vi "ControlProgram6.6_10_updateFFB_3_savefittingoutput_v2.vi"() -> ()   [LabVIEW 2016]
uses:
  <vilib>/Utility/miscctls.llb/LVPoint32TypeDef.ctl
  <vilib>/Platform/TimedLoop/XDataNode/timing_clust.ctl
  <vilib>/Platform/TimedLoop/XDataNode/nitl_modes.ctl
  <vilib>/Platform/TimedLoop/XDataNode/wakeup.ctl
  <vilib>/Instr/_visa.llb/Select Event Type.ctl
  <vilib>/vision/Avi1.llb/AviRefnum.ctl
  <vilib>/Utility/error.llb/DialogType.ctl
  <vilib>/DAQmx/write.llb/DAQmx Write (Analog 1D DBL NChan 1Samp).vi
  <vilib>/DAQmx/read.llb/DAQmx Read (Analog 2D DBL NChan NSamp).vi
  <vilib>/Analysis/baseanly.llb/Mean (DBL).vi
  <vilib>/DAQmx/write.llb/DAQmx Write (Digital Bool 1Line 1Point).vi
  <vilib>/DAQmx/create/channels.llb/DAQmx Create Channel (DO-Digital Output).vi
  <vilib>/DAQmx/create/channels.llb/DAQmx Create Channel (AI-Voltage-Basic).vi
  <vilib>/DAQmx/create/channels.llb/DAQmx Create Channel (AO-Voltage-Basic).vi
  <vilib>/DAQmx/configure/timing.llb/DAQmx Timing (Sample Clock).vi
  <vilib>/DAQmx/miscellaneous.llb/DAQmx Fill In Error Info.vi
  <vilib>/Instr/_visa.llb/VISA Configure Serial Port (Instr).vi
  Arnulf--joystick/git(most_up_to_date)/Logitech-joystick/Old Trap/FAST_Global_var.vi
  <vilib>/Utility/inputDevices.llb/mouseAcquire.vi
  <vilib>/Utility/inputDevices.llb/closeMouse.vi
  <vilib>/platform/TimedLoop/XDataNode/XDataNode.xnode
  <vilib>/Platform/TimedLoop/XDataNode/XDNodeRunTimeDep.lvlib
  <resource>/objmgr/daqmx.rc
  <vilib>/Analysis/NI_AALBase.lvlib
panel:
  out "offset ffb param":T1
  in  "Save file index":i32
  out "Saving Move":bool
  out "Move time":string
  out "Primary Video Display":T2(plugin-control)
  out "Flush Sample Start Time":u32=2111292881
  out "Sample flush time (s)":dbl=48.0
  in  "Inject Sample":bool
  out "Cal values":T3={"AX alpha"=612.9626061060078, "BX alpha"=549.6584469744151, "AX kappa"=0.3485731373010688, "BX kappa"=0.3853424216291352, "AX offset"=-0.03900484438240665, "BX offset"=-0.11295550662085417, "AY alpha"=582.7562541114835, "BY alpha"=571.1587543790358, "AY kappa"=0.37498408087930674, "BY kappa"=0.36252029651198364, "AY offset"=-0.21125584642206058, "BY offset"=-0.12469077200400738}
  in  "Inject Pump 1":bool
  in  "Inject Pump 2":bool
  in  "Tab Control 2":T4(tab)
  in  "Force FB script":bool
  in  "Got ADig bead":bool
  in  "Move Cap. 2 (ADig Top)":bool
  in  "Dump beads":bool
  in  "Got DNA bead":bool
  in  "Flow on\ncap 2?":bool=TRUE
  in  "Flow on\ncap 1?":bool=TRUE
  in  "Flow on\ndump?":bool=TRUE
  in  "Raster set":i32=1
  in  "Fish After TA?":bool=TRUE
  in  "Delta after tether":dbl=1700.0
  in  "TA Cancel Save?":bool=TRUE
  in  "Min fish\ndelta (nm)":dbl=1425.0 min=0.0 max=5000.0 step=50.0
  in  "Max fish\ndelta (nm)":dbl=1900.0 min=0.0 max=5000.0 step=25.0
  in  "Fish Speed (ms)":i32=5000
  in  "Wait (ms)":i32=1500
  in  "# attempts":dbl=10.0
  in  "Cutoff force (pN)":dbl=4.5
  in  "Raster after\n tether?":bool=TRUE
  out "Tether":bool
  out "Attempt #":i32
  in  "Flow on\nwhile fish?":bool=TRUE
  in  "Flow on\nafter raster?":bool=TRUE
  in  "Offset raster set":i32
  in  "Offset @ Delta (nm)":dbl=1700.0
  in  "Cal @ Delta (nm)":dbl=2500.0
  in  "Cal stage position":i32=3
  out "Cal Final Sampling Rate":dbl=125000.0
  in  "Cal Averaging":i32=1
  in  "Wait before dip (s)":dbl=3.0
  in  "Start dipping after?":bool
  in  "Start trap delta (nm)":dbl=1700.0
  in  "Repeat Dip":bool
  out "Dip #":i32
  in  "Dip attempts":dbl=3.0
  in  "Cancel Rep\n Dip":bool
  out "Return elasped time":i32
  in  "Return duration":dbl=15.0
  in  "Cancel dwell":bool=TRUE
  in  "Pause dwell":bool
  in  "Start/Return position":dbl=3.0
  in  "Dip duration":dbl=15.0
  in  "Dip position":dbl=4.0
  in  "Dip":bool
  out "Dip elasped time":i32
  in  "Stop":bool=TRUE
  in  "?":T5(tab)
  out "FAST X-Y":bool
  out "FAST Z":bool
  in  "Cal time (s)":dbl=5.0
  in  "Save N sets":bool
  in  "N sets":i32=200
  out "Cal sets to save":i32=500
  in  "Reset data stream":bool
  out "Buffer Overflow":bool
  out "Stage moving":bool
  in  "Comment":string
  in  "Raster scan":bool
  out "Saving":bool
  in  "Save cal":bool
  in  "Save Data":bool
  in  "Stop saving":bool
  out "Calibrating":bool
  out "Progress":dbl(slide) scale=0.0..100.0
  in  "Read Cal":bool
  in  "Fish":bool
  in  "Averaging Number":i32=1250
  out "Final Sampling Rate":dbl=100.0
  in  "Trap position (V)":cluster{"X":dbl, "Y":dbl}={"X"=3.9042624789680316, "Y"=0.2}
  in  "Trap delta (nm)":dbl=2500.0 min=0.0 max=5000.0 step=50.0
  in  "Fixed X":dbl=1.1
  in  "Fixed Y":dbl=0.15
  in  "Shutter 1 (B)":bool
  in  "Shutter 2 (A)":bool
  in  "Pulling direction":bool
  out "Raster scanning...":bool
  out "Current file name":path=path "D:/data/160111/160111_006.dat"
  in  "AX alpha":dbl=612.9626061060078 format="%#_3p"
  in  "BX alpha":dbl=549.6584469744151 format="%#_3g"
  in  "AX kappa":dbl=0.3485731373010688 format="%#_3g"
  in  "BX kappa":dbl=0.3853424216291352 format="%#_3g"
  in  "AX offset":dbl=-0.03900484438240665 format="%#_3g"
  in  "BX offset":dbl=-0.11295550662085417 format="%#_3g"
  in  "AY alpha":dbl=582.7562541114835 format="%#_3g"
  in  "BY alpha":dbl=571.1587543790358 format="%#_3g"
  in  "AY kappa":dbl=0.37498408087930674 format="%#_3g"
  in  "BY kappa":dbl=0.36252029651198364 format="%#_3g"
  in  "AY offset":dbl=-0.21125584642206058 format="%#_3g"
  in  "BY offset":dbl=-0.12469077200400738 format="%#_3g"
  out "Buffer status":u8(slide) scale=0.0..100.0
  in  "Target":bool
  in  "Default data save Avg Num":i32=1250
  in  "dump spot 2":string="Dump beads spot"
  in  "Move to Position 6":bool
  in  "Set Position 6":bool
  in  "Set Current\nPos to (0,0,0)":bool
  in  "dump spot":string="Dump beads spot"
  in  "up flow spot":string="Upper flow spot"
  in  "low flow spot":string="Lower flow spot"
  in  "up cap":string="Upper capillary (ADig beads)"
  in  "bottom cap":string="Lower capillary (DNA beads)"
  in  "Move to Position 5":bool
  in  "Set Position 5":bool
  in  "Saved stage positions":dbl[][](array[numeric])=[[1.0, 0.0, 0.0, 0.0], [2.0, -0.13716, -3.21132, 0.01436], [3.0, 0.45, -0.73974, 0.005], [4.0, 0.45, -2.1978, 0.005], [5.0, 0.45, -2.63158, -0.02256]]
  in  "Set Position 2":bool
  in  "Move to Position 2":bool
  in  "Set Position 1":bool
  in  "Move to Position 1":bool
  in  "Set Position 4":bool
  in  "Move to Position 4":bool
  in  "Set Position 3":bool
  in  "Move to Position 3":bool
  out "Stage error":errorcluster
  in  "Clear Volume":bool
  out "Sample Flush Meter":u8(slide) scale=0.0..100.0
  out "Flushing Sample":bool
  in  "Flush Sample":bool
  in  "Normal \nRate (ul/hr)  3":dbl=100.0
  in  "Normal \nVolume (ul) 3":dbl=250.0
  in  "Normal \nVolume (ul) 2":dbl
  in  "Normal \nRate (ul/hr)":dbl
  in  "Normal \nVolume (ul)":dbl
  in  "Flush\nRate (ul/min)":dbl
  in  "Flush\nVolume (ul)":dbl
  in  "Flush \nRate (ul/min)  2":dbl
  in  "Flush Pump 2":bool
  in  "Flush\nVolume (ul)  2":dbl
  in  "Flush Pump 1":bool
  in  "Normal \nRate (ul/hr)  2":dbl
  in  "Write Wait":i32=1000
  in  "Flush \nRate (ul/min)  3":dbl=100.0
  in  "Flush\nVolume (ul)  3":dbl=80.0
  out "error out":errorcluster
  in  "Use Mouse to Move Trap?":bool
  in  "Pause Mouse/Mirror Connection":bool
  out "Reference Voltage":cluster{dbl, dbl}={0.0, -0.0}
  out "Saved voltage":cluster{dbl, dbl}={5.766666666666665, 1.45}
  out "Real Coordinates":cluster{"Horizontal":i32, "Vertical":i32}={"Horizontal"=897, "Vertical"=-1271}
  out "CoordinatesMousePressed":T6
  in  "reset offset ffb param":bool
  in  "Read \nOffset FFB param":bool
  in  "Force Feedback 2":bool
  in  "Offset 2":cluster{"Off Y":dbl, "Off X":dbl}={"Off Y"=1.5, "Off X"=0.17}
  in  "Setpoint voltage 2":cluster{"SP Y":dbl, "SP X":dbl}={"SP Y"=0.6, "SP X"=0.0}
  out "Sum error":dbl(knob) scale=-0.2..0.2
  out "Trap sep":waveform(dbl)[](graph)=[{"t0"=timestamp(4.489999999999949 s since 1904-01-01), "dt"=0.002, "Y"=[-1157.7639781743756, -1157.678951177374, -1157.7582331070425, -1157.7490409992681, -1157.8995617642552], "attributes"=variant("NI_ChannelName"=variant(string "T2 X"))}, {"t0"=timestamp(4.489999999999949 s since 1904-01-01), "dt"=0.002, "Y"=[-909.0775466981794, -909.1316439023619, -909.1322956759037, -909.1570630705896, -909.1264297140281], "attributes"=variant("NI_ChannelName"=variant(string "T2 Y"))}]
  in  "Set reading to\nsetpoint 1":bool
  in  "Offset Y (nm)":dbl format="%0.2f"
  in  "Offset X (nm)":dbl format="%0.2f"
  in  "Remove offsets":bool
  in  "Force Feedback 1":bool
  out "Feedback Output \nVoltage 2":cluster{dbl, dbl} {"?" format="%#_4g"; "?" format="%#_4g"}
  in  "Offset 1":cluster{"Off Y":dbl, "Off X":dbl}={"Off Y"=1.5, "Off X"=0.17}
  in  "Setpoint voltage 1":cluster{"SP Y":dbl, "SP X":dbl}={"SP Y"=0.6, "SP X"=0.0}
  in  "Feedback const":T7={"Ki_B_Y"=0.5, "Ki_B_X"=0.0, "Kp Y"=1.0, "Kp X"=0.0}
  out "Mean Trap Pos X 2 (nm)":dbl=-1157.769953044463 format="%0.2f"
  out "Mean Trp Pos Y 2 (nm)":dbl=-909.1249958122125 format="%0.2f"
  out "T2 X RMS (A)":dbl=0.7168002469275427 format="%0.2f"
  out "T2 Y RMS (A)":dbl=0.25997187037503383 format="%0.2f"
  in  "Set reading to\nsetpoint 2":bool
  out "offset fit ffb output":cluster{dbl, dbl} {"?" format="%#_4g"; "?" format="%#_4g"}
  in  "Scan range (nm)":dbl=425.0
  in  "Scan speed (nm/s)":dbl=100.0 min=0.0 max=100.0
  in  "Step size (nm)":dbl=1.0
  in  "Save scans":bool=TRUE
  in  "# scans":i32=1
  in  "Load param":bool
  in  "Scan Parameters":T8(array[cluster])
  in  "Trap delta\nafter (nm)":dbl=1550.0
  in  "Stop raster":bool
  out "Scan range (V)":dbl=0.47672462142456534
  out "Scan steps (mirror)":u64=425
  out "Scan increment (V)":dbl=0.0011217049915872126
  out "Time per step (ms)":dbl=10.0
  out "Total raster time (s)":dbl=8.5
  out "N sets to be saved":dbl=850.0
  out "moveX":string
  out "moveY":string
  in  "Grid Movable Trap":bool
  in  "take fixed bead\n Images":bool
  in  "Zoom Factor":sgl=7.0
  in  "Center Point":cluster{"X":i32, "Y":i32}={"X"=335, "Y"=271}
  in  "Intensity Upper":dbl=88.0
  in  "Intensity Lower":dbl=66.0
  out "Window Size":cluster{"Height":i32, "Width":i32}
  in  "Image Index":dbl=1.0 min=1.0
  in  "Save Image":bool
  in  "Averaging":bool
  in  "Reset Averaging":bool
  in  "Save Video":bool
  in  "New Video File":bool
  in  "Video Index":dbl=1.0 min=1.0 step=1.0
  in  "Video Capture Rate (Hz)":dbl=30.0
  in  "Initial Window Size":cluster{"Width":i32, "Height":i32}={"Width"=884, "Height"=619}
  in  "Initial Window Position":cluster{"X Position":i32, "Y Position":i32}={"X Position"=796, "Y Position"=4}
  out "Window Position":cluster{"X Position":i32, "Y Position":i32}={"X Position"=40, "Y Position"=40}
  out "Path Out":path
  in  "Target coordinates":cluster{"X1":dbl, "Y1":dbl, "X2":dbl, "Y2":dbl}={"X1"=328.0, "Y1"=274.0, "X2"=368.0, "Y2"=314.0}
  out "image8bitArray":u8[][](array[numeric])
  out "GreyscaleArray":u32[](array[numeric])
  in  "take background images":bool
  in  "# Samples/channel (in)":i32=40000 format="%.2f"
  out "Buffer size\n(Samples/channel)":u32=511
  out "DAQ rate\n(Samples/s)":dbl=125000.0 format="%#_6p"
  out "# Samples/channel":i32=1250
  out "# Samples/channel/s":dbl=100.0
  out "AvailSampPerChan":u32=9
  out "Data update period (s/set)":dbl=0.01 format="%#_6p"
  out "AvailSampPerChan 2":u32=110
  in  "PC samp per channel":i32=1000
  in  "Sampling Rate":dbl=125000.0 format="%0.0p"
  in  "DAQ Rate2":dbl=1000000.0 format="%#_6p"
  out "Data period (s)":dbl=8e-06 format="%#_6p"
  in  "Save user params":bool
  in  "User":string(combo)
  in  "Load user params":bool
  in  "Tether break\nforce (pN)":dbl=1.0
  in  "Path":path=path "E:/Data"
  out "Mirror task":refnum<k21>
  in  "Conv X (nm/V)":dbl=891.5
  in  "Conv Y (nm/V)":dbl=505.7
  in  "Min value Y":dbl format="%.1g"
  in  "Max value Y":dbl=10.0 format="%.1f"
  in  "Min value X":dbl format="%0.1f"
  in  "Max value X":dbl=10.0 format="%.1f"
  in  "HWP1":string="Half waveplate 1: differential trap power"
  in  "HWP0":string="Half waveplate 0: total trap power"
  in  "Move 1":bool
  in  "\"Degrees\" 1":dbl
  in  "Move 0":bool
  in  "\"Degrees\" 0":dbl
  in  "Y command":enum16{"Fish", "Dump", "Got ADig", "Got DNA"}(ring)
  in  "B command":enum16{"Got DNA", "Got ADig", "Dump", "Fish"}(ring)
  in  "A command":enum16{"Got ADig", "Dump", "Fish", "Got DNA"}(ring)
  in  "X command":enum16{"Dump", "Fish", "Got ADig", "Got DNA"}(ring)
  out "Logitech":bool
  out "START":bool
  out "BACK":bool
  out "Right stick button":bool
  out "Left Y":i8(slide) scale=-128.0..127.0
  out "Left X":i8(slide) scale=-128.0..127.0
  out "Right Y":i8(slide) scale=-128.0..127.0
  out "Right X":i8(slide) scale=-128.0..127.0
  out "X":bool
  out "Y":bool
  out "A":bool
  out "B":bool
  out "RB":bool
  out "LB":bool
  out "R":bool
  out "L":bool
  out "D":bool
  out "U":bool
  out "Left stick button":bool
  out "FAST Z":bool
  out "FAST X-Y":bool
  in  "XY Speed Definitions":T9={"Slow X velocity input"="0.05", "Slow Y velocity input"="0.05", "Fast1 X velocity input"="0.1", "Fast1 Y velocity input"="0.1", "Fast2 X velocity input"="0.2", "Fast2 Y velocity input"="0.2"}
  in  "Z Speed Definitions":cluster{"Slow Z":string, "Fast Z":string}={"Slow Z"="0.025", "Fast Z"="0.05"}
  in  "Z Wait time":string="120"
  in  "X-Y Wait time":string="125"
  in  "USB port":refnum<visa-resource-name>="USB0::0x046D::0xC21D::CC66247B::RAW"
  out "Deflection":T6
  in  "Sampling Rate":dbl=125000.0 format="%0.2f"
  in  "Averaging Number":i32=12500
  in  "DAQ Rate":dbl=1000000.0
  out "Final Sampling Rate":dbl
  in  "Tab Control":T10(tab)
  in  "Downsamp\nfact":dbl=250.0
  out "Bead sep":waveform(dbl)[](graph)=[{"t0"=timestamp(4.489999999999949 s since 1904-01-01), "dt"=0.002, "Y"=[8093.963535945606, 8103.1617772716045, 8385.72390184118, 8245.733099167523, 8154.925676756515], "attributes"=variant("NI_ChannelName"=variant(string "T2"))}, {"t0"=timestamp(4.489999999999949 s since 1904-01-01), "dt"=0.002, "Y"=[1717.924930434114, 1628.723007842151, 1787.6888378897193, 1598.475730715916, 1776.2517588078954], "attributes"=variant("NI_ChannelName"=variant(string "T1"))}]
  out "Force (pN)":waveform(dbl)[](graph)=[{"t0"=timestamp(4.489999999999949 s since 1904-01-01), "dt"=0.002, "Y"=[2821.5994183803123, 2824.8226375853515, 2923.3663028678166, 2874.5254578927593, 2842.869034836209], "attributes"=variant("NI_ChannelName"=variant(string "T2"))}, {"t0"=timestamp(4.489999999999949 s since 1904-01-01), "dt"=0.002, "Y"=[623.5850847499229, 591.0680427774053, 648.761979867749, 579.944408346982, 644.7436619059413], "attributes"=variant("NI_ChannelName"=variant(string "T1"))}]
  out "Mean force (pN)":dbl=1737.5286029210451 format="%0.2f"
  out "Force noise (pN)":dbl=26.83032703631318 format="%0.2f"
  out "Mean Bead Sep\n(nm)":dbl=4949.257225667222 format="%0.2f"
  out "Bead Sep Noise\n(A)":dbl=757.8078481959694 format="%0.2f"
  out "PSD 2":cluster{dbl[], dbl[]}(graph)
  out "PSD 1":cluster{dbl[], dbl[]}(graph)
  out "PSD 1 Sum":dbl(slide) scale=0.0..10.0
  out "PSD 2 Sum":dbl(slide) scale=0.0..10.0
  in  "Start":bool
  out "All signals 2":waveform(dbl)[](graph)=[{"t0"=timestamp(4.489999999999949 s since 1904-01-01), "dt"=0.002, "Y"=[0.0010396217068286443, 0.0010666908927528754, 0.001103298744846499, 0.0010651440823993424, 0.0010656596859401936], "attributes"=variant("NI_ChannelName"=variant(string "A y"))}, {"t0"=timestamp(4.489999999999949 s since 1904-01-01), "dt"=0.002, "Y"=[0.02000680227246931, 0.020097032918054827, 0.02003412926844257, 0.020136734401221615, 0.020087494249822452], "attributes"=variant("NI_ChannelName"=variant(string "A x"))}, {"t0"=timestamp(4.489999999999949 s since 1904-01-01), "dt"=0.002, "Y"=[-0.0014958587831537804, -0.0015046240440107857, -0.0014930229638311983, -0.001533240041751485, -0.0015262793936602433], "attributes"=variant("NI_ChannelName"=variant(string "B y"))}, {"t0"=timestamp(4.489999999999949 s since 1904-01-01), "dt"=0.002, "Y"=[0.0002901198559372817, 0.0002731049385577592, 0.00026511308349727467, 0.0002517073909711183, 0.0002916666665966012], "attributes"=variant("NI_ChannelName"=variant(string "B x"))}, {"t0"=timestamp(4.489999999999949 s since 1904-01-01), "dt"=0.002, "Y"=[-0.001511556786147372, -0.0015167122027053212, -0.0014612914746018214, -0.0014935128282145193, -0.0015064013696263116], "attributes"=variant("NI_ChannelName"=variant(string "A sum"))}, {"t0"=timestamp(4.489999999999949 s since 1904-01-01), "dt"=0.002, "Y"=[-0.0005242945138364382, -0.0005565158674093218, -0.000501095139248956, -0.0005771375336978897, -0.0005165613890095197], "attributes"=variant("NI_ChannelName"=variant(string "B sum"))}, {"t0"=timestamp(4.489999999999949 s since 1904-01-01), "dt"=0.002, "Y"=[0.0013303666019343777, 0.0014257418088905328, 0.0013368108726387405, 0.0013471217058124534, 0.0011782818123890176], "attributes"=variant("NI_ChannelName"=variant(string "Trap x"))}, {"t0"=timestamp(4.489999999999949 s since 1904-01-01), "dt"=0.002, "Y"=[0.0023382505474007294, 0.002231275652833831, 0.002229986798687363, 0.0021810103409340116, 0.002241586486003531], "attributes"=variant("NI_ChannelName"=variant(string "Trap y"))}]
  out "All signals":waveform(dbl)[](graph)=[{"t0"=timestamp(4.489999999999949 s since 1904-01-01), "dt"=0.002, "Y"=[0.0010396217068286443, 0.0010666908927528754, 0.001103298744846499, 0.0010651440823993424, 0.0010656596859401936], "attributes"=variant("NI_ChannelName"=variant(string "A y"))}, {"t0"=timestamp(4.489999999999949 s since 1904-01-01), "dt"=0.002, "Y"=[0.02000680227246931, 0.020097032918054827, 0.02003412926844257, 0.020136734401221615, 0.020087494249822452], "attributes"=variant("NI_ChannelName"=variant(string "A x"))}, {"t0"=timestamp(4.489999999999949 s since 1904-01-01), "dt"=0.002, "Y"=[-0.0014958587831537804, -0.0015046240440107857, -0.0014930229638311983, -0.001533240041751485, -0.0015262793936602433], "attributes"=variant("NI_ChannelName"=variant(string "B y"))}, {"t0"=timestamp(4.489999999999949 s since 1904-01-01), "dt"=0.002, "Y"=[0.0002901198559372817, 0.0002731049385577592, 0.00026511308349727467, 0.0002517073909711183, 0.0002916666665966012], "attributes"=variant("NI_ChannelName"=variant(string "B x"))}, {"t0"=timestamp(4.489999999999949 s since 1904-01-01), "dt"=0.002, "Y"=[-0.001511556786147372, -0.0015167122027053212, -0.0014612914746018214, -0.0014935128282145193, -0.0015064013696263116], "attributes"=variant("NI_ChannelName"=variant(string "A sum"))}, {"t0"=timestamp(4.489999999999949 s since 1904-01-01), "dt"=0.002, "Y"=[-0.0005242945138364382, -0.0005565158674093218, -0.000501095139248956, -0.0005771375336978897, -0.0005165613890095197], "attributes"=variant("NI_ChannelName"=variant(string "B sum"))}, {"t0"=timestamp(4.489999999999949 s since 1904-01-01), "dt"=0.002, "Y"=[0.0013303666019343777, 0.0014257418088905328, 0.0013368108726387405, 0.0013471217058124534, 0.0011782818123890176], "attributes"=variant("NI_ChannelName"=variant(string "Trap x"))}, {"t0"=timestamp(4.489999999999949 s since 1904-01-01), "dt"=0.002, "Y"=[0.0023382505474007294, 0.002231275652833831, 0.002229986798687363, 0.0021810103409340116, 0.002241586486003531], "attributes"=variant("NI_ChannelName"=variant(string "Trap y"))}]
  out "Chart Freq (Hz)":dbl=500.0
  # "Bead Calibration"
  # "Y"
  # "X"
  # "Pump #1 Controls"
  # "Pump #2 Controls"
  # "Sample Pump Controls"
  # "Retract the pumps manually. Change it back to INFUSE when you're done. Suck it up, don't whine."
  # "Shutter 1 (B)"
  # "Move to Lower Cap"
  # "Inject Sample"
  # "Move to Upper Cap"
  # "Shutter 2 (A)"
  # "Select the Joystick input:"
  # "Overflow happens when >40 commands\nsent in 5 seconds. Then 4 consecutive beeps."
  # "Try increasing wait time to reduce 'following error threshold exceeded' occurances."
  # "Left stick controls Z axis.\nRight on stick: neg Z-dir\nUp on stick: neg Z-dir"
  # "Toggles FAST Z"
  # "Toggles FAST X-Y"
  # "The default Newport max velocity is 0.4"
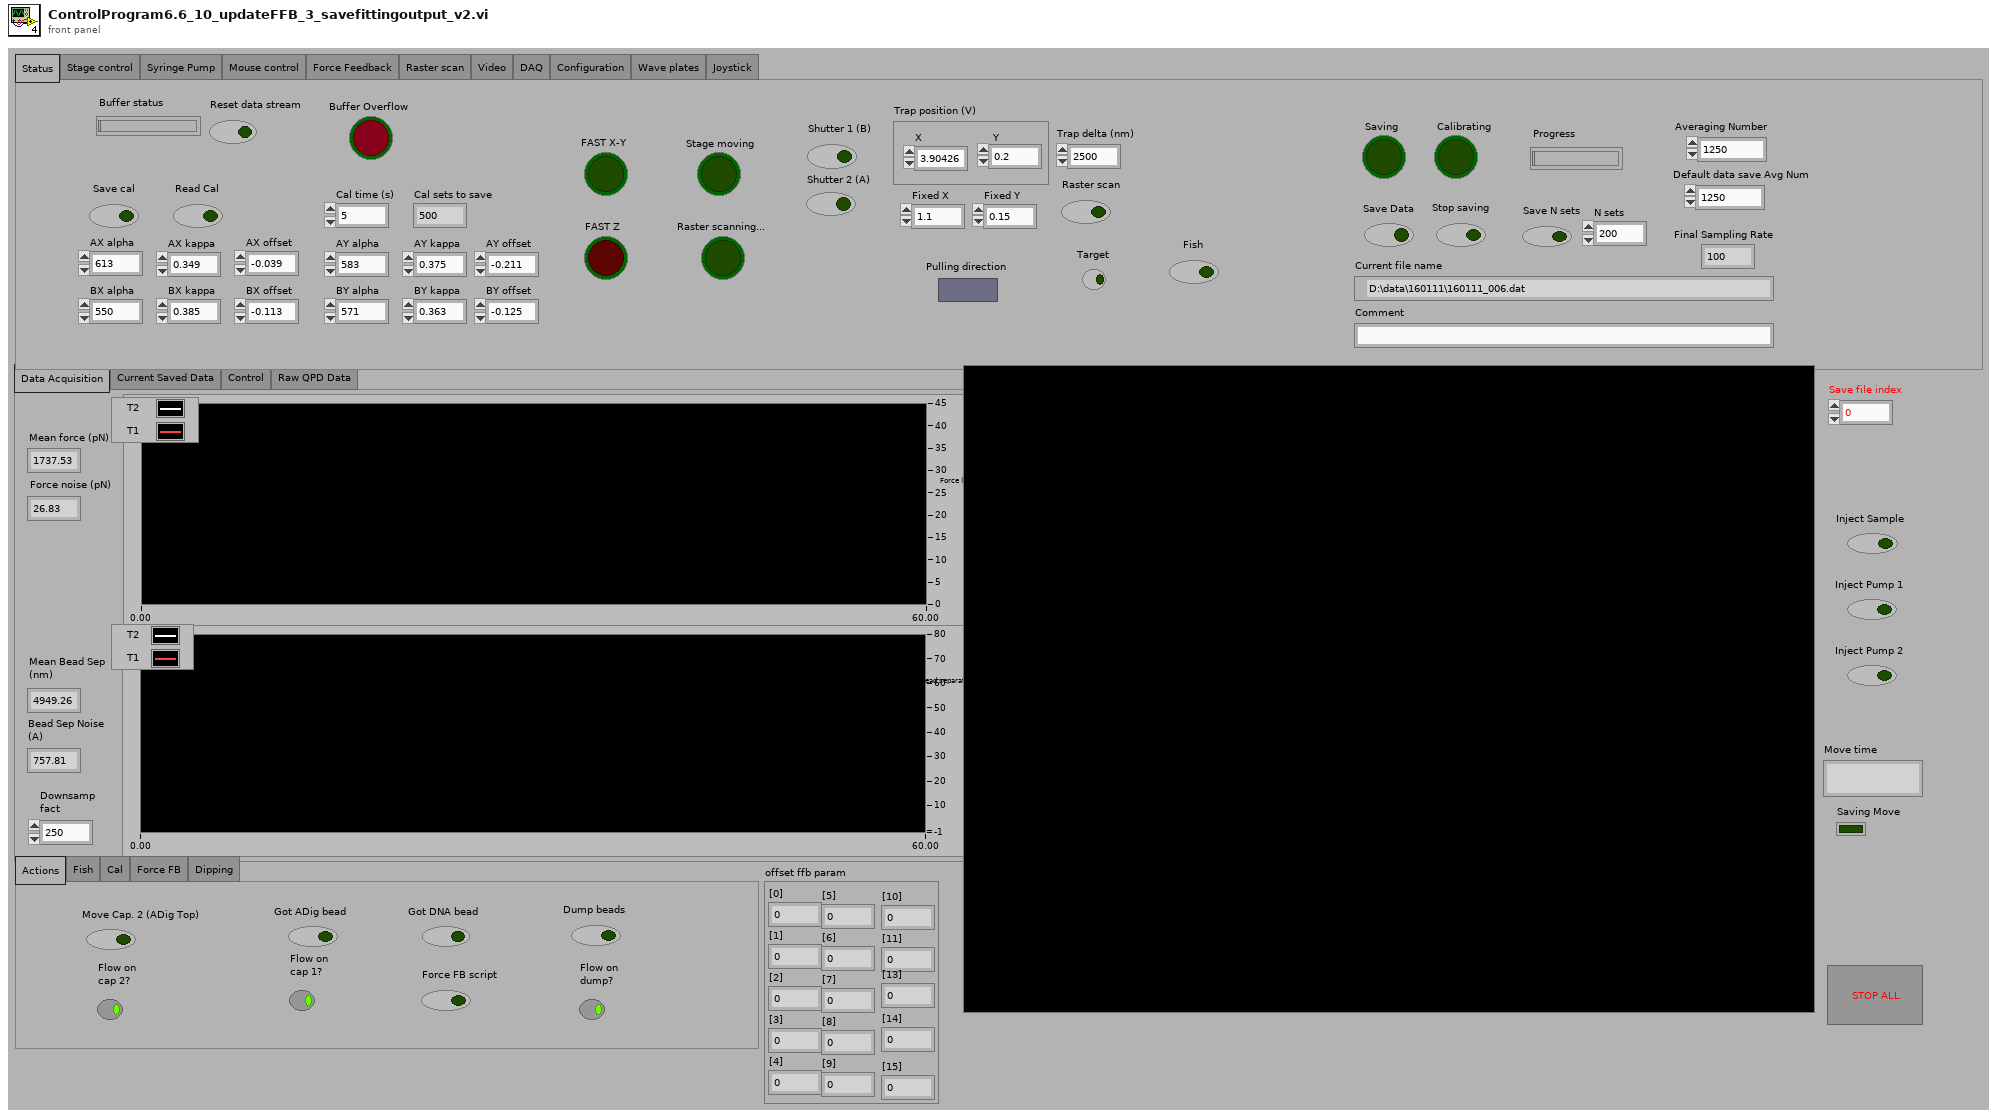
[diagram p1: front panel]
types:
  T1 = cluster{"[0]":dbl, "[1]":dbl, "[2]":dbl, "[3]":dbl, "[4]":dbl, "[5]":dbl, "[6]":dbl, "[7]":dbl, "[8]":dbl, "[9]":dbl, "[10]":dbl, "[11]":dbl, "[13]":dbl, "[14]":dbl, "[15]":dbl}
  T2 = typedef "IMAQ Image.ctl" = refnum<image>
  T3 = cluster{"AX alpha":dbl, "BX alpha":dbl, "AX kappa":dbl, "BX kappa":dbl, "AX offset":dbl, "BX offset":dbl, "AY alpha":dbl, "BY alpha":dbl, "AY kappa":dbl, "BY kappa":dbl, "AY offset":dbl, "BY offset":dbl}
  T4 = enum32{"Actions", "Fish", "Cal", "Force FB", "Dipping"}
  T5 = enum32{"Status", "Stage control", "Syringe Pump", "Mouse control", "Force Feedback", "Raster scan", "Video", "DAQ", "Configuration", "Wave plates", "Joystick"}
  T6 = typedef "LVPoint32TypeDef.ctl" = cluster{"Horizontal":i32, "Vertical":i32}
  T7 = cluster{"Ki_B_Y":dbl, "Ki_B_X":dbl, "Kp Y":dbl, "Kp X":dbl}
  T8 = cluster{"Label":string, "Scan range 1":dbl, "Step size 1":dbl, "Scan speed 1":i32, "# scans 2":i32}[]
  T9 = cluster{"Slow X velocity input":string, "Slow Y velocity input":string, "Fast1 X velocity input":string, "Fast1 Y velocity input":string, "Fast2 X velocity input":string, "Fast2 Y velocity input":string}
  T10 = enum32{"Data Acquisition", "Current Saved Data", "Control", "Raw QPD Data"}
  T11 = typedef "Select Event Type.ctl" = u32
  T12 = enum32{"setting", "request", "request control", "info", "statistics", "system settings", "I/O sub system", "HRT control", "camera descriptions", "device specific data", "event sub system settings", "event sub system results", "image memory manager"}
  T13 = typedef "AviRefnum.ctl" = refnum<k1>
  T14 = typedef "XDNodeRunTimeDep.lvlib/timing_clust.ctl" = cluster{"Expected End [f-1]":u64, "Actual End [f-1]":u64, "Finished Late? [f-1]":bool, "Expected End [i-1]":u64, "Actual End [i-1]":u64, "Finished Late? [i-1]":bool, "Expected Start [i]":u64, "Actual Start [i]":u64, "Expected Start [f]":u64, "Actual Start [f]":u64, "Source Name":string, "Structure Name":string, "Period":i64, "Deadline":i64, "Offset":i64, "Start":i64, "Priority":i32, "Timeout":i32, "Mode":T15, "Wakeup Reason":T16, "Error":errorcluster, "Source Type":string, "Secondary Source Type":string, "Global End Time":u64, "Global Start Time":u64, "Frame Duration":u64, "Iteration Duration":u64, "Assigned CPU":i32, "I/O Scan Engine Mode":u32}
  T15 = typedef "XDNodeRunTimeDep.lvlib/nitl_modes.ctl" = enum32{"No Change", "Process missed periods, maintain original phase", "Discard missed periods, maintain original phase", "Process missed periods, ignore original phase", "Discard missed periods, ignore original phase"}
  T16 = typedef "XDNodeRunTimeDep.lvlib/wakeup.ctl" = enum32{"Normal", "Aborted", "Asynchronous wakeup", "Timing source error", "Timed loop error", "Timeout"}
  T17 = typedef "Image Type" = u32
  T18 = typedef "imagedata.ctl" = cluster{"image type":i32, "image depth":i32, "image":u8[], "mask":u8[], "colors":u32[], "Rectangle":cluster{"left":i16, "top":i16, "right":i16, "bottom":i16}}
  T19 = enum16{"open", "replace", "create", "open or create", "replace or create", "replace or create with confirmation"}
  T20 = enum16{"big-endian, network order", "native, host order", "little-endian"}
  T21 = cluster{string, string, string, string, string, string, string, string}
  T22 = cluster{"LB":bool, "RB":bool, "BACK":bool, "Logitech":bool, "START":bool}
  T23 = cluster{"Right X":i8, "Right Y":i8, "Left X":i8, "Left Y":i8}
  T24 = enum32{"Status", "Stage control", "Syringe Pump", "Mouse control", "Force Feedback", "Raster scan", "Video", "DAQ", "Configuration", "Wave plates"}
  T25 = typedef "DialogType.ctl" = u16
  T26 = cluster{"button 1":bool, "button 2":bool, "button 3":bool, "button 4":bool}
  T27 = cluster{"[0]":dbl, "[1]":dbl, "[2]":dbl, "[3]":dbl, "[4]":dbl, "[5]":dbl, "[6]":dbl, "[7]":dbl, "[8]":dbl, "[9]":dbl, "[10]":dbl, "[11]":dbl}
  T28 = cluster{"[0]":dbl, "[1]":dbl, "[2]":dbl, "[3]":dbl, "[4]":dbl, "[5]":dbl, "[6]":dbl, "[7]":dbl, "[8]":dbl, "[9]":dbl, "[10]":dbl, "[11]":dbl, "[12]":dbl, "[13]":dbl, "[14]":dbl}
  T29 = cluster{"array[0]":dbl, "array[1]":dbl, "array[2]":dbl, "array[3]":dbl, "array[4]":dbl, "array[5]":dbl, "array[6]":dbl, "array[7]":dbl, "array[8]":dbl, "array[9]":dbl, "array[10]":dbl, "array[11]":dbl, "array[12]":dbl, "array[13]":dbl, "array[14]":dbl}
  T30 = cluster{"Label":string, "Scan range 1":dbl, "Step size 1":dbl, "Scan speed 1":i32, "# scans 2":i32}
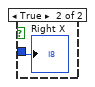
[diagram p5: hidden frame]
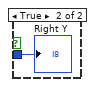
[diagram p6: hidden frame]
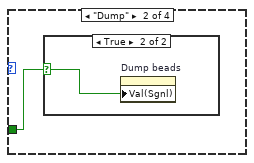
[diagram p10: hidden frame]
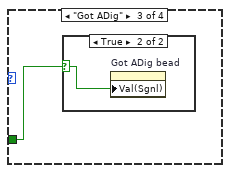
[diagram p12: hidden frame]
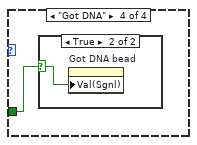
[diagram p14: hidden frame]
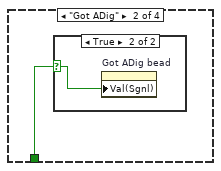
[diagram p17: hidden frame]
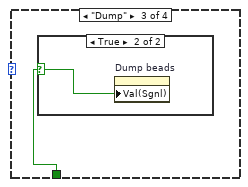
[diagram p19: hidden frame]
diagram:
  w10 = T11 1073684535 items=["Service Request"=1073684491, "Trigger"=3221168138, "Clear"=1073684493, "VXI Signal"=1073684512, "VXI/VME Interrupt"=3221168161, "VXI/VME Sysfail"=1073684509, "VXI/VME Sysreset"=1073684510, "GPIB CIC"=1073684498, "GPIB Talk"=1073684499, "GPIB Listen"=1073684500, "PXI Interrupt"=1073684514, "Serial Break"=1073684515, "Serial TermChar"=1073684516, "Serial CTS"=1073684521, "Serial DSR"=1073684522, "Serial DCD"=1073684524, "Serial RI"=1073684526, "Serial Character"=1073684533, "USB Interrupt"=1073684535, "All Enabled"=1073709055] ("Event Type")
  w49 = 10.0 ("Minimum Value")
  w50 = -10.0 ("Minimum Value")
  w52 = -2.0 ("Minimum Value")
  w53 = 2.0 ("Maximum Value")
  w78 = 10123 items=["Finite Samples"=10178, "Continuous Samples"=10123] ("sample mode")
  w98 = tag "Dev1/port2/line1"  # Shutter 2
  w101 = tag "Dev1/port1/line4"  # Shutter 1
  # "Open the RAW resource"
  # "Enable USB Interrupt Event"
  # "Create channels for movable mirror"
  # "Create channels for detectors"
  n1 = call-poly <vilib>:"DAQmx Create Virtual Channel.vi"("maximum value"=w53, "minimum value"=w52, "physical channels"=tag "Dev1/ai0" ("Physical Channel")) -> ("task out"=w54:refnum<k21>, "error out"=w77:errorcluster)  [unwired: 11 in]
  n2 = call-poly <vilib>:"DAQmx Create Virtual Channel.vi"("task in"=w54, "maximum value"=w53, "minimum value"=w52, "physical channels"=tag "Dev1/ai1", "error in"=w77) -> ("task out"=w75:refnum<k21>, "error out"=w74:errorcluster)  [unwired: 9 in]
  n3 = call-poly <vilib>:"DAQmx Create Virtual Channel.vi"("task in"=w75, "maximum value"=w53, "minimum value"=w52, "physical channels"=tag "Dev1/ai2", "error in"=w74) -> ("task out"=w66:refnum<k21>, "error out"=w65:errorcluster)  [unwired: 9 in]
  n4 = call-poly <vilib>:"DAQmx Create Virtual Channel.vi"("task in"=w66, "maximum value"=w53, "minimum value"=w52, "physical channels"=tag "Dev1/ai3" ("Physical Channel"), "error in"=w65) -> ("task out"=w51:refnum<k21>, "error out"=w71:errorcluster)  [unwired: 9 in]
  n5 = call-poly <vilib>:"DAQmx Create Virtual Channel.vi"("task in"=w51, "maximum value"=w49, "minimum value"=w50, "physical channels"=tag "Dev1/ai4", "error in"=w71) -> ("task out"=w69:refnum<k21>, "error out"=w68:errorcluster)  [unwired: 9 in]
  n6 = call-poly <vilib>:"DAQmx Create Virtual Channel.vi"("task in"=w69, "maximum value"=w49, "minimum value"=w50, "physical channels"=tag "Dev1/ai5", "error in"=w68) -> ("task out"=w64:refnum<k21>, "error out"=w63:errorcluster)  [unwired: 9 in]
  n7 = call-poly <vilib>:"DAQmx Create Virtual Channel.vi"("task in"=w64, "maximum value"=w49, "minimum value"=w50, "physical channels"=tag "Dev1/ai6", "error in"=w63) -> ("task out"=w58:refnum<k21>, "error out"=w56:errorcluster)  [unwired: 9 in]
  n8 = call-poly <vilib>:"DAQmx Create Virtual Channel.vi"("task in"=w58, "maximum value"=w49, "minimum value"=w50, "physical channels"=tag "Dev1/ai7", "error in"=w56) -> ("task out"=w57:refnum<k21>, "error out"=w55:errorcluster)  [unwired: 9 in]
  n9 = call-poly <vilib>:"DAQmx Timing.vi"("task/channels in"=w57, "sample mode"=w78, "samples per channel"="PC samp per channel", "rate"="Sampling Rate", "error in"=w55) -> ("task out"=w61:refnum<k21>, "error out"=w60:errorcluster)  [unwired: 9 in]
  n10 = call-poly <vilib>:"DAQmx Create Virtual Channel.vi"("maximum value"="Max value Y", "minimum value"="Min value Y", "physical channels"=tag "Dev1/ao1" ("Trap X Axis")) -> ("task out"=w46:refnum<k21>, "error out"=w48:errorcluster)  [unwired: 11 in]
  n11 = property class="DAQmx Timing"(reference=w61, error in=w60, "More:AI Convert:Rate"="DAQ Rate2") -> (reference out=w19:refnum<k21>, error out=w18:errorcluster, "SampClk.Rate"=→"DAQ rate\n(Samples/s)":dbl)
  n12 = call-poly <vilib>:"DAQmx Create Virtual Channel.vi"("task in"=w46, "maximum value"="Max value X", "minimum value"="Min value X", "physical channels"=tag "Dev1/ao0" ("Trap Y Axis"), "error in"=w48) -> ("task out"=w37:refnum<k21>, "error out"=w36:errorcluster)  [unwired: 9 in]
  "Mirror task" <- w37
  n13 = property class="DAQmx Buffer"(reference=w19, error in=w18) -> (reference out=w16:refnum<k21>, error out=w15:errorcluster, "Input.OnbrdBufSize"=→"Buffer size\n(Samples/channel)":u32)
  n14 = call <vilib>:"DAQmx Start Task.vi"("task/channels in"=w16, "error in"=w15) -> ("task out"=w38:refnum<k21>)  [unwired: 12 in, 1 out]
  n15 = flat-sequence "Video" {
    tunnel: [w114] -> w13
    tunnel: w13 -> [w155]
    frame #0 {
      n16 = while {
        stop <- w107 continue-if-true
        n17 = call "Close Video Capture.vi"() -> ("error code OUT"=w109:i32)
        n18 = Equal?(x=w109, y=0) -> (x = y?=w107:bool)
      }
      n19 = local write "Stop"(FALSE ("Stop All")) -> ()
    }
    frame #1 {
      n20 = call "DMR_Init.vi"() -> ()  [unwired: 3 out]
    }
    frame #2 {
      # "Setting the destination format to Mono8 makes sure that the image can be displayed in the intensity plot."
      n21 = call "DMR_GetDevice.vi"("search string IN"="DE514724602") -> ("device handle OUT"=w132:i32)  [unwired: 4 in, 2 out]
      n22 = call "DMR_OpenDevice.vi"("device handle IN"=w132) -> ("driver handle OUT"=w115:i32)  [unwired: 4 out]
      n23 = call "DMR_FindList.vi"("flags IN"=u32 0 ("flags"), "list name IN"="" ("String"), "list type IN"=T12."camera descriptions", "driver handle IN"=w115) -> ("list handle OUT"=w118:i32)  [unwired: 2 out]
      n24 = call "DMR_FindList.vi"("flags IN"=u32 0 ("flags"), "list name IN"="Base", "list type IN"=T12."setting", "driver handle IN"=w115) -> ("list handle OUT"=w116:i32)  [unwired: 2 out]
      n25 = call "OBJ_GetHandle.vi"("object name IN"="VideoStandard", "list handle IN"=w118) -> ("object handle OUT"=w112:i32)  [unwired: 3 out]
      n26 = call "OBJ_GetHandle.vi"("object name IN"="PixelFormat", "list handle IN"=w116) -> ("object handle OUT"=w126:i32)  [unwired: 3 out]
      n27 = call "OBJ_SetS.vi"("value index IN"=0, "value IN"="NTSC M", "object handle IN"=w112) -> ()  [unwired: 2 out]
      n28 = call "OBJ_SetS.vi"("value index IN"=0, "value IN"="Mono8" ("value"), "object handle IN"=w126) -> ()  [unwired: 2 out]
      n29 = call "OBJ_GetHandle.vi"("object name IN"="VideoChannel", "list handle IN"=w116) -> ("object handle OUT"=w122:i32)  [unwired: 3 out]
      n30 = while {
        tunnel: [w137] -> w114
        tunnel: w115 -> [w134]
        stop <- w135 continue-if-true
        n31 = call "DMR_ImageRequestSingle.vi"("request control IN"=0, "driver handle IN"=w134) -> ("error code OUT"=w136:i32, "driver handle OUT"=w137:i32)  [unwired: 2 out]
        n32 = Equal To 0?(x=w136) -> (x = 0?=w135:bool)
      }
      n33 = call "OBJ_SetI.vi"("value index IN"=0, "value IN"=0 ("Video channel"), "object handle IN"=w122) -> ()  [unwired: 2 out]
    }
    frame #3 {
      w143 = T17 0 items=["Grayscale (U8)", "Grayscale (I16)", "Grayscale (SGL)", "Complex (CSG)", "RGB (U32)", "HSL (U32)", "RGB (U64)"] ("Image Type")
      w151 = T17 0 items=["Grayscale (U8)", "Grayscale (I16)", "Grayscale (SGL)", "Complex (CSG)", "RGB (U32)", "HSL (U32)", "RGB (U64)"] ("Image Type")
      n34 = for "Create Greyscale map" {
        N: 256 -> [_]
        tunnel: [w157] -> w140 mode=indexing
        workers-P: _ -> [_]
        i -> [w160]
        n35 = To Unsigned Byte Integer(number=w160) -> (unsigned 8bit integer=w156:u8)
        n36 = Join Numbers(hi=w156, lo=w156) -> ((hi.lo)=w159:u16)
        n37 = Join Numbers(hi=w156, lo=w156) -> ((hi.lo)=w158:u16)
        n38 = Join Numbers(hi=w159, lo=w158) -> ((hi.lo)=w157:u32)
      }
      n39 = call "IMAQ Create"("Image Name"="Scaled video", "Image Type"=w143) -> ("New Image"=w142:T2)  [unwired: 2 in, 2 out]
      n40 = call "IMAQ Create"("Image Name"="Main video", "Image Type"=w151) -> ("New Image"=w152:T2)  [unwired: 2 in, 2 out]
      n41 = node-c288(0 ("Processor")) -> (w150:T14)  [unwired: 3 out]
      n42 = Initialize Array(u32 0 ("Window Number (0...15)"), 480 ("dimension size"), 640 ("dimension size")) -> (w145:u32[][])
      n43 = timed-loop {
        tunnel: w155 -> [w177]
        tunnel: [w176] -> w154
        tunnel: w152 -> [w175]
        timing: w150 -> [_]
        timing-out: [_] -> w149
        tunnel: w145 -> [w164]
        tunnel: w142 -> [w162]
        tunnel: w140 -> [w161]
        stop <- w163 stop-if-true
        # "This block performs the \nactual image capture."
        n44 = node-c288() -> ()  [unwired: 2 out]
        n45 = local read "Stop"() -> (w163:bool)
        n46 = Reciprocal(x="Video Capture Rate (Hz)") -> (1/x=w167:dbl)
        n47 = Multiply(x=w167, y=1000.0) -> (x*y=w165:dbl)
        n48 = call "DMR_ImageRequestWaitFor.vi"("queue number IN"=0, "timeout(ms) IN"=500, "driver handle IN"=w177) -> ("error code OUT"=w181:i32, "request number OUT"=w178:i32, "driver handle OUT"=w179:i32)
        n49 = feedback #1(T13 refnum ("Avi Refnum")) -> (w169:T13)
        n50 = case shown="True" "New Video File" {
          tunnel: [T13 refnum ("Avi Refnum") w198] -> w171
          tunnel: [FALSE TRUE] -> w172
          tunnel: w169 -> [_ w194]
          frame False {
          }
          frame True {
            n51 = call "Create new save file.vi"("Ext"=".avi" ("string"), "Index In"="Video Index") -> ("Path Out"=w190:path, "Index Out"=w191:dbl)  [unwired: 1 in]
            "Path Out" <- w190
            n52 = Not Equal?(x=w194, y=T13 refnum ("Avi Refnum")) -> (x != y?=w195:bool)
            n53 = Increment(x=w191) -> (x+1=w200:dbl)
            n54 = case shown="True" w195 {
              tunnel: w194 -> [_ w201]
              frame False {
              }
              frame True {
                n55 = call "IMAQ AVI Close"("Avi Refnum"=w201) -> ()  [unwired: 1 in, 10 out]
              }
            }
            n56 = local write "Video Index"(w200) -> ()
            n57 = call "IMAQ AVI Create"("Frames Per Second"=u32 30, "AVI Path"=w190) -> ("Avi Refnum"=w198:T13)  [unwired: 5 in, 4 out]
          }
        }
        n58 = Equal To 0?(x=w181) -> (x = 0?=w180:bool)
        n59 = Select(t=w171, s=w172, f=w169) -> (s? t:f=w170:T13)
        n60 = feedback-in #1(w170) -> ()
        n61 = case shown="True" w180 {
          tunnel: w179 -> [w202 w231]
          tunnel: w178 -> [_ w230]
          tunnel: [w202 w227] -> w176
          tunnel: w175 -> [_ w210]
          tunnel: w164 -> [_ w215]
          tunnel: w170 -> [_ w213]
          tunnel: w162 -> [_ w211]
          tunnel: w161 -> [_ w204]
          frame False {
          }
          frame True {
            w221 = u32 0 ("X-offset IN")
            n62 = call "DMR_GetImageRequestBufferData.vi"("driver handle IN"=w231, "request number IN"=w230) -> ("width OUT"=w220:i32, "height OUT"=w219:i32, "driver handle OUT"=w226:i32, "request number OUT"=w225:i32, "bytes per pixel OUT"=w222:i32)  [unwired: 13 out]
            n63 = call "DMR_GetImageRequestBufferImageData.vi"("driver handle IN"=w226, "request number IN"=w225, "bytes per pixel IN"=w222, "X-offset IN"=w221, "Y-offset IN"=w221, "height IN"=w219, "width IN"=w220) -> ("driver handle OUT"=w224:u32, "request number OUT"=w223:u32, "image OUT"=w216:u32[][])  [unwired: 10 out]
            n64 = call "DMR_ImageRequestUnlock.vi"("request number IN"=w223, "driver handle IN"=w224) -> ("driver handle OUT"=w229:i32)  [unwired: 1 in, 2 out]
            n65 = case shown="False" "Averaging" {
              tunnel: w216 -> [w307 w312]
              tunnel: [w307 w311] -> w212
              tunnel: w215 -> [_ w309]
              frame False {
              }
              frame True {
                (unwired) 1
                w317 = 1
                n66 = feedback #2(w309) -> (w308:u32[][])
                n67 = Add(x=w312, y=w308) -> (x+y=w313:u32[][])
                n68 = Select(t=w309, s="Reset Averaging", f=w313) -> (s? t:f=w315:u32[][])
                n69 = feedback-in #2(w315) -> ()
                n70 = feedback #3(w317) -> (w310:i32)
                n71 = Divide(x=w313, y=w310) -> (x/y=w314:dbl[][])
                n72 = Increment(x=w310) -> (x+1=w318:i32)
                n73 = To Unsigned Long Integer(number=w314) -> (unsigned 32bit integer=w311:u32[][])
                n74 = Select(t=w317, s="Reset Averaging", f=w318) -> (s? t:f=w316:i32)
                n75 = feedback-in #3(w316) -> ()
              }
            }
            n76 = call "DMR_ImageRequestSingle.vi"("request control IN"=0, "driver handle IN"=w229) -> ("driver handle OUT"=w227:i32)  [unwired: 3 out]
            n77 = disable-structure shown="Disabled" {
              disable-tunnel: w212 -> [w284 _]
              disable-tunnel: w211 -> [w283 _]
              frame Disabled {
                n78 = To Double Precision Float(number=w284) -> (double precision float=w282:dbl[][])
                n79 = In Range and Coerce(upper limit="Intensity Upper", x=w282, lower limit="Intensity Lower") -> (coerced(x)=w281:dbl[][])  [unwired: 1 out]
                n80 = Subtract(x="Intensity Upper", y="Intensity Lower") -> (x-y=w278:dbl)
                n81 = Subtract(x=w281, y="Intensity Lower") -> (x-y=w279:dbl[][])
                n82 = Divide(x=w279, y=w278) -> (x/y=w280:dbl[][])
                n83 = Multiply(x=255.0, y=w280) -> (x*y=w276:dbl[][])
                n84 = To Unsigned Byte Integer(number=w276) -> (unsigned 8bit integer=w285:u8[][])
                n85 = call "IMAQ ArrayToImage"("Image Pixels (U8)"=w285, "Image"=w283) -> ("Image Out"=w272:T2)  [unwired: 4 in, 5 out]
                n86 = First Call?() -> (First Call?: T/F=w273:bool)
                n87 = case shown="True" w273 {
                  tunnel: w272 -> [w286 w297]
                  frame False {
                    n88 = flat-sequence {
                      tunnel: w286 -> [w292]
                      frame #0 {
                        w289 = FALSE ("Get/Set Status? (Set)")
                        w288 = 0 ("Window Number (0...15)")
                        n89 = call "IMAQ WindSize"("Get/Set Status? (Set)"=w289, "Window Number"=w288) -> ("Width & Height out"=→"Window Size":cluster{"Width":i32, "Height":i32})  [unwired: 4 in, 2 out]
                        n90 = call "IMAQ WindMove"("Window Number (0...15)"=w288, "Get/Set Status? (Set)"=w289) -> ("Coordinates (screen)"=→"Window Position":cluster{"X Position":i32, "Y Position":i32})  [unwired: 3 in, 1 out]
                        n91 = call "IMAQ WindDraw"("Resize to Image Size? (Y)"=FALSE, "Window Number (0...15)"=w288, "Image"=w292) -> ()  [unwired: 7 in, 2 out]
                      }
                      frame #1 {
                        n92 = call "IMAQ WindZoom 2"("Center Point"="Center Point", "Zoom to Fit? (False)"=FALSE, "Zoom Factor"="Zoom Factor") -> ()  [unwired: 5 in, 4 out]
                      }
                    }
                  }
                  frame True {
                    n93 = flat-sequence {
                      tunnel: w297 -> [w300]
                      tunnel: [w298] -> w296
                      tunnel: w296 -> [w302]
                      frame #0 {
                        w299 = TRUE ("Resize to Image Size? (Y)")
                        w298 = 0 ("Window Number (0...15)")
                        n94 = call "IMAQ WindNonTearing"("Window Number"=w298, "NonTearing? (True)"=w299) -> ()  [unwired: 8 in, 2 out]
                        n95 = call "IMAQ WindDraw"("Resize to Image Size? (Y)"=w299, "Window Number (0...15)"=w298, "Image"=w300) -> ()  [unwired: 7 in, 2 out]
                      }
                      frame #1 {
                        n96 = call "IMAQ WindSize"("Scrollbars? (N)"=FALSE, "Width & Height"="Initial Window Size", "Window Number"=w302) -> ()  [unwired: 3 in, 3 out]
                        n97 = call "IMAQ WindMove"("Window Number (0...15)"=w302, "Coordinates (screen)"="Initial Window Position") -> ()  [unwired: 3 in, 2 out]
                      }
                    }
                  }
                }
              }
              frame Enabled {
              }
            }
            n98 = To Unsigned Byte Integer(number=w212) -> (unsigned 8bit integer=w203:u8[][])
            "image8bitArray" <- w203
            n99 = call "IMAQ ArrayToImage"("Image Pixels (U8)"=w203, "Image"=w210) -> ("Image Out"=w208:T2)  [unwired: 4 in, 5 out]
            n100 = case shown="True" "take fixed bead\n Images" {
              tunnel: w203 -> [_ w251]
              tunnel: w204 -> [_ w250]
              frame False {
              }
              frame True {
                n101 = local write "take fixed bead\n Images"(FALSE ("Save 10 Images")) -> ()
                n102 = while {
                  tunnel: w251 -> [w253]
                  tunnel: w250 -> [w252]
                  i -> [w255]
                  stop <- w254 stop-if-true
                  n103 = flat-sequence {
                    tunnel: w253 -> [w265]
                    tunnel: w252 -> [w264]
                    frame #0 {
                      n104 = local read "Image Index"() -> (w261:dbl)
                      n105 = call "Create new save file.vi"("Insert"="fixed_" ("string"), "Ext"=".bmp" ("string"), "Index In"=w261) -> ("Path Out"=w262:path, "Index Out"=w258:dbl)
                      n106 = call <vilib>:"Flatten Pixmap.vi"("colors"=w264, "8-bit pixmap"=w265) -> ("image data"=w263:T18)  [unwired: 4 in, 5 out]
                      n107 = Increment(x=w258) -> (x+1=w257:dbl)
                      n108 = call <vilib>:"Write BMP File.vi"("image data"=w263, "path to BMP file"=w262) -> ()  [unwired: 1 in, 9 out]
                      n109 = local write "Image Index"(w257) -> ()
                    }
                    frame #1 {
                      n110 = Wait (ms)(milliseconds to wait=u32 50) -> ()  [unwired: 1 out]
                    }
                  }
                  n111 = Equal?(x=w255, y=2) -> (x = y?=w254:bool)
                }
              }
            }
            n112 = case shown="True" "Save Video" {
              tunnel: w213 -> [_ w306]
              tunnel: w208 -> [_ w305]
              frame False {
              }
              frame True {
                n113 = call "IMAQ AVI Write Frame"("Image"=w305, "Avi Refnum"=w306) -> ()  [unwired: 2 in, 8 out]
              }
            }
            n114 = case shown="True" "take background images" {
              tunnel: w204 -> [_ w233]
              tunnel: w203 -> [_ w232]
              frame False {
              }
              frame True {
                n115 = while {
                  tunnel: w233 -> [w235]
                  tunnel: w232 -> [w234]
                  i -> [w238]
                  stop <- w236 stop-if-true
                  n116 = flat-sequence {
                    tunnel: w235 -> [w240]
                    tunnel: w234 -> [w239]
                    frame #0 {
                      n117 = local read "Image Index"() -> (w246:dbl)
                      n118 = call "Create new save file.vi"("Insert"="background_" ("string"), "Ext"=".bmp" ("string"), "Index In"=w246) -> ("Path Out"=w242:path, "Index Out"=w243:dbl)
                      n119 = call <vilib>:"Flatten Pixmap.vi"("colors"=w240, "8-bit pixmap"=w239) -> ("image data"=w241:T18)  [unwired: 4 in, 5 out]
                      n120 = Increment(x=w243) -> (x+1=w247:dbl)
                      n121 = local write "Image Index"(w247) -> ()
                      n122 = call <vilib>:"Write BMP File.vi"("image data"=w241, "path to BMP file"=w242) -> ()  [unwired: 1 in, 9 out]
                    }
                    frame #1 {
                      n123 = Wait (ms)(milliseconds to wait=u32 50) -> ()  [unwired: 1 out]
                    }
                  }
                  n124 = Equal?(x=w238, y=9) -> (x = y?=w236:bool)
                }
              }
            }
            n125 = case shown="False" "Target" {
              tunnel: w208 -> [w267 w271]
              tunnel: [w267 w269] -> w207
              frame False {
              }
              frame True {
                n126 = local read "Target coordinates"() -> (w268:cluster{"X1":dbl, "Y1":dbl, "X2":dbl, "Y2":dbl})
                n127 = call "IMAQ Overlay Oval"("Color"=u32 16711680, "Bounding Rectangle"=w268, "Image"=w271) -> ("Image Out"=w269:T2)  [unwired: 7 in, 1 out]
              }
            }
            "Primary Video Display" <- w207
            n128 = case shown="True" "Save Image" {
              tunnel: w203 -> [_ w321]
              tunnel: w204 -> [_ w320]
              frame False {
              }
              frame True {
                n129 = call <vilib>:"Flatten Pixmap.vi"("colors"=w320, "8-bit pixmap"=w321) -> ("image data"=w327:T18)  [unwired: 4 in, 5 out]
                n130 = call "Create new save file.vi"("Insert"="video_frame_" ("string"), "Ext"=".bmp" ("string"), "Index In"="Image Index") -> ("Path Out"=w323:path, "Index Out"=w328:dbl)
                n131 = Increment(x=w328) -> (x+1=w322:dbl)
                n132 = local write "Image Index"(w322) -> ()
                n133 = call <vilib>:"Write BMP File.vi"("image data"=w327, "path to BMP file"=w323) -> ()  [unwired: 1 in, 9 out]
              }
            }
            "GreyscaleArray" <- w204
          }
        }
        n134 = node-c288(w165) -> ()  [unwired: 1 out]
      }
      n135 = node-c288(w149) -> ()  [unwired: 1 out]
      n136 = call "DMR_CloseDevice2.vi"("driver handle IN"=w154) -> ()  [unwired: 3 in, 2 out]
    }
    frame #4 {
      n137 = call "DMR_Close.vi"() -> ()  [unwired: 1 out]
    }
  }
  n138 = while {
    tunnel: [w412] -> w84
    tunnel: [w583] -> w85
    tunnel: [w410] -> w83
    tunnel: [w691] -> w80
    tunnel: w38 -> [w397]
    tunnel: w37 -> [w687]
    tunnel: w36 -> [w692]
    stop <- w691 stop-if-true
    w448 = "NI_ChannelName" ("name")
    w354 = "NI_ChannelName" ("name")
    w511 = -1
    # "Negate these value to make Force feedback work in X. 6-14-18 A.T."
    # "BX - AX"
    # "BY - AY"
    # "Scan # counter"
    # "DAQ loop iteration\ncounter (for timing)"
    # "Step counter"
    # "Force feedback"
    # "Raster scan"
    # "Rewire everything"
    # "Invert these because changed\nfrom PSD to QPD"
    # "Trap Y"
    # "Trap X"
    # "Convert to\npN"
    # "Convert to\nnm"
    # "Subtract\noffset"
    # "Normalize by\nsum"
    # "B sum"
    # "BX"
    # "BY"
    # "AX"
    # "AY"
    # "A sum"
    # "Close files when done saving"
    n139 = disable-structure shown="Disabled" {
      frame Disabled {
        n140 = property class="DAQmx Read"() -> ("AvailSampPerChan"=→"AvailSampPerChan 2":u32)  [unwired: 2 in, 2 out]
      }
      frame Enabled {
      }
    }
    n141 = local read "Averaging Number"() -> (w420:i32)
    n142 = local read "Averaging Number"() -> (w422:i32)
    "# Samples/channel" <- w422
    n143 = local read "Sampling Rate"() -> (w690:dbl)
    n144 = call-poly <vilib>:"DAQmx Read.vi"("task/channels in"=w397, "number of samples per channel"=w420, "timeout"=10.0) -> ("task out"=w396:refnum<k21>, "data"=w421:dbl[][], "error out"=w512:errorcluster)  [unwired: 10 in]
    n145 = Unbundle By Name(w512) -> ("status"=w631:bool)
    n146 = Divide(x=w690, y="Cal Averaging") -> (x/y=→"Cal Final Sampling Rate":dbl)
    n147 = Divide(x=w690, y=w422) -> (x/y=→"Final Sampling Rate" →"# Samples/channel/s":dbl)
    n148 = Index Array(array=w421, index (row)=4) -> (element=w341:dbl[])  [unwired: 1 in]
    n149 = disable-structure shown="Disabled" {
      frame Disabled {
        n150 = local read "Buffer size\n(Samples/channel)"() -> (w709:u32)
        n151 = property class="DAQmx Read"() -> ("AvailSampPerChan"=w710:u32)  [unwired: 2 in, 2 out]
        "AvailSampPerChan" <- w710
        n152 = Divide(x=w710, y=w709) -> (x/y=→"Buffer status":dbl)
      }
      frame Enabled {
      }
    }
    n153 = Index Array(array=w421, index (row)=5) -> (element=w343:dbl[])  [unwired: 1 in]
    n154 = Index Array(array=w421, index (row)=0) -> (element=w373:dbl[])  [unwired: 1 in]
    n155 = Index Array(array=w421, index (row)=3) -> (element=w372:dbl[])  [unwired: 1 in]
    n156 = Index Array(array=w421, index (row)=1) -> (element=w371:dbl[])  [unwired: 1 in]
    n157 = Index Array(array=w421, index (row)=7) -> (element=w369:dbl[])  [unwired: 1 in]
    n158 = Index Array(array=w421, index (row)=2) -> (element=w374:dbl[])  [unwired: 1 in]
    n159 = Index Array(array=w421, index (row)=6) -> (element=w370:dbl[])  [unwired: 1 in]
    n160 = case shown="True" w631 {
      frame False {
      }
      frame True {
        n161 = call <vilib>:"Beep.vi"() -> ()  [unwired: 12 in]
        "Buffer Overflow" <- TRUE
      }
    }
    n162 = Divide(x=w374, y=w370) -> (x/y=w368:dbl[])
    n163 = Divide(x=w373, y=w370) -> (x/y=w367:dbl[])
    n164 = Divide(x=w372, y=w369) -> (x/y=w366:dbl[])
    n165 = Divide(x=w371, y=w369) -> (x/y=w365:dbl[])
    n166 = local read "Cal values"() -> (w623:T3)
    n167 = call-poly <vilib>:"Mean.vi"("X"=w343) -> ("mean"=w342:dbl)  [unwired: 1 out]
    n168 = Build Array(w368, w367, w366, w365) -> (w364:dbl[][])
    n169 = call-poly <vilib>:"Mean.vi"("X"=w341) -> ("mean"=w340:dbl)  [unwired: 1 out]
    n170 = Bundle("mean"=w342, "mean"=w340) -> (w339:cluster{"mean":dbl, "mean":dbl})  [unwired: 1 in]
    n171 = Unbundle(w623) -> ("AX alpha"=w611:dbl, "BX alpha"=w607:dbl, "AX kappa"=w603:dbl, "BX kappa"=w599:dbl, "AX offset"=w617:dbl, "BX offset"=w615:dbl, "AY alpha"=w614:dbl, "BY alpha"=w609:dbl, "AY kappa"=w605:dbl, "BY kappa"=w601:dbl, "AY offset"=w621:dbl, "BY offset"=w619:dbl)
    n172 = Multiply(x=w371, y=w511) -> (x*y=w509:dbl[])
    n173 = Multiply(x=w373, y=w511) -> (x*y=w510:dbl[])
    n174 = local write "AX alpha"(w611) -> ()
    n175 = local write "BY offset"(w619) -> ()
    n176 = Build Array(w510, w374, w509, w372, w370, w369, w341, w343) -> (w333:dbl[][])
    n177 = local write "BX alpha"(w607) -> ()
    n178 = case shown="True" "Reset data stream" {
      selector: "Reset data stream" -> [_ w858]
      tunnel: w396 -> [w850 w856]
      tunnel: [w850 w854] -> w583
      tunnel: w512 -> [w849 w853]
      tunnel: [w849 w851] -> _
      frame False {
      }
      frame True {
        n179 = Not(x=w858) -> (.not. x?=w857:bool)
        n180 = call <vilib>:"DAQmx Stop Task.vi"("task/channels in"=w856, "error in"=w853) -> ("task out"=w855:refnum<k21>, "error out"=w852:errorcluster)  [unwired: 12 in]
        n181 = local write "Reset data stream"(w857) -> ()
        n182 = local write "Buffer Overflow"(w857) -> ()
        n183 = call <vilib>:"DAQmx Start Task.vi"("task/channels in"=w855, "error in"=w852) -> ("task out"=w854:refnum<k21>, "error out"=w851:errorcluster)  [unwired: 12 in]
      }
    }
    n184 = call-poly <vilib>:"Mean.vi"("X"=w343) -> ("mean"=w637:dbl)  [unwired: 1 out]
    n185 = local write "AY offset"(w621) -> ()
    n186 = call-poly <vilib>:"Mean.vi"("X"=w341) -> ("mean"=w638:dbl)  [unwired: 1 out]
    n187 = call-poly <vilib>:"Mean.vi"("X"=w374) -> ("mean"=w644:dbl)  [unwired: 1 out]
    n188 = call-poly <vilib>:"Mean.vi"("X"=w372) -> ("mean"=w642:dbl)  [unwired: 1 out]
    n189 = call-poly <vilib>:"Mean.vi"("X"=w370) -> ("mean"=w641:dbl)  [unwired: 1 out]
    n190 = call-poly <vilib>:"Mean.vi"("X"=w369) -> ("mean"=w640:dbl)  [unwired: 1 out]
    n191 = local read "Averaging Number"() -> (w419:i32)
    n192 = local write "BY kappa"(w601) -> ()
    n193 = local write "AX kappa"(w603) -> ()
    n194 = call-poly <vilib>:"Mean.vi"("X"=w509) -> ("mean"=w643:dbl)  [unwired: 1 out]
    n195 = local write "AY kappa"(w605) -> ()
    n196 = call-poly <vilib>:"Mean.vi"("X"=w510) -> ("mean"=w645:dbl)  [unwired: 1 out]
    n197 = local read "DAQ rate\n(Samples/s)"() -> (w425:dbl)
    n198 = Build Array(w638, w637) -> (w636:dbl[])
    n199 = local write "BX kappa"(w599) -> ()
    n200 = local write "BY alpha"(w609) -> ()
    n201 = local write "AX offset"(w617) -> ()
    n202 = local write "BX offset"(w615) -> ()
    n203 = local write "AY alpha"(w614) -> ()
    n204 = Build Array(w645, w644, w643, w642, w641, w640) -> (w634:dbl[])
    n205 = local read "Total raster time (s)"() -> (w393:dbl)
    n206 = local read "offset ffb param"() -> (w344:T1)
    n207 = Divide(x=w419, y=w425) -> (x/y=w389:dbl)
    "Data update period (s/set)" <- w389
    n208 = Reciprocal(x=w425) -> (1/x=w426:dbl)
    "Data period (s)" <- w426
    n209 = Divide(x=w393, y=w389) -> (x/y=w392:dbl)
    n210 = Divide(x="Cal time (s)", y=w389) -> (x/y=w388:dbl)
    n211 = Divide(x=w645, y=w641) -> (x/y=w675:dbl)
    n212 = Divide(x=w644, y=w641) -> (x/y=w334:dbl)
    n213 = Round Toward -Infinity(1:w392) -> (0:w391:dbl)
    n214 = Divide(x=w643, y=w640) -> (x/y=w682:dbl)
    n215 = Divide(x=w642, y=w640) -> (x/y=w386:dbl)
    n216 = Round Toward -Infinity(1:w388) -> (0:→"Cal sets to save":dbl)
    n217 = local write "N sets to be saved"(w391) -> ()
    n218 = Build Array("Force Feedback 1", "Force Feedback 2") -> (w350:bool[])
    n219 = Boolean Array To Number(Boolean array=w350) -> (number=w349:u32)
    n220 = Negate(x=w334) -> (-x=w384:dbl)
    n221 = Negate(x=w386) -> (-x=w385:dbl)
    n222 = Subtract(x=w675, y="AY offset") -> (x-y=w657:dbl)
    n223 = Subtract(x=w334, y="AX offset") -> (x-y=w658:dbl)
    n224 = Subtract(x=w682, y="BY offset") -> (x-y=w656:dbl)
    n225 = Subtract(x=w386, y="BX offset") -> (x-y=w659:dbl)
    n226 = Subtract(x=w682, y=w675) -> (x-y=w673:dbl)
    n227 = Subtract(x=w385, y=w384) -> (x-y=w674:dbl)
    n228 = feedback #4(0.0) -> (w582:dbl)
    n229 = Multiply(x="Downsamp\nfact", y=w426) -> (x*y=w362:dbl)
    n230 = Multiply(x=w657, y="AY alpha") -> (x*y=w591:dbl)
    n231 = Multiply(x=w658, y="AX alpha") -> (x*y=w589:dbl)
    n232 = Multiply(x=w659, y="BX alpha") -> (x*y=w590:dbl)
    n233 = Multiply(x=w656, y="BY alpha") -> (x*y=w592:dbl)
    n234 = Add(x=w389, y=w582) -> (x+y=w580:dbl)
    n235 = feedback-in #4(w580) -> ()
    n236 = Square(x=w591) -> (x^2=w667:dbl)
    n237 = Square(x=w589) -> (x^2=w668:dbl)
    n238 = Square(x=w592) -> (x^2=w669:dbl)
    n239 = Square(x=w590) -> (x^2=w670:dbl)
    n240 = Bundle(w673, w674) -> (w381:cluster{dbl, dbl})  [unwired: 1 in]
    n241 = case shown="True" "Set reading to\nsetpoint 1" {
      tunnel: w381 -> [_ w847]
      frame False {
      }
      frame True {
        n242 = property on="Setpoint voltage 1" class="Clust (strict)"("Val(Sgnl)"=w847) -> ()  [unwired: 2 in, 2 out]
        n243 = local read "Trap position (V)"() -> (w846:cluster{"X":dbl, "Y":dbl})
        n244 = local write "Set reading to\nsetpoint 1"(FALSE ("Set reading to\nsetpoint")) -> ()
        n245 = Unbundle(w846) -> ("X"=w845:dbl, "Y"=w844:dbl)
        n246 = Bundle("Y"=w844, "X"=w845) -> (w843:cluster{"Y":dbl, "X":dbl})  [unwired: 1 in]
        n247 = property on="Offset 1" class="Clust (strict)"("Val(Sgnl)"=w843) -> ()  [unwired: 2 in, 2 out]
      }
    }
    n248 = Reciprocal(x=w362) -> (1/x=→"Chart Freq (Hz)":dbl)
    n249 = To Time Stamp(1:w580) -> (0:w361:timestamp)
    n250 = Add(x=w667, y=w668) -> (x+y=w671:dbl)
    n251 = Add(x=w669, y=w670) -> (x+y=w681:dbl)
    n252 = Multiply(x=w589, y="AX kappa") -> (x*y=w585:dbl)
    n253 = Bundle("A y", "A x", "B y", "B x", "A sum", "B sum", "Trap x", "Trap y") -> (w571:T21)  [unwired: 1 in]
    n254 = Multiply(x=w590, y="BX kappa") -> (x*y=w586:dbl)
    n255 = Square Root(x=w671) -> (sqrt(x)=w685:dbl)
    n256 = Square Root(x=w681) -> (sqrt(x)=w684:dbl)
    n257 = Multiply(x=w591, y="AY kappa") -> (x*y=w587:dbl)
    n258 = Multiply(x=w592, y="BY kappa") -> (x*y=w588:dbl)
    n259 = Subtract(x=w637, y="Fixed Y") -> (x-y=w672:dbl)
    n260 = Subtract(x=w638, y="Fixed X") -> (x-y=w676:dbl)
    n261 = Cluster To Array(cluster=w571) -> (array=w570:string[])
    n262 = for {
      tunnel: w333 -> [w836] mode=indexing
      tunnel: w362 -> [w835]
      tunnel: "Downsamp\nfact" -> [w841]
      tunnel: [w839] -> w380 mode=indexing
      tunnel: w361 -> [w842]
      tunnel: w570 -> [w838] mode=indexing
      tunnel: w354 -> [w837]
      n263 = call "Downsample 1D array.vi"("Ave N"=w841, "Arrray In"=w836) -> ("Array Out"=w834:dbl[])  [unwired: 9 in]
      n264 = Bundle By Name("Y"=w834, "dt"=w835, "t0"=w842) -> (w840:waveform(dbl))  [unwired: 1 in]
      n265 = Set Waveform Attribute(5:w838, 6:w837, 7:w840) -> (3:w839:waveform(dbl))  [unwired: 1 in, 2 out]
    }
    "All signals" <- w380
    n266 = Square(x=w587) -> (x^2=w660:dbl)
    n267 = Square(x=w585) -> (x^2=w661:dbl)
    n268 = Square(x=w588) -> (x^2=w662:dbl)
    n269 = Square(x=w586) -> (x^2=w663:dbl)
    n270 = Add(x=w660, y=w661) -> (x+y=w664:dbl)
    n271 = Add(x=w662, y=w663) -> (x+y=w665:dbl)
    n272 = Multiply(x=w672, y="Conv Y (nm/V)") -> (x*y=w594:dbl)
    n273 = Multiply(x=w676, y="Conv X (nm/V)") -> (x*y=w595:dbl)
    n274 = feedback #5() -> (w632:cluster{"B_Y":dbl, "B_X":dbl})  [unwired: 1 in]
    n275 = case shown="1" w349 {
      tunnel: [w1207 w1226 w1239] -> w413
      tunnel: [w1206 w1225 w1240] -> w411
      tunnel: w381 -> [_ w1224 w1242]
      tunnel: [cluster{"B_Y":dbl, "B_X":dbl} {"B_Y"=0.0, "B_X"=0.0} ("Sum error past") w1218 w1237] -> w633
      tunnel: w632 -> [_ w1223 w1238]
      tunnel: w687 -> [w1207 w1221 w1233]
      tunnel: w692 -> [w1206 w1220 w1241]
      tunnel: [0.0 ("B_X") w1213 w1231] -> w347
      tunnel: [cluster{"B_Y":dbl, "B_X":dbl} {"B_Y"=0.0, "B_X"=0.0} ("Sum error past") w1212 w1230] -> w346
      tunnel: "Feedback const" -> [_ w1211 w1232]
      tunnel: w344 -> [_ w1210 w1229]
      tunnel: w339 -> [_ w1209 w1228]
      tunnel: [cluster{dbl, dbl} {0.0, 0.0} ("output cluster") w1208 w1227] -> w338
      frame 0, Default {
        # "Force feedback"
      }
      frame 1 {
        n276 = local write "Force Feedback 2"(FALSE) -> ()
        n277 = call "ForceFeedback4_offsetoutput.vi"("Current Voltage(B-A)"=w1224, "Current Mirror Voltage"=w1209, "offset ffb param"=w1210, "Sum error"=w1223, "task/channels in"=w1221, "error in"=w1220, "Setpoint/Desired Voltage"="Setpoint voltage 1", "Feedback const"=w1211, "offset voltage"="Offset 1") -> ("task out"=w1226:refnum<k21>, "output cluster"=w1208:cluster{dbl, dbl}, "Sum error past"=w1218:cluster{"B_Y":dbl, "B_X":dbl}, "Output Voltage"=w1212:cluster{dbl, dbl}, "error out"=w1225:errorcluster)  [unwired: 4 in, 2 out]
        n278 = local read "Pulling direction"() -> (w1217:bool)
        n279 = Unbundle(w1218) -> ("B_Y"=w1216:dbl, "B_X"=w1215:dbl)
        n280 = Select(t=w1216, s=w1217, f=w1215) -> (s? t:f=w1213:dbl)
      }
      frame 2 {
        n281 = local write "Force Feedback 1"(FALSE) -> ()
        n282 = call "ForceFeedback4_offsetoutput.vi"("Current Voltage(B-A)"=w1242, "Current Mirror Voltage"=w1228, "offset ffb param"=w1229, "Sum error"=w1238, "task/channels in"=w1233, "error in"=w1241, "Setpoint/Desired Voltage"="Setpoint voltage 2", "Feedback const"=w1232, "offset voltage"="Offset 2") -> ("task out"=w1239:refnum<k21>, "output cluster"=w1227:cluster{dbl, dbl}, "Sum error past"=w1237:cluster{"B_Y":dbl, "B_X":dbl}, "Output Voltage"=w1230:cluster{dbl, dbl}, "error out"=w1240:errorcluster)  [unwired: 4 in, 2 out]
        n283 = local read "Pulling direction"() -> (w1234:bool)
        n284 = Unbundle(w1237) -> ("B_Y"=w1236:dbl, "B_X"=w1235:dbl)
        n285 = Select(t=w1236, s=w1234, f=w1235) -> (s? t:f=w1231:dbl)
      }
    }
    "Sum error" <- w347
    "Feedback Output \nVoltage 2" <- w346
    "offset fit ffb output" <- w338
    n286 = feedback-in #5(w633) -> ()
    n287 = Square Root(x=w664) -> (sqrt(x)=w593:dbl)
    n288 = Square Root(x=w665) -> (sqrt(x)=w686:dbl)
    n289 = Add(x=w593, y=w686) -> (x+y=w666:dbl)
    n290 = case shown="True" "Set reading to\nsetpoint 2" {
      tunnel: w381 -> [_ w704]
      frame False {
      }
      frame True {
        n291 = local read "Trap position (V)"() -> (w707:cluster{"X":dbl, "Y":dbl})
        n292 = property on="Setpoint voltage 2" class="Clust (strict)"("Val(Sgnl)"=w704) -> ()  [unwired: 2 in, 2 out]
        n293 = local write "Set reading to\nsetpoint 2"(FALSE) -> ()
        n294 = Unbundle(w707) -> ("X"=w706:dbl, "Y"=w705:dbl)
        n295 = Bundle("Y"=w705, "X"=w706) -> (w703:cluster{"Y":dbl, "X":dbl})  [unwired: 1 in]
        n296 = property on="Offset 2" class="Clust (strict)"("Val(Sgnl)"=w703) -> ()  [unwired: 2 in, 2 out]
      }
    }
    n297 = Build Array(w675, w334, w682, w386, w641, w640, w593, w686, w685, w684, w595, w594) -> ()  [unwired: 1 out]
    n298 = Divide(x=w666, y=2.0) -> (x/y=w630:dbl)
    n299 = Bundle("AX/Asum", "AY/Asum", "BX/Bsum", "BY/Bsum") -> (w356:cluster{string, string, string, string})  [unwired: 1 in]
    n300 = Index Array(array=w380, index=6) -> (element=w450:waveform(dbl))
    n301 = Index Array(array=w380, index=7) -> (element=w452:waveform(dbl))
    n302 = Cluster To Array(cluster=w356) -> (array=w355:string[])
    n303 = for {
      tunnel: w364 -> [w702] mode=indexing
      tunnel: "Downsamp\nfact" -> [w701]
      tunnel: w362 -> [w700]
      tunnel: w361 -> [w698]
      tunnel: w355 -> [w696] mode=indexing
      tunnel: w354 -> [w695]
      tunnel: [w694] -> w353 mode=indexing
      n304 = call "Downsample 1D array.vi"("Ave N"=w701, "Arrray In"=w702) -> ("Array Out"=w699:dbl[])  [unwired: 9 in]
      n305 = Bundle By Name("Y"=w699, "dt"=w700, "t0"=w698) -> (w697:waveform(dbl))  [unwired: 1 in]
      n306 = Set Waveform Attribute(5:w696, 6:w695, 7:w697) -> (3:w694:waveform(dbl))  [unwired: 1 in, 2 out]
    }
    "All signals 2" <- w353
    n307 = local read "Fixed X"() -> (w499:dbl)
    n308 = local read "Fixed Y"() -> (w501:dbl)
    n309 = Unbundle By Name(w450) -> ("Y"=w503:dbl[])
    n310 = Unbundle By Name(w452) -> ("Y"=w502:dbl[])
    n311 = Index Array(array=w380, index=0) -> (element=w457:waveform(dbl))
    n312 = Index Array(array=w380, index=1) -> (element=w567:waveform(dbl))
    n313 = Index Array(array=w380, index=4) -> (element=w561:waveform(dbl))
    n314 = Subtract(x=w503, y=w499) -> (x-y=w500:dbl[])
    n315 = Subtract(x=w502, y=w501) -> (x-y=w497:dbl[])
    n316 = Unbundle By Name(w457) -> ("Y"=w559:dbl[])
    n317 = Unbundle By Name(w567) -> ("Y"=w558:dbl[])
    n318 = Unbundle By Name(w561) -> ("Y"=w557:dbl[])
    n319 = Index Array(array=w380, index=5) -> (element=w560:waveform(dbl))
    n320 = local read "Conv X (nm/V)"() -> (w498:dbl)
    n321 = Unbundle(w338) -> (w337:dbl, w336:dbl)
    n322 = local read "Conv Y (nm/V)"() -> (w496:dbl)
    n323 = Index Array(array=w380, index=2) -> (element=w375:waveform(dbl))
    n324 = Index Array(array=w380, index=3) -> (element=w564:waveform(dbl))
    n325 = Set Waveform Attribute(5:"T2 X", 6:w448, 7:w450) -> (3:w449:waveform(dbl))  [unwired: 1 in, 2 out]
    n326 = Set Waveform Attribute(5:"T2 Y", 6:w448, 7:w452) -> (3:w451:waveform(dbl))  [unwired: 1 in, 2 out]
    n327 = Unbundle By Name(w560) -> ("Y"=w554:dbl[])
    n328 = Unbundle By Name(w375) -> ("Y"=w556:dbl[])
    n329 = Unbundle By Name(w564) -> ("Y"=w555:dbl[])
    n330 = Divide(x=w559, y=w557) -> (x/y=w379:dbl[])
    n331 = Divide(x=w558, y=w557) -> (x/y=w378:dbl[])
    n332 = local read "AY offset"() -> (w545:dbl)
    n333 = Build Array(w337, w336) -> (w335:dbl[])
    n334 = local read "AX offset"() -> (w543:dbl)
    n335 = Multiply(x=w500, y=w498) -> (x*y=w443:dbl[])
    n336 = Multiply(x=w497, y=w496) -> (x*y=w445:dbl[])
    n337 = Divide(x=w555, y=w554) -> (x/y=w376:dbl[])
    n338 = local read "Raster scanning..."() -> (w395:bool)
    n339 = Subtract(x=w378, y=w543) -> (x-y=w546:dbl[])
    n340 = local read "BX offset"() -> (w553:dbl)
    n341 = local read "Saving"() -> (w596:bool)
    n342 = local read "Tether"() -> (w597:bool)
    n343 = Subtract(x=w379, y=w545) -> (x-y=w547:dbl[])
    n344 = Divide(x=w556, y=w554) -> (x/y=w377:dbl[])
    n345 = local read "AY alpha"() -> (w544:dbl)
    n346 = local read "AX alpha"() -> (w542:dbl)
    n347 = call-poly <vilib>:"Mean.vi"("X"=w445) -> ("mean"=w479:dbl)  [unwired: 1 out]
    "Mean Trp Pos Y 2 (nm)" <- w479
    n348 = Subtract(x=w377, y=w379) -> (x-y=w469:dbl[])
    n349 = Subtract(x=w376, y=w378) -> (x-y=w468:dbl[])
    n350 = local read "BY offset"() -> (w550:dbl)
    n351 = Subtract(x=w443, y="Offset X (nm)") -> (x-y=w442:dbl[])
    n352 = Subtract(x=w445, y="Offset Y (nm)") -> (x-y=w444:dbl[])
    n353 = Subtract(x=w377, y=w550) -> (x-y=w552:dbl[])
    n354 = Subtract(x=w376, y=w553) -> (x-y=w551:dbl[])
    n355 = Less?(x=w630, y="Tether break\nforce (pN)") -> (x < y?=w628:bool)
    n356 = Subtract(x=w479, y=w445) -> (x-y=w478:dbl[])
    n357 = call-poly <vilib>:"Mean.vi"("X"=w443) -> ("mean"=w483:dbl)  [unwired: 1 out]
    "Mean Trap Pos X 2 (nm)" <- w483
    n358 = Build Array(w469, w468) -> (w466:dbl[][])
    n359 = Index Array(array=w466, index (row)=0) -> (element=w464:dbl[])  [unwired: 1 in]
    n360 = Index Array(array=w466, index (row)=1) -> (element=w463:dbl[])  [unwired: 1 in]
    n361 = call-poly <vilib>:"Mean.vi"("X"=w464) -> ("mean"=w462:dbl)  [unwired: 1 out]
    n362 = call-poly <vilib>:"Mean.vi"("X"=w463) -> ("mean"=w461:dbl)  [unwired: 1 out]
    n363 = Bundle("mean"=w462, "mean"=w461) -> ()  [unwired: 1 in, 1 out]
    n364 = local read "BX alpha"() -> (w548:dbl)
    n365 = Multiply(x=w547, y=w544) -> (x*y=w535:dbl[])
    n366 = Multiply(x=w546, y=w542) -> (x*y=w534:dbl[])
    n367 = Square(x=w478) -> (x^2=w477:dbl[])
    n368 = Subtract(x=w483, y=w443) -> (x-y=w482:dbl[])
    n369 = Bundle By Name(cluster=w451, "Y"=w444) -> (w494:waveform(dbl))
    n370 = Bundle By Name(cluster=w449, "Y"=w442) -> (w495:waveform(dbl))
    n371 = Compound Arithmetic op=AND(w596, w597, w628) -> (w627:bool)
    n372 = local read "BY alpha"() -> (w549:dbl)
    n373 = Square(x=w482) -> (x^2=w481:dbl[])
    n374 = case shown="True" w627 {
      selector: w627 -> [_ w864]
      tunnel: w395 -> [w859 w861]
      tunnel: [w859 w861] -> w394
      frame False {
      }
      frame True {
        n375 = stacked-sequence {
          frame #0 {
            n376 = property on="Cancel Rep\n Dip" class="Bool (strict)"("Val(Sgnl)"=TRUE) -> ()  [unwired: 2 in, 2 out]
          }
          frame #1 {
            n377 = local write "Cancel Rep\n Dip"(FALSE ("Cancel Rep\n Dip")) -> ()
          }
          frame #2 {
            n378 = property on="Stop saving" class="Bool (strict)"("Val(Sgnl)"="TA Cancel Save?") -> ()  [unwired: 2 in, 2 out]
          }
        }
        n379 = And(x=w861, y="Fish After TA?") -> (x .and. y?=w863:bool)
        n380 = case shown="True" w863 {
          selector: w863 -> [_ w868]
          frame False {
          }
          frame True {
            n381 = property on="Fish" class="Bool (strict)"("Val(Sgnl)"=w868) -> ()  [unwired: 2 in, 2 out]
          }
        }
        n382 = call <vilib>:"Beep.vi"() -> ()  [unwired: 12 in]
        n383 = Not(x=w864) -> (.not. x?=w860:bool)
        n384 = local write "Force Feedback 1"(w860) -> ()
        n385 = local write "Tether"(w860) -> ()
        n386 = local write "Force Feedback 2"(w860) -> ()
      }
    }
    n387 = call-poly <vilib>:"Mean.vi"("X"=w477) -> ("mean"=w476:dbl)  [unwired: 1 out]
    n388 = Square(x=w535) -> (x^2=w541:dbl[])
    n389 = Multiply(x=w552, y=w549) -> (x*y=w533:dbl[])
    n390 = Square(x=w534) -> (x^2=w540:dbl[])
    n391 = Multiply(x=w551, y=w548) -> (x*y=w532:dbl[])
    n392 = call-poly <vilib>:"Mean.vi"("X"=w481) -> ("mean"=w480:dbl)  [unwired: 1 out]
    n393 = Build Array(w495, w494) -> (w414:waveform(dbl)[])
    "Trap sep" <- w414
    n394 = Square Root(x=w476) -> (sqrt(x)=w475:dbl)
    n395 = Square(x=w533) -> (x^2=w539:dbl[])
    n396 = Square(x=w532) -> (x^2=w538:dbl[])
    n397 = Add(x=w541, y=w540) -> (x+y=w537:dbl[])
    n398 = Square Root(x=w480) -> (sqrt(x)=w473:dbl)
    n399 = Multiply(x=w475, y=10) -> (x*y=→"T2 Y RMS (A)":dbl)
    n400 = Square Root(x=w537) -> (sqrt(x)=w438:dbl[])
    n401 = Add(x=w539, y=w538) -> (x+y=w536:dbl[])
    n402 = Set Waveform Attribute(5:"T2", 6:"NI_ChannelName" ("name"), 7:w457) -> (3:w456:waveform(dbl))  [unwired: 1 in, 2 out]
    n403 = Set Waveform Attribute(5:"T1", 6:"NI_ChannelName" ("name"), 7:w375) -> (3:w454:waveform(dbl))  [unwired: 1 in, 2 out]
    n404 = Square Root(x=w536) -> (sqrt(x)=w437:dbl[])
    n405 = Multiply(x=w473, y=10) -> (x*y=→"T2 X RMS (A)":dbl)
    n406 = Bundle By Name(cluster=w456, "Y"=w438) -> (w460:waveform(dbl))
    n407 = Bundle By Name(cluster=w454, "Y"=w437) -> (w514:waveform(dbl))
    n408 = Add(x=w438, y=w437) -> (x+y=w436:dbl[])
    n409 = case shown="True" "Remove offsets" {
      selector: "Remove offsets" -> [_ w832]
      frame False {
      }
      frame True {
        n410 = local read "Mean Trp Pos Y 2 (nm)"() -> (w830:dbl)
        n411 = Not(x=w832) -> (.not. x?=w833:bool)
        n412 = local read "Mean Trap Pos X 2 (nm)"() -> (w831:dbl)
        n413 = local write "Remove offsets"(w833) -> ()
        n414 = local write "Offset Y (nm)"(w830) -> ()
        n415 = local write "Offset X (nm)"(w831) -> ()
      }
    }
    n416 = Build Array(w460, w514) -> (→"Bead sep":waveform(dbl)[])
    n417 = local read "AY kappa"() -> (w531:dbl)
    n418 = local read "AX kappa"() -> (w530:dbl)
    n419 = Divide(x=w436, y=2) -> (x/y=w434:dbl[])
    n420 = local read "BX kappa"() -> (w528:dbl)
    n421 = local read "BY kappa"() -> (w529:dbl)
    n422 = call-poly <vilib>:"Mean.vi"("X"=w434) -> ("mean"=w433:dbl)  [unwired: 1 out]
    "Mean Bead Sep\n(nm)" <- w433
    n423 = local read "Calibrating"() -> (w348:bool)
    n424 = Multiply(x=w535, y=w531) -> (x*y=w524:dbl[])
    n425 = Multiply(x=w534, y=w530) -> (x*y=w525:dbl[])
    n426 = Square(x=w524) -> (x^2=w523:dbl[])
    n427 = Square(x=w525) -> (x^2=w522:dbl[])
    n428 = Subtract(x=w434, y=w433) -> (x-y=w432:dbl[])
    n429 = Multiply(x=w533, y=w529) -> (x*y=w526:dbl[])
    n430 = Multiply(x=w532, y=w528) -> (x*y=w527:dbl[])
    n431 = Or(x=w394, y="Raster scan") -> (x .or. y?=w409:bool)
    n432 = Add(x=w523, y=w522) -> (x+y=w519:dbl[])
    n433 = Square(x=w432) -> (x^2=w431:dbl[])
    n434 = call-poly <vilib>:"Mean.vi"("X"=w431) -> ("mean"=w430:dbl)  [unwired: 1 out]
    n435 = Square Root(x=w519) -> (sqrt(x)=w493:dbl[])
    n436 = Square(x=w526) -> (x^2=w521:dbl[])
    n437 = Square(x=w527) -> (x^2=w520:dbl[])
    n438 = Add(x=w521, y=w520) -> (x+y=w518:dbl[])
    n439 = Bundle By Name(cluster=w456, "Y"=w493) -> (w517:waveform(dbl))
    n440 = Square Root(x=w518) -> (sqrt(x)=w492:dbl[])
    n441 = local read "Saving"() -> (w626:bool)
    n442 = Or(x=w348, y=w626) -> ()  [unwired: 1 out]
    n443 = Square Root(x=w430) -> (sqrt(x)=w429:dbl)
    n444 = Multiply(x=10, y=w429) -> (x*y=→"Bead Sep Noise\n(A)":dbl)
    n445 = Bundle By Name(cluster=w454, "Y"=w492) -> (w516:waveform(dbl))
    n446 = Add(x=w493, y=w492) -> (x+y=w491:dbl[])
    n447 = Build Array(w517, w516) -> (→"Force (pN)":waveform(dbl)[])
    n448 = Divide(x=w491, y=2) -> (x/y=w488:dbl[])
    n449 = call-poly <vilib>:"Mean.vi"("X"=w488) -> ("mean"=w489:dbl)  [unwired: 1 out]
    "Mean force (pN)" <- w489
    n450 = Subtract(x=w489, y=w488) -> (x-y=w487:dbl[])
    n451 = Square(x=w487) -> (x^2=w486:dbl[])
    n452 = call-poly <vilib>:"Mean.vi"("X"=w486) -> ("mean"=w485:dbl)  [unwired: 1 out]
    n453 = flat-sequence {
      tunnel: w348 -> [w911]
      tunnel: w626 -> [_]
      tunnel: w348 -> [_]
      tunnel: w626 -> [_]
      tunnel: w333 -> [w898]
      tunnel: [w898] -> w647
      tunnel: w512 -> [w897]
      tunnel: [w897] -> w646
      tunnel: w634 -> [w896]
      tunnel: [w896] -> w639
      tunnel: w636 -> [w895]
      tunnel: [w895] -> w635
      tunnel: [w892] -> w625
      tunnel: [w889] -> w624
      tunnel: [w886] -> w508
      tunnel: [w885] -> w507
      tunnel: [w882] -> w506
      tunnel: w416 -> [w879]
      tunnel: ["Save Data"] -> w415
      tunnel: [w872] -> w383
      tunnel: w647 -> [w1082]
      tunnel: w646 -> [w1092]
      tunnel: w639 -> [_]
      tunnel: w635 -> [_]
      tunnel: w625 -> [w1091]
      tunnel: w624 -> [w1090]
      tunnel: w508 -> [w1089]
      tunnel: w507 -> [w1088]
      tunnel: w506 -> [w1087]
      tunnel: w415 -> [w1086]
      tunnel: w414 -> [w1085]
      tunnel: w383 -> [w1083]
      tunnel: w335 -> [w1081]
      frame #0 {
        w878 = 0.0
        # "1: old trap\n0: fleezers"
        # "Create files if saving data"
        n454 = local read "Save N sets"() -> (w881:bool)
        n455 = local read "Fixed X"() -> (w877:dbl)
        n456 = local read "Trap position (V)"() -> (w906:cluster{"X":dbl, "Y":dbl})
        n457 = local read "Fixed Y"() -> (w876:dbl)
        n458 = local read "Sampling Rate"() -> (w909:dbl)
        n459 = Or(x=w881, y="Save Data") -> (x .or. y?=w880:bool)
        n460 = Build Array(w880, "Save cal", w879) -> (w900:bool[])
        n461 = Compound Arithmetic op=OR("Save Data", "Save cal", w879) -> (w902:bool)
        n462 = Boolean Array To Number(Boolean array=w900) -> (number=w899:u32)
        n463 = Unbundle(w906) -> ("X"=w875:dbl, "Y"=w874:dbl)
        n464 = Build Array(w875, w874, w877, w876, w878, w878) -> (w905:dbl[])
        n465 = feedback #6(refnum<k0> refnum) -> (w871:refnum<file>)
        n466 = feedback #7(0) -> (w903:i32)
        n467 = feedback #8(refnum<k0> refnum) -> (w893:refnum<file>)
        n468 = feedback #9() -> (w887:dbl)  [unwired: 1 in]
        n469 = feedback #10(FALSE) -> (w883:bool)
        n470 = feedback #11(refnum<k0> refnum) -> (w890:refnum<file>)
        n471 = case shown="True" w902 {
          tunnel: w911 -> [_ _]
          tunnel: 9 -> [_ w957]
          tunnel: w909 -> [_ w956]
          tunnel: 6 -> [_ w955]
          tunnel: 5 -> [_ w954]
          tunnel: w905 -> [_ w953]
          tunnel: [w917 1] -> w886
          tunnel: w903 -> [w918 _]
          tunnel: w899 -> [_ w929]
          tunnel: [w916 w928] -> w892
          tunnel: w893 -> [w916 _]
          tunnel: [w915 w927] -> w889
          tunnel: w890 -> [w915 _]
          tunnel: 1.0 -> [_ w926]
          tunnel: [w914 w925] -> w885
          tunnel: w887 -> [w914 _]
          tunnel: [w913 w924] -> w882
          tunnel: w883 -> [w913 _]
          tunnel: [w912 w919] -> w872
          tunnel: w871 -> [w912 _]
          frame False {
            n472 = Increment(x=w918) -> (x+1=w917:i32)
          }
          frame True {
            w930 = FALSE ("Save Data")
            w935 = FALSE
            w936 = T20."big-endian, network order" ("byte order (0:big-endian, network order)")
            n473 = local write "Save cal"(w930) -> ()
            n474 = local write "Save Data"(w930) -> ()
            n475 = case shown="1, Default" w929 {
              tunnel: w957 -> [w1031 w1049 w1080]
              tunnel: w956 -> [w1012 w1048 w1058]
              tunnel: w955 -> [w1030 w1046 w1076]
              tunnel: w954 -> [w1029 w1045 w1075]
              tunnel: w953 -> [w1028 w1042 w1072]
              tunnel: [w1027 w1041 w1061] -> w950
              tunnel: [w1010 w1032 w1053] -> w924
              tunnel: ["Default data save Avg Num" 200 w1050] -> _
              tunnel: w926 -> [w1017 w1034 w1059]
              tunnel: [w1013 w1033 w1054] -> w925
              tunnel: [w1010 w1032 w1052] -> w921
              frame 1, Default {
                w1010 = TRUE
                w1018 = 0.0
                # "stage x,yz"
                # "Save N number/length of data. e.g. N =200 \nwill give only 200 long data points"
                # "Time trace"
                n476 = Boolean To (0,1)(Boolean=w1010) -> (0, 1=w1022:i16)
                n477 = Increment(x=w1022) -> (x+1=w1021:i16)
                n478 = Divide(x=w1012, y="Default data save Avg Num") -> (x/y=w1026:dbl)
                n479 = To Double Precision Float(number=w1021) -> (double precision float=w1020:dbl)
                n480 = Reciprocal(x=w1026) -> (1/x=w1025:dbl)
                n481 = Reciprocal(x=w1012) -> (1/x=w1011:dbl)
                n482 = Build Array(w1031, w1011, w1025, w1030, w1029, 0 ("f")) -> (w1024:dbl[])
                n483 = Build Array(w1020, w1017, w1018, w1018, w1018) -> (w1023:dbl[])
                n484 = Build Array (concatenate)(w1024, w1028, w1023) -> (w1027:dbl[])
                n485 = Select(t="N sets", s="Save N sets", f=2147483647) -> (s? t:f=w1013:i32)
              }
              frame 2 {
                w1032 = FALSE
                w1037 = 0.0
                # "Calibration file"
                n486 = Reciprocal(x=w1048) -> (1/x=w1047:dbl)
                n487 = Boolean To (0,1)(Boolean=w1032) -> (0, 1=w1040:i16)
                n488 = To Double Precision Float(number=w1040) -> (double precision float=w1039:dbl)
                n489 = Build Array(w1049, w1047, w1047, w1046, w1045, 1) -> (w1043:dbl[])
                n490 = Build Array(w1039, w1034, w1037, w1037, w1037) -> (w1038:dbl[])
                n491 = Build Array (concatenate)(w1043, w1042, w1038) -> (w1041:dbl[])
                n492 = local read "Cal sets to save"() -> (w1033:i32)
                "Calibrating" <- TRUE ("Calibrating")
              }
              frame 4 {
                w1051 = FALSE ("Raster scan")
                w1068 = 0.0
                w1053 = TRUE
                # "Not using ncycles"
                # "FX curve"
                n493 = Not(x=w1053) -> (.not. x?=w1052:bool)
                n494 = local read "Averaging Number"() -> (w1079:i32)
                n495 = Boolean To (0,1)(Boolean=w1053) -> (0, 1=w1071:i16)
                n496 = local write "Saving Move"(w1051) -> ()
                n497 = Divide(x=w1058, y=w1079) -> (x/y=w1078:dbl)
                n498 = Increment(x=w1071) -> (x+1=w1070:i16)
                n499 = local write "Raster scan"(w1051) -> ()
                n500 = To Double Precision Float(number=w1070) -> (double precision float=w1069:dbl)
                n501 = Reciprocal(x=w1078) -> (1/x=w1077:dbl)
                n502 = Reciprocal(x=w1058) -> (1/x=w1057:dbl)
                n503 = Build Array(w1069, w1059, w1068, w1068, w1068) -> (w1067:dbl[])
                n504 = Build Array(w1080, w1057, w1077, w1076, w1075, 2) -> (w1073:dbl[])
                n505 = local read "Scan range (V)"() -> (w1055:dbl)
                n506 = local read "Pulling direction"() -> (w1065:bool)
                n507 = local read "Scan steps (mirror)"() -> (w1056:u64)
                n508 = local read "# scans"() -> (w1063:i32)
                n509 = local read "N sets to be saved"() -> (w1054:dbl)
                n510 = Not(x=w1065) -> (.not. x?=w1064:bool)
                n511 = local read "Averaging Number"() -> (w1050:i32)
                n512 = Boolean To (0,1)(Boolean=w1064) -> (0, 1=w1066:i16)
                n513 = Build Array(w1066, w1055, w1056, 0, w1063) -> (w1062:dbl[])
                n514 = Build Array (concatenate)(w1073, w1072, w1067, w1062) -> (w1061:dbl[])
              }
            }
            n515 = call "CreateSaveFile.vi"("Index In"="Save file index", "Ext"=".dat", "Insert"="", "Directory"="Path") -> ("Index Out"=w923:i32, "Path Out"=w920:path)  [unwired: 6 in]
            "Current file name" <- w920
            n516 = case shown="True" w921 {
              tunnel: w920 -> [_ w969]
              tunnel: [refnum<k0> refnum w966] -> w919
              frame False {
              }
              frame True {
                # "SY 190201 \nAdding functionality to get time points of start and stop moves. \nWehn timetrace save data starts save time point"
                n517 = Path To String(path=w969) -> (string=w973:string)
                n518 = Get Date/Time In Seconds() -> (seconds since 1Jan1904=w983:timestamp)
                n519 = String Length(string=w973) -> (length=w970:i32)
                n520 = Subtract(x=w970, y=4) -> (x-y=w972:i32)
                n521 = Format Date/Time String(time format string (%c)="%H:%M:%S%3u", seconds (now)=w983, UTC format=TRUE) -> (date/time string=w967:string)
                n522 = call <vilib>:"Space Constant.vi"() -> ("String"=w961:string)
                n523 = String Subset(string=w973, length (rest)=w972) -> (substring=w974:string)  [unwired: 1 in]
                n524 = Concatenate Strings(w974, "_stagetime.txt" ("string")) -> (w976:string)
                n525 = String To Path(string=w976) -> (path=w977:path)
                n526 = Open/Create/Replace File(file path (use dialog)=w977, operation (0:open)=T19."create", access (0:read/write)=enum16{"read/write", "read-only", "write-only"}."write-only") -> (refnum out=w981:refnum<file>, error out=w980:errorcluster)  [unwired: 3 in, 1 out]
                n527 = Deny Access(4:w980, 7:w981) -> (3:w982:refnum<file>)  [unwired: 1 in, 1 out]
                n528 = Concatenate Strings(w967, w961, "start", "\r\n") -> (w968:string)
                n529 = Write to Text File(file (use dialog)=w982, text=w968) -> (refnum out=w966:refnum<file>)  [unwired: 2 in, 2 out]
                n530 = local write "Move time"(w967) -> ()
                n531 = local read "Raster scanning..."() -> (w964:bool)
                n532 = local read "Calibrating"() -> (w965:bool)
                n533 = Or(x=w965, y=w964) -> (x .or. y?=w963:bool)
                n534 = Not(x=w963) -> (.not. x?=w962:bool)
                n535 = local write "Saving Move"(w962) -> ()
              }
            }
            n536 = Open/Create/Replace File(file path (use dialog)=w920, operation (0:open)=T19."create", access (0:read/write)=enum16{"read/write", "read-only", "write-only"}."write-only") -> (refnum out=w943:refnum<file>, error out=w944:errorcluster)  [unwired: 3 in, 1 out]
            n537 = local write "Save file index"(w923) -> ()
            n538 = Array Size(array=w950) -> (size(s)=w952:i32)
            n539 = case shown="True" w924 {
              tunnel: w920 -> [_ w1008]
              tunnel: [refnum<k0> refnum w988] -> w927
              frame False {
              }
              frame True {
                w987 = 0.0
                n540 = Path To String(path=w1008) -> (string=w1004:string)
                n541 = Build Array(w987, w987, w987, w987, w987, w987, w987, w987) -> (w992:dbl[])
                n542 = String Length(string=w1004) -> (length=w1007:i32)
                n543 = Array Size(array=w992) -> (size(s)=w994:i32)
                n544 = Subtract(x=w1007, y=4) -> (x-y=w1005:i32)
                n545 = To Double Precision Float(number=w994) -> (double precision float=w993:dbl)
                n546 = String Subset(string=w1004, length (rest)=w1005) -> (substring=w1003:string)  [unwired: 1 in]
                n547 = Build Array (concatenate)(w993, w992) -> (w991:dbl[])
                n548 = Concatenate Strings(w1003, "_pos.dat" ("string")) -> (w1001:string)
                n549 = String To Path(string=w1001) -> (path=w1000:path)
                n550 = Open/Create/Replace File(file path (use dialog)=w1000, operation (0:open)=T19."create", access (0:read/write)=enum16{"read/write", "read-only", "write-only"}."write-only") -> (refnum out=w996:refnum<file>, error out=w997:errorcluster)  [unwired: 3 in, 1 out]
                n551 = Deny Access(4:w997, 7:w996) -> (3:w995:refnum<file>)  [unwired: 1 in, 1 out]
                n552 = Write to Binary File(file (use dialog)=w995, data=w991, 5:FALSE ("prepend array or string size? (T)"), 9:T20."big-endian, network order" ("byte order (0:big-endian, network order)")) -> (refnum out=w988:refnum<file>)  [unwired: 2 in, 2 out]
              }
            }
            n553 = Deny Access(4:w944, 7:w943) -> (0:w934:errorcluster, 3:w942:refnum<file>)  [unwired: 1 in]
            n554 = String Length(string="Comment") -> (length=w949:i32)
            n555 = To Double Precision Float(number=w952) -> (double precision float=w951:dbl)
            n556 = To Double Precision Float(number=w949) -> (double precision float=w948:dbl)
            n557 = Build Array (concatenate)(w951, w950, w948) -> (w939:dbl[])
            n558 = Write to Binary File(file (use dialog)=w942, data=w939, error in=w934, 5:w935, 9:w936) -> (refnum out=w938:refnum<file>, error out=w933:errorcluster)  [unwired: 1 in, 1 out]
            n559 = Write to Binary File(file (use dialog)=w938, data="Comment", error in=w933, 5:w935, 9:w936) -> (refnum out=w928:refnum<file>)  [unwired: 1 in, 2 out]
            "Saving" <- TRUE
          }
        }
        n560 = feedback-in #6(w872) -> ()
        n561 = feedback-in #7(w886) -> ()
        n562 = feedback-in #8(w892) -> ()
        n563 = feedback-in #9(w885) -> ()
        n564 = feedback-in #10(w882) -> ()
        n565 = feedback-in #11(w889) -> ()
      }
      frame #1 {
        n566 = local read "Saving"() -> (w1084:bool)
        n567 = case shown="True" w1084 {
          tunnel: w1082 -> [_ w1113]
          tunnel: w1092 -> [_ w1112]
          tunnel: w1091 -> [_ w1111]
          tunnel: w1090 -> [_ w1110]
          tunnel: w1089 -> [_ w1101]
          tunnel: w1088 -> [_ w1102]
          tunnel: w1087 -> [_ w1105]
          tunnel: w1086 -> [_ w1097]
          tunnel: w1085 -> [_ w1096]
          tunnel: w1083 -> [_ w1094]
          tunnel: w1081 -> [_ w1093]
          frame False {
            (unwired) FALSE ("Calibrating")
          }
          frame True {
            n568 = local read "Stop"() -> (w1108:bool)
            n569 = Less Or Equal?(x=w1101, y=w1102) -> (x <= y?=w1109:bool)
            n570 = Divide(x=w1101, y=w1102) -> (x/y=w1100:dbl)
            n571 = Or(x=w1108, y="Stop saving") -> (x .or. y?=w1095:bool)
            n572 = Multiply(x=100.0, y=w1100) -> (x*y=w1099:dbl)
            n573 = Not(x=w1095) -> (.not. x?=w1107:bool)
            n574 = And(x=w1109, y=w1107) -> (x .and. y?=w1106:bool)
            n575 = case shown="True" w1106 {
              tunnel: w1111 -> [w1118 w1144]
              tunnel: w1112 -> [_ w1143]
              tunnel: w1113 -> [_ w1142]
              tunnel: w1110 -> [w1117 w1141]
              tunnel: w1105 -> [w1114 _]
              tunnel: [0.0 ("Progress") w1140] -> w1104
              tunnel: w1099 -> [_ w1140]
              tunnel: w1097 -> [_ _]
              tunnel: w1096 -> [_ w1139]
              tunnel: w1094 -> [w1115 w1136]
              tunnel: w1093 -> [_ w1135]
              frame False {
                n576 = flat-sequence {
                  tunnel: w1118 -> [w1123]
                  tunnel: w1117 -> [w1122]
                  tunnel: w1115 -> [w1121]
                  tunnel: w1114 -> [w1120]
                  frame #0 {
                    n577 = local read "Saving Move"() -> (w1119:bool)
                    n578 = case shown="True" w1120 {
                      tunnel: w1122 -> [_ w1133]
                      frame False {
                      }
                      frame True {
                        n579 = Close File(refnum=w1133) -> ()  [unwired: 1 in, 2 out]
                      }
                    }
                    n580 = case shown="True" w1119 {
                      tunnel: w1121 -> [_ w1128]
                      frame False {
                      }
                      frame True {
                        n581 = Get Date/Time In Seconds() -> (seconds since 1Jan1904=w1132:timestamp)
                        n582 = call <vilib>:"Space Constant.vi"() -> ("String"=w1127:string)
                        n583 = Format Date/Time String(time format string (%c)="%H:%M:%S%3u", seconds (now)=w1132, UTC format=TRUE) -> (date/time string=w1125:string)
                        n584 = Concatenate Strings(w1125, w1127, "end") -> (w1124:string)
                        n585 = Write to Text File(file (use dialog)=w1128, text=w1124) -> (refnum out=w1129:refnum<file>)  [unwired: 2 in, 2 out]
                        n586 = Close File(refnum=w1129) -> ()  [unwired: 1 in, 2 out]
                        n587 = local write "Move time"(w1125) -> ()
                      }
                    }
                    n588 = Close File(refnum=w1123) -> ()  [unwired: 1 in, 2 out]
                  }
                  frame #1 {
                    w1134 = FALSE
                    n589 = local write "Saving"(w1134) -> ()
                    n590 = local write "Stop saving"(w1134) -> ()
                    n591 = local write "Saving Move"(w1134) -> ()
                    n592 = local write "Calibrating"(w1134) -> ()
                    n593 = call <vilib>:"Beep.vi"() -> ()  [unwired: 12 in]
                  }
                }
              }
              frame True {
                n594 = local read "Calibrating"() -> (w1138:bool)
                n595 = local read "Saving Move"() -> (w1137:bool)
                n596 = case shown="False" w1138 {
                  tunnel: w1144 -> [w1185 w1201]
                  tunnel: w1143 -> [_ w1200]
                  tunnel: w1142 -> [w1172 w1194]
                  tunnel: w1141 -> [w1171 _]
                  tunnel: w1139 -> [w1164 _]
                  tunnel: w1135 -> [w1155 _]
                  frame False {
                    n597 = Array Subset(array=w1172, index (row)=6 ("index"), length (row)=2 ("length")) -> (w1159:dbl[][])  [unwired: 2 in]
                    n598 = Array Subset(array=w1155, index=0, length=1) -> (w1152:dbl[])
                    n599 = Array Subset(array=w1155, index=1, length=1) -> (w1151:dbl[])
                    n600 = local read "Averaging Number"() -> (w1179:i32)
                    n601 = Array Subset(array=w1172, index (row)=0 ("index"), length (row)=6 ("length")) -> (w1168:dbl[][])  [unwired: 2 in]
                    n602 = Build Array (concatenate)(w1159, w1152, w1151) -> (w1158:dbl[][])
                    n603 = Array Size(array=w1168) -> (size(s)=w1175:i32[])
                    n604 = for {
                      tunnel: w1168 -> [w1189] mode=indexing
                      tunnel: w1179 -> [w1191]
                      tunnel: [w1190] -> w1167 mode=indexing
                      n605 = call "Downsample 1D array.vi"("Ave N"=w1191, "Arrray In"=w1189) -> ("Array Out"=w1190:dbl[])  [unwired: 9 in]
                    }
                    n606 = Multiply Array Elements(1:w1175) -> (0:w1174:i32)
                    n607 = for {
                      tunnel: w1158 -> [w1186] mode=indexing
                      tunnel: w1179 -> [w1188]
                      tunnel: [w1187] -> w1170 mode=indexing
                      n608 = call "Downsample 1D array.vi"("Ave N"=w1188, "Arrray In"=w1186) -> ("Array Out"=w1187:dbl[])  [unwired: 9 in]
                    }
                    n609 = Array Size(array=w1158) -> (size(s)=w1178:i32[])
                    n610 = Multiply Array Elements(1:w1178) -> (0:w1177:i32)
                    n611 = Divide(x=w1174, y=w1179) -> (x/y=w1180:dbl)
                    n612 = Divide(x=w1177, y=w1179) -> (x/y=w1176:dbl)
                    n613 = Transpose 2D Array(2D array=w1167) -> (transposed array=w1166:dbl[][])
                    n614 = Transpose 2D Array(2D array=w1170) -> (transposed array=w1165:dbl[][])
                    n615 = Reshape Array(w1166, w1180) -> (w1169:dbl[])
                    n616 = Reshape Array(w1165, w1176) -> (w1173:dbl[])
                    n617 = Index Array(array=w1164, index=0) -> (element=w1161:waveform(dbl))
                    n618 = Index Array(array=w1164, index=1) -> (element=w1160:waveform(dbl))
                    n619 = call <vilib>:"Write File+ [SGL].vi"("1D array"=w1169, "refnum"=w1185) -> ()  [unwired: 7 in, 3 out]
                    n620 = call <vilib>:"Write File+ [SGL].vi"("1D array"=w1173, "refnum"=w1171) -> ()  [unwired: 7 in, 3 out]
                    n621 = Unbundle By Name(w1161) -> ()  [unwired: 1 out]
                    n622 = Unbundle By Name(w1160) -> ()  [unwired: 1 out]
                  }
                  frame True {
                    n623 = Array Subset(array=w1194, index (row)=0 ("index"), length (row)=6 ("length")) -> (w1192:dbl[][])  [unwired: 2 in]
                    n624 = Transpose 2D Array(2D array=w1192) -> (transposed array=w1198:dbl[][])
                    n625 = Array Size(array=w1192) -> (size(s)=w1193:i32[])
                    n626 = Multiply Array Elements(1:w1193) -> (0:w1199:i32)
                    n627 = Reshape Array(w1198, w1199) -> (w1197:dbl[])
                    n628 = call <vilib>:"Write File+ [SGL].vi"("1D array"=w1197, "error in (no error)"=w1200, "refnum"=w1201) -> ()  [unwired: 6 in, 3 out]
                  }
                }
                n629 = case shown="True" w1137 {
                  tunnel: w1136 -> [_ w1145]
                  frame False {
                  }
                  frame True {
                    n630 = event shown="[0] \"Move time\": Value Change" {
                      selector: _ -> [_ _]
                      dyn-events: _ -> [_ _]
                      timeout: 1 -> [_ _]
                      tunnel: w1145 -> [w1150 _]
                      event "Move time": Value Change {
                        n631 = event-data() -> ("NewVal"=w1149:string)  [unwired: 1 in, 5 out]
                        n632 = Concatenate Strings(w1149, "\r\n") -> (w1147:string)
                        n633 = Write to Text File(file (use dialog)=w1150, text=w1147) -> ()  [unwired: 2 in, 3 out]
                      }
                      event Timeout {
                        n634 = event-data() -> ()  [unwired: 1 in, 3 out]
                      }
                    }
                  }
                }
              }
            }
            "Progress" <- w1104
          }
        }
      }
    }
    n635 = Square Root(x=w485) -> (sqrt(x)=→"Force noise (pN)":dbl)
    n636 = local read "Flushing Sample"() -> (w418:bool)
    n637 = case shown="True" w418 {
      frame False {
      }
      frame True {
        n638 = local read "Flush Sample Start Time"() -> (w826:u32)
        n639 = local read "Sample flush time (s)"() -> (w819:dbl)
        n640 = Tick Count (ms)() -> (millisecond timer value=w827:u32)
        n641 = Subtract(x=w827, y=w826) -> (x-y=w817:u32)
        n642 = Multiply(x=u32 1000, y=w819) -> (x*y=w818:dbl)
        n643 = Divide(x=w817, y=w818) -> (x/y=w822:dbl)
        n644 = Greater?(x=w817, y=w818) -> (0:w825:bool)
        n645 = Not(x=w825) -> (.not. x?=w824:bool)
        n646 = Boolean To (0,1)(Boolean=w824) -> (0, 1=w823:i16)
        n647 = Compound Arithmetic op=MULTIPLY(w823, w822, 100.0 ("value")) -> (→"Sample Flush Meter":dbl)
        n648 = case shown="True" w825 {
          frame False {
          }
          frame True {
            w829 = FALSE ("Inject Sample")
            n649 = property on="Clear Volume" class="Bool (strict)"("Val(Sgnl)"=TRUE ("Value (Signaling)")) -> ()  [unwired: 2 in, 2 out]
            n650 = local write "Inject Sample"(w829) -> ()
            n651 = local write "Flushing Sample"(w829) -> ()
          }
        }
      }
    }
    n652 = feedback #12(0) -> (w402:i32)
    n653 = feedback #13(0) -> (w399:i32)
    n654 = feedback #14(0) -> (w404:i32)
    n655 = case shown="True" w409 {
      tunnel: w413 -> [w718 w776]
      tunnel: [w718 w760] -> w412
      tunnel: w411 -> [w717 w775]
      tunnel: [w717 w759] -> w410
      tunnel: "Raster scan" -> [w716 w753]
      tunnel: [w716 w752] -> w407
      tunnel: [0 w751] -> w405
      tunnel: w404 -> [_ w745]
      tunnel: w402 -> [_ w733]
      tunnel: [0 w736] -> w401
      tunnel: w399 -> [_ w742]
      tunnel: [0 w741] -> w398
      frame False {
      }
      frame True {
        # "Reset step counter"
        # "Current position"
        # "Initial values"
        n656 = local read "Conv Y (nm/V)"() -> (w728:dbl)
        n657 = local read "Conv X (nm/V)"() -> (w729:dbl)
        n658 = local read "Trap delta (nm)"() -> (w727:dbl)
        n659 = disable-structure shown="Disabled" {
          frame Disabled {
            n660 = local write "Raster scan"(FALSE ("Raster scan")) -> ()
            n661 = property on="Reset data stream" class="Bool (strict)"("Val(Sgnl)"=TRUE) -> ()  [unwired: 2 in, 2 out]
          }
          frame Enabled {
          }
        }
        n662 = local read "Data update period (s/set)"() -> (w750:dbl)
        n663 = local read "Time per step (ms)"() -> (w747:dbl)
        n664 = Select(t=w728, s="Pulling direction", f=w729) -> (s? t:f=w726:dbl)
        n665 = Divide(x=w727, y=w726) -> (x/y=w725:dbl)
        n666 = local read "Fixed X"() -> (w769:dbl)
        n667 = local read "Fixed Y"() -> (w770:dbl)
        n668 = local read "Fixed X"() -> (w731:dbl)
        n669 = local read "Fixed Y"() -> (w730:dbl)
        n670 = local read "Trap position (V)"() -> (w732:cluster{"X":dbl, "Y":dbl})
        n671 = Select(t=w730, s="Pulling direction", f=w731) -> (s? t:f=w724:dbl)
        n672 = local read "Scan steps (mirror)"() -> (w758:u64)
        n673 = Unbundle(w732) -> ("X"=w722:dbl, "Y"=w723:dbl)
        n674 = Multiply(x=w750, y=1000.0) -> (x*y=w748:dbl)
        n675 = local read "Stop raster"() -> (w765:bool)
        n676 = local read "Stop saving"() -> (w766:bool)
        n677 = Select(t=w769, s="Pulling direction", f=w770) -> (s? t:f=w777:dbl)
        n678 = Add(x=w725, y=w724) -> ()  [unwired: 1 out]
        n679 = local write "Saving Move"(FALSE) -> ()
        n680 = Divide(x=w747, y=w748) -> (x/y=w746:dbl)
        n681 = Quotient & Remainder(x=w745, y=w746) -> (x-y*floor(x/y)=w744:dbl)  [unwired: 1 out]
        n682 = Not(x=w765) -> (.not. x?=w764:bool)
        n683 = Select(t=w723, s="Pulling direction", f=w722) -> (s? t:f=w720:dbl)
        n684 = Not(x=w766) -> (.not. x?=w763:bool)
        n685 = Multiply(x=u64 2, y=w758) -> (x*y=w754:u64)
        n686 = Equal To 0?(x=w744) -> (x = 0?=w743:bool)
        n687 = Less?(x=w733, y=w754) -> (x < y?=w755:bool)
        n688 = Compound Arithmetic op=AND(w755, w764, w763, w743) -> (w756:bool)
        n689 = Not(x=w755) -> (.not. x?=w739:bool)
        n690 = feedback #15() -> (w761:dbl)  [unwired: 1 in]
        n691 = case shown="True" w756 {
          tunnel: w777 -> [_ w812]
          tunnel: w720 -> [_ w794]
          tunnel: w776 -> [w789 w811]
          tunnel: w775 -> [w788 w810]
          tunnel: [w789 w809] -> w760
          tunnel: [w788 w808] -> w759
          tunnel: [w785 w797] -> w762
          tunnel: w733 -> [w786 w792]
          tunnel: w761 -> [w785 w791]
          tunnel: w753 -> [w787 w796]
          tunnel: [w787 w796] -> w752
          tunnel: [w786 w795] -> w737
          frame False {
          }
          frame True {
            # "Go forward or backward?"
            n692 = local read "Scan increment (V)"() -> (w790:dbl)
            n693 = local read "Scan steps (mirror)"() -> (w801:u64)
            n694 = Multiply(x=w790, y=w792) -> (x*y=w793:dbl)
            n695 = Less?(x=w792, y=w801) -> (x < y?=w800:bool)
            n696 = Add(x=w794, y=w793) -> (x+y=w803:dbl)
            n697 = Subtract(x=w791, y=w790) -> (x-y=w802:dbl)
            n698 = Select(t=w803, s=w800, f=w802) -> (s? t:f=w797:dbl)
            n699 = local read "Pulling direction"() -> (w799:bool)
            n700 = Build Array(w797, w812) -> (w806:dbl[])
            n701 = Build Array(w812, w797) -> (w805:dbl[])
            n702 = Select(t=w806, s=w799, f=w805) -> (s? t:f=w804:dbl[])
            n703 = call-poly <vilib>:"DAQmx Write.vi"("task/channels in"=w811, "auto start"=TRUE, "data"=w804, "error in"=w810) -> ("task out"=w809:refnum<k21>, "error out"=w808:errorcluster)  [unwired: 9 in, 1 out]
            n704 = Increment(x=w792) -> (x+1=w795:i32)
            "Raster scanning..." <- TRUE ("Raster scanning...")
          }
        }
        n705 = feedback-in #15(w762) -> ()
        n706 = case shown="True" w739 {
          tunnel: w742 -> [w782 w784]
          tunnel: [w782 w783] -> w741
          frame False {
          }
          frame True {
            n707 = Increment(x=w784) -> (x+1=w783:i32)
          }
        }
        n708 = local read "# scans"() -> (w740:i32)
        n709 = local read "Stop saving"() -> (w768:bool)
        n710 = Greater Or Equal?(x=w741, y=w740) -> (x >= y?=w734:bool)
        n711 = Not(x=w734) -> (.not. x?=w735:bool)
        n712 = And(x=w739, y=w735) -> (x .and. y?=w738:bool)
        n713 = Compound Arithmetic op=OR(w734, "Stop raster", w768) -> (w771:bool)
        n714 = case shown="True" w771 {
          frame False {
          }
          frame True {
            n715 = flat-sequence {
              frame #0 {
                n716 = Wait (ms)(milliseconds to wait=u32 300) -> ()  [unwired: 1 out]
              }
              frame #1 {
                n717 = property on="Trap delta (nm)" class="DigNum (strict)"("Val(Sgnl)"="Trap delta\nafter (nm)") -> ()  [unwired: 2 in, 2 out]
              }
            }
          }
        }
        n718 = And(x="Flow on\nafter raster?", y=w771) -> (x .and. y?=w772:bool)
        n719 = case shown="True" w772 {
          frame False {
          }
          frame True {
            n720 = property on="Inject Sample" class="Bool (strict)"("Val(Sgnl)"=TRUE ("Value (Signaling)")) -> ()  [unwired: 2 in, 2 out]
          }
        }
        n721 = case shown="True" w738 {
          tunnel: w737 -> [w780 _]
          tunnel: [w780 0] -> w736
          frame False {
          }
          frame True {
          }
        }
        n722 = Not(x=w771) -> (.not. x?=w774:bool)
        n723 = local write "Raster scanning..."(w774) -> ()
        n724 = Increment(x=w745) -> (x+1=w751:i32)
      }
    }
    n725 = And(x="Save scans", y=w407) -> (x .and. y?=w416:bool)
    n726 = feedback-in #12(w401) -> ()
    n727 = feedback-in #13(w398) -> ()
    n728 = feedback-in #14(w405) -> ()
    n729 = local read "Stop"() -> (w691:bool)
  }
  n730 = local write "Progress"(u8 0 ("Progress")) -> ()
  n731 = local write "Calibrating"(FALSE ("Calibrating")) -> ()
  n732 = VISA Open(VISA resource name="USB port") -> (VISA resource name=w12:refnum<visa-resource-name>, error out=w11:errorcluster)  [unwired: 1 in, 3 out]
  n733 = VISA Enable Event(8:w11, 10:w10, 11:w12) -> (0:w7:errorcluster, 3:w8:refnum<visa-resource-name>)  [unwired: 1 out]
  n734 = call-poly "VISA Configure Serial Port"("VISA resource name"=refnum<visa-resource-name> "COM5", "baud rate (9600)"=u32 19200) -> ("VISA resource name out"=w2:refnum<visa-resource-name>, "error out"=w28:errorcluster)  [unwired: 12 in]
  n735 = while {
    tunnel: w2 -> [w1292]
    shift-right: [w1288] -> w4
    shift-left: w8 -> [w1291]
    shift-right: [w1289] -> w3
    shift-left: w7 -> [w1290]
    stop <- w1287 stop-if-true
    n736 = global read "FAST_Global_var.vi" "FAST L"() -> (→"FAST Z" →"FAST Z":bool)
    n737 = global read "FAST_Global_var.vi" "FAST R"() -> (→"FAST X-Y" →"FAST X-Y":bool)
    n738 = call "LogitechSubVi.vi"("USB port"=w1291, "VISA resource name in 2 (for the Newport)"=w1292, "error in (no error)"=w1290, "X-Y Wait time"="X-Y Wait time", "Z Wait time"="Z Wait time", "XY Speed Definitions"="XY Speed Definitions", "Z Speed Definitions"="Z Speed Definitions") -> ("Right stick button"=→"Right stick button":bool, "Left stick button"=→"Left stick button":bool, "USB port out"=w1288:refnum<visa-resource-name>, "error out"=w1289:errorcluster, "A B X Y"=w1281:cluster{"A":bool, "B":bool, "X":bool, "Y":bool}, "LB RB"=w1280:T22, "U D L R"=w1286:cluster{"U":bool, "D":bool, "L":bool, "R":bool}, "Sticks"=w1279:T23)  [unwired: 5 in]
    n739 = Unbundle By Name(w1280) -> ("LB"=w1274:bool, "RB"=w1273:bool, "BACK"=w1247:bool, "Logitech"=w1246:bool, "START"=w1248:bool)
    "RB" <- w1273
    "LB" <- w1274
    "BACK" <- w1247
    "START" <- w1248
    "Logitech" <- w1246
    n740 = case shown="True" w1248 {
      selector: w1248 -> [_ w1296]
      frame False {
      }
      frame True {
        n741 = property on="Move to Position 2" class="Bool (strict)"("Val(Sgnl)"=w1296) -> ()  [unwired: 2 in, 2 out]
      }
    }
    n742 = case shown="True" w1246 {
      frame False {
      }
      frame True {
        n743 = local read "Inject Sample"() -> (w1293:bool)
        n744 = Not(x=w1293) -> (.not. x?=w1294:bool)
        n745 = property on="Inject Sample" class="Bool (strict)"("Val(Sgnl)"=w1294) -> ()  [unwired: 2 in, 2 out]
      }
    }
    n746 = case shown="True" w1274 {
      frame False {
      }
      frame True {
        n747 = local read "Shutter 1 (B)"() -> (w1340:bool)
        n748 = Not(x=w1340) -> (.not. x?=w1339:bool)
        n749 = property on="Shutter 1 (B)" class="Bool (strict)"("Val(Sgnl)"=w1339) -> ()  [unwired: 2 in, 2 out]
      }
    }
    n750 = case shown="True" w1247 {
      selector: w1247 -> [_ w1295]
      frame False {
      }
      frame True {
        n751 = property on="Move to Position 1" class="Bool (strict)"("Val(Sgnl)"=w1295) -> ()  [unwired: 2 in, 2 out]
      }
    }
    n752 = Unbundle By Name(w1286) -> ("U"=→"U":bool, "D"=→"D":bool, "L"=→"L":bool, "R"=→"R":bool)
    n753 = Unbundle By Name(w1281) -> ("A"=w1269:bool, "B"=w1267:bool, "X"=w1272:bool, "Y"=w1265:bool)
    "A" <- w1269
    "B" <- w1267
    "X" <- w1272
    "Y" <- w1265
    n754 = case shown="\"Fish\"" "A command" {
      tunnel: w1269 -> [w1319 w1321 w1323 w1326]
      frame "Got ADig", Default {
        n755 = case shown="True" w1319 {
          selector: w1319 -> [_ w1320]
          frame False {
          }
          frame True {
            n756 = property on="Got ADig bead" class="Bool (strict)"("Val(Sgnl)"=w1320) -> ()  [unwired: 2 in, 2 out]
          }
        }
      }
      frame "Dump" {
        n757 = case shown="True" w1321 {
          selector: w1321 -> [_ w1322]
          frame False {
          }
          frame True {
            n758 = property on="Dump beads" class="Bool (strict)"("Val(Sgnl)"=w1322) -> ()  [unwired: 2 in, 2 out]
          }
        }
      }
      frame "Fish" {
        n759 = case shown="True" w1323 {
          frame False {
          }
          frame True {
            n760 = local read "Fish"() -> (w1324:bool)
            n761 = Not(x=w1324) -> (.not. x?=w1325:bool)
            n762 = property on="Fish" class="Bool (strict)"("Val(Sgnl)"=w1325) -> ()  [unwired: 2 in, 2 out]
          }
        }
      }
      frame "Got DNA" {
        n763 = case shown="True" w1326 {
          selector: w1326 -> [_ w1327]
          frame False {
          }
          frame True {
            n764 = property on="Got DNA bead" class="Bool (strict)"("Val(Sgnl)"=w1327) -> ()  [unwired: 2 in, 2 out]
          }
        }
      }
    }
    n765 = case shown="True" w1273 {
      frame False {
      }
      frame True {
        n766 = local read "Shutter 2 (A)"() -> (w1338:bool)
        n767 = Not(x=w1338) -> (.not. x?=w1337:bool)
        n768 = property on="Shutter 2 (A)" class="Bool (strict)"("Val(Sgnl)"=w1337) -> ()  [unwired: 2 in, 2 out]
      }
    }
    n769 = Unbundle By Name(w1279) -> ("Right X"=w1251:i8, "Right Y"=w1253:i8, "Left X"=w1255:i8, "Left Y"=w1260:i8)
    n770 = Not Equal?(x=w1260, y=i8 0) -> (x != y?=w1261:bool)
    n771 = case shown="True" w1261 {
      tunnel: w1260 -> [_ w1300]
      frame False {
      }
      frame True {
        "Left Y" <- w1300
      }
    }
    n772 = case shown="\"Got DNA\", Default" "B command" {
      tunnel: w1267 -> [w1310 w1312 w1314 w1316]
      frame "Got DNA", Default {
        n773 = case shown="True" w1310 {
          selector: w1310 -> [_ w1311]
          frame False {
          }
          frame True {
            n774 = property on="Got DNA bead" class="Bool (strict)"("Val(Sgnl)"=w1311) -> ()  [unwired: 2 in, 2 out]
          }
        }
      }
      frame "Got ADig" {
        n775 = case shown="True" w1312 {
          selector: w1312 -> [_ w1313]
          frame False {
          }
          frame True {
            n776 = property on="Got ADig bead" class="Bool (strict)"("Val(Sgnl)"=w1313) -> ()  [unwired: 2 in, 2 out]
          }
        }
      }
      frame "Dump" {
        n777 = case shown="True" w1314 {
          selector: w1314 -> [_ w1315]
          frame False {
          }
          frame True {
            n778 = property on="Dump beads" class="Bool (strict)"("Val(Sgnl)"=w1315) -> ()  [unwired: 2 in, 2 out]
          }
        }
      }
      frame "Fish" {
        n779 = case shown="True" w1316 {
          frame False {
          }
          frame True {
            n780 = local read "Fish"() -> (w1317:bool)
            n781 = Not(x=w1317) -> (.not. x?=w1318:bool)
            n782 = property on="Fish" class="Bool (strict)"("Val(Sgnl)"=w1318) -> ()  [unwired: 2 in, 2 out]
          }
        }
      }
    }
    n783 = Not Equal?(x=w1251, y=i8 0) -> (x != y?=w1252:bool)
    n784 = Not Equal?(x=w1253, y=i8 0) -> (x != y?=w1254:bool)
    n785 = Not Equal?(x=w1255, y=i8 0) -> (x != y?=w1256:bool)
    n786 = case shown="True" w1256 {
      tunnel: w1255 -> [_ w1299]
      frame False {
      }
      frame True {
        "Left X" <- w1299
      }
    }
    n787 = case shown="False" w1252 {
      tunnel: w1251 -> [_ w1297]
      frame False {
      }
      frame True {
        "Right X" <- w1297
      }
    }
    n788 = case shown="False" w1254 {
      tunnel: w1253 -> [_ w1298]
      frame False {
      }
      frame True {
        "Right Y" <- w1298
      }
    }
    n789 = case shown="\"Dump\", Default" "X command" {
      tunnel: w1272 -> [w1328 w1330 w1333 w1335]
      frame "Dump", Default {
        n790 = case shown="True" w1328 {
          selector: w1328 -> [_ w1329]
          frame False {
          }
          frame True {
            n791 = property on="Dump beads" class="Bool (strict)"("Val(Sgnl)"=w1329) -> ()  [unwired: 2 in, 2 out]
          }
        }
      }
      frame "Fish" {
        n792 = case shown="True" w1330 {
          frame False {
          }
          frame True {
            n793 = local read "Fish"() -> (w1332:bool)
            n794 = Not(x=w1332) -> (.not. x?=w1331:bool)
            n795 = property on="Fish" class="Bool (strict)"("Val(Sgnl)"=w1331) -> ()  [unwired: 2 in, 2 out]
          }
        }
      }
      frame "Got ADig" {
        n796 = case shown="True" w1333 {
          selector: w1333 -> [_ w1334]
          frame False {
          }
          frame True {
            n797 = property on="Got ADig bead" class="Bool (strict)"("Val(Sgnl)"=w1334) -> ()  [unwired: 2 in, 2 out]
          }
        }
      }
      frame "Got DNA" {
        n798 = case shown="True" w1335 {
          selector: w1335 -> [_ w1336]
          frame False {
          }
          frame True {
            n799 = property on="Got DNA bead" class="Bool (strict)"("Val(Sgnl)"=w1336) -> ()  [unwired: 2 in, 2 out]
          }
        }
      }
    }
    n800 = case shown="\"Fish\", Default" "Y command" {
      tunnel: w1265 -> [w1301 w1304 w1306 w1308]
      frame "Fish", Default {
        n801 = case shown="True" w1301 {
          frame False {
          }
          frame True {
            n802 = local read "Fish"() -> (w1302:bool)
            n803 = Not(x=w1302) -> (.not. x?=w1303:bool)
            n804 = property on="Fish" class="Bool (strict)"("Val(Sgnl)"=w1303) -> ()  [unwired: 2 in, 2 out]
          }
        }
      }
      frame "Dump" {
        n805 = case shown="True" w1304 {
          selector: w1304 -> [_ w1305]
          frame False {
          }
          frame True {
            n806 = property on="Dump beads" class="Bool (strict)"("Val(Sgnl)"=w1305) -> ()  [unwired: 2 in, 2 out]
          }
        }
      }
      frame "Got ADig" {
        n807 = case shown="True" w1306 {
          selector: w1306 -> [_ w1307]
          frame False {
          }
          frame True {
            n808 = property on="Got ADig bead" class="Bool (strict)"("Val(Sgnl)"=w1307) -> ()  [unwired: 2 in, 2 out]
          }
        }
      }
      frame "Got DNA" {
        n809 = case shown="True" w1308 {
          selector: w1308 -> [_ w1309]
          frame False {
          }
          frame True {
            n810 = property on="Got DNA bead" class="Bool (strict)"("Val(Sgnl)"=w1309) -> ()  [unwired: 2 in, 2 out]
          }
        }
      }
    }
    n811 = local read "Stop"() -> (w1287:bool)
  }
  n812 = VISA Close(VISA resource name=w4, error in (no error)=w3) -> (error out=w5:errorcluster)
  n813 = call <vilib>:"Simple Error Handler.vi"("error in (no error)"=w5) -> ()  [unwired: 1 in, 8 out]
  n814 = node-c288(i64 100 ("Period"), 2 ("Processor")) -> (w30:T14)  [unwired: 2 in]
  n815 = timed-loop {
    timing: w30 -> [_]
    timing-out: [_] -> w29
    tunnel: w2 -> [w1341]
    tunnel: w28 -> [w1343]
    tunnel: [w1341] -> w27
    stop <- w1342 stop-if-true
    n816 = node-c288() -> ()  [unwired: 1 in, 1 out]
    n817 = event shown="[0] \"Got DNA bead\": Value Change" {
      selector: _ -> [_ _ _ _ _ _ _ _ _ _ _ _ _ _ _ _]
      dyn-events: _ -> [_ _ _ _ _ _ _ _ _ _ _ _ _ _ _ _]
      timeout: _ -> [_ _ _ _ _ _ _ _ _ _ _ _ _ _ _ _]
      tunnel: w1341 -> [w1353 w1417 w1437 w1455 w1473 w1495 w1543 w1558 _ w1715 _ _ _ _ _ _]
      tunnel: w1343 -> [w1352 w1416 w1436 w1454 w1472 w1494 w1542 w1557 _ w1713 _ _ _ _ _ _]
      tunnel: [_ _ _ _ _ _ _ _ _ _ _ _ _ _ _ w1903] -> w1342
      event "Got DNA bead": Value Change {
        n818 = event-data() -> ()  [unwired: 1 in, 5 out]
        n819 = flat-sequence {
          tunnel: w1353 -> [w1358]
          tunnel: "Cal @ Delta (nm)" -> [w1354]
          tunnel: w1352 -> [w1356]
          tunnel: [w1373] -> w1351
          tunnel: "Cal @ Delta (nm)" -> [w1372]
          tunnel: w1351 -> [w1394]
          tunnel: [w1394] -> w1350
          tunnel: w1350 -> [w1400]
          tunnel: [w1400] -> w1348
          tunnel: w1348 -> [w1402]
          tunnel: [w1402] -> w1347
          tunnel: w1347 -> [w1403]
          tunnel: [w1403] -> w1346
          tunnel: w1346 -> [w1411]
          tunnel: [w1411] -> w1345
          tunnel: w1345 -> [w1412]
          frame #0 {
            n820 = disable-structure shown="Disabled" {
              frame Disabled {
                n821 = property on="Inject Pump 2" class="Bool (strict)"("Val(Sgnl)"=FALSE ("Inject Pump 2")) -> ()  [unwired: 2 in, 2 out]
              }
              frame Enabled {
              }
            }
            n822 = local read "Saved stage positions"() -> (w1359:dbl[][])
            n823 = local write "Stage moving"(TRUE ("Stage moving")) -> ()
            n824 = property on="Inject Sample" class="Bool (strict)"("Val(Sgnl)"=TRUE ("Value (Signaling)")) -> ()  [unwired: 2 in, 2 out]
            n825 = property on="Trap delta (nm)" class="DigNum (strict)"("Val(Sgnl)"=w1354) -> ()  [unwired: 2 in, 2 out]
            n826 = call "move to saved stage position.vi"("error in"=w1356, "Stage VISA resource name in"=w1358, "Position"="Cal stage position", "Saved Stage Positions"=w1359) -> ()  [unwired: 2 out]
          }
          frame #1 {
            n827 = local write "Stage moving"(FALSE ("Stage moving")) -> ()
            n828 = call <vilib>:"Beep.vi"() -> ()  [unwired: 12 in]
            n829 = Wait (ms)(milliseconds to wait=u32 2000) -> ()  [unwired: 1 out]
          }
          frame #2 {
            n830 = property on="Inject Sample" class="Bool (strict)"("Val(Sgnl)"=FALSE ("Value (Signaling)")) -> ()  [unwired: 2 in, 2 out]
          }
          frame #3 {
            # "increased from 1000 to 5000 v6.4. \nMar.7,2018."
            n831 = Wait (ms)(milliseconds to wait=u32 2000) -> ()  [unwired: 1 out]
          }
          frame #4 {
            n832 = property on="Save cal" class="Bool (strict)"("Val(Sgnl)"=TRUE ("Value (Signaling)")) -> ()  [unwired: 2 in, 2 out]
          }
          frame #5 {
            n833 = Wait (ms)(milliseconds to wait=u32 2000) -> ()  [unwired: 1 out]
          }
          frame #6 {
            n834 = while {
              stop <- w1369 stop-if-true
              n835 = local read "Saving"() -> (w1370:bool)
              n836 = Not(x=w1370) -> (.not. x?=w1369:bool)
              n837 = Wait (ms)(milliseconds to wait=u32 100) -> ()  [unwired: 1 out]
            }
          }
          frame #7 {
            n838 = Wait (ms)(milliseconds to wait=u32 1000) -> ()  [unwired: 1 out]
          }
          frame #8 {
            n839 = stacked-sequence {
              tunnel: [_ _ _ _ _ _ w1388 _] -> w1373
              tunnel: w1372 -> [_ _ _ _ _ _ _ w1393]
              frame #0 {
                n840 = property on="Trap delta (nm)" class="DigNum (strict)"("Val(Sgnl)"="Offset @ Delta (nm)") -> ()  [unwired: 2 in, 2 out]
                n841 = Replace Array Subset(array=i32[] [0], new element="Offset raster set", index=0) -> (w1377:i32[])
                n842 = property on="Scan Parameters" class="Arr (strict)"("Index Values"=w1377) -> ()  [unwired: 2 in, 2 out]
              }
              frame #1 {
                n843 = Wait (ms)(milliseconds to wait=u32 500) -> ()  [unwired: 1 out]
              }
              frame #2 {
                n844 = property on="Load param" class="Bool (strict)"("Val(Sgnl)"=TRUE ("Load param")) -> ()  [unwired: 2 in, 2 out]
              }
              frame #3 {
                n845 = Wait (ms)(milliseconds to wait=u32 1000) -> ()  [unwired: 1 out]
              }
              frame #4 {
                # "Only continue if there is no buffer\noverflow error"
                n846 = local read "Buffer Overflow"() -> (w1383:bool)
                n847 = Not(x=w1383) -> (.not. x?=w1382:bool)
                n848 = case shown="True" w1382 {
                  frame False {
                  }
                  frame True {
                    n849 = property on="Raster scan" class="Bool (strict)"("Val(Sgnl)"=TRUE ("Value (Signaling)")) -> ()  [unwired: 2 in, 2 out]
                  }
                }
              }
              frame #5 {
                n850 = local read "Buffer Overflow"() -> (w1386:bool)
                n851 = Not(x=w1386) -> (.not. x?=w1385:bool)
                n852 = case shown="True" w1385 {
                  frame False {
                  }
                  frame True {
                    n853 = Wait (ms)(milliseconds to wait=u32 2000) -> ()  [unwired: 1 out]
                  }
                }
              }
              frame #6 {
                n854 = local read "Buffer Overflow"() -> (w1389:bool)
                n855 = Not(x=w1389) -> (.not. x?=w1388:bool)
                n856 = case shown="True" w1388 {
                  frame False {
                  }
                  frame True {
                    n857 = while {
                      stop <- w1391 stop-if-true
                      n858 = local read "Saving"() -> (w1392:bool)
                      n859 = Not(x=w1392) -> (.not. x?=w1391:bool)
                      n860 = Wait (ms)(milliseconds to wait=u32 100) -> ()  [unwired: 1 out]
                    }
                  }
                }
              }
              frame #7 {
                n861 = property on="Trap delta (nm)" class="DigNum (strict)"("Val(Sgnl)"=w1393) -> ()  [unwired: 2 in, 2 out]
              }
            }
          }
          frame #9 {
            n862 = case shown="True" w1394 {
              frame False {
              }
              frame True {
                n863 = case shown="False" "Flow on\nwhile fish?" {
                  frame False {
                    n864 = property on="Inject Sample" class="Bool (strict)"("Val(Sgnl)"=FALSE) -> ()  [unwired: 2 in, 2 out]
                  }
                  frame True {
                    n865 = property on="Inject Sample" class="Bool (strict)"("Val(Sgnl)"=TRUE ("Value (Signaling)")) -> ()  [unwired: 2 in, 2 out]
                  }
                }
                n866 = property on="Read Cal" class="Bool (strict)"("Val(Sgnl)"=TRUE ("Value (Signaling)")) -> ()  [unwired: 2 in, 2 out]
              }
            }
          }
          frame #10 {
            n867 = Wait (ms)(milliseconds to wait=u32 1000) -> ()  [unwired: 1 out]
          }
          frame #11 {
            n868 = property on="Read \nOffset FFB param" class="Bool (strict)"("Val(Sgnl)"=TRUE ("Value (Signaling)")) -> ()  [unwired: 2 in, 2 out]
          }
          frame #12 {
            n869 = stacked-sequence {
              frame #0 {
                n870 = local read "Raster set"() -> (w1405:i32)
                n871 = Replace Array Subset(array=i32[] [0], new element=w1405, index=0) -> (w1404:i32[])
                n872 = property on="Scan Parameters" class="Arr (strict)"("Index Values"=w1404) -> ()  [unwired: 2 in, 2 out]
              }
              frame #1 {
                n873 = Wait (ms)(milliseconds to wait=u32 500) -> ()  [unwired: 1 out]
              }
              frame #2 {
                n874 = property on="Load param" class="Bool (strict)"("Val(Sgnl)"=TRUE ("Load param")) -> ()  [unwired: 2 in, 2 out]
              }
            }
          }
          frame #13 {
            n875 = Wait (ms)(milliseconds to wait=u32 100) -> ()  [unwired: 1 out]
          }
          frame #14 {
            n876 = case shown="True" w1412 {
              frame False {
              }
              frame True {
                n877 = property on="Fish" class="Bool (strict)"("Val(Sgnl)"=TRUE ("Value (Signaling)")) -> ()  [unwired: 2 in, 2 out]
              }
            }
          }
        }
        n878 = local write "Got DNA bead"(FALSE) -> ()
      }
      event "Dump beads": Value Change {
        n879 = event-data() -> ()  [unwired: 1 in, 5 out]
        n880 = flat-sequence {
          tunnel: w1416 -> [w1420]
          tunnel: w1417 -> [w1421]
          tunnel: [w1421] -> w1415
          tunnel: [w1420] -> w1414
          tunnel: w1415 -> [w1424]
          tunnel: w1414 -> [w1423]
          frame #0 {
            w1418 = FALSE ("Fish")
            n881 = local read "Saving"() -> (w1419:bool)
            n882 = local write "Force Feedback 2"(w1418) -> ()
            n883 = local write "Pause dwell"(w1418) -> ()
            n884 = local write "Force Feedback 1"(w1418) -> ()
            n885 = local write "Dump beads"(w1418) -> ()
            n886 = property on="Stop saving" class="Bool (strict)"("Val(Sgnl)"=w1419) -> ()  [unwired: 2 in, 2 out]
            n887 = local write "Fish"(w1418) -> ()
          }
          frame #1 {
            n888 = local read "Saved stage positions"() -> (w1426:dbl[][])
            n889 = case shown="True" "Flow on\ndump?" {
              frame False {
              }
              frame True {
                n890 = property on="Inject Sample" class="Bool (strict)"("Val(Sgnl)"=TRUE ("Value (Signaling)")) -> ()  [unwired: 2 in, 2 out]
              }
            }
            n891 = local write "Stage moving"(TRUE ("Stage moving")) -> ()
            n892 = call "move to saved stage position.vi"("error in"=w1423, "Stage VISA resource name in"=w1424, "Position"=5, "Saved Stage Positions"=w1426) -> ()  [unwired: 2 out]
          }
          frame #2 {
            n893 = local read "Shutter 1 (B)"() -> (w1431:bool)
            n894 = local read "Shutter 2 (A)"() -> (w1430:bool)
            n895 = call <vilib>:"Beep.vi"() -> ()  [unwired: 12 in]
            n896 = case shown="True" w1431 {
              frame False {
              }
              frame True {
                n897 = property on="Shutter 1 (B)" class="Bool (strict)"("Val(Sgnl)"=FALSE ("Value (Signaling)")) -> ()  [unwired: 2 in, 2 out]
              }
            }
            n898 = case shown="True" w1430 {
              frame False {
              }
              frame True {
                n899 = property on="Shutter 2 (A)" class="Bool (strict)"("Val(Sgnl)"=FALSE) -> ()  [unwired: 2 in, 2 out]
              }
            }
            n900 = local write "Stage moving"(FALSE ("Stage moving")) -> ()
            n901 = local write "Tether"(FALSE ("Tether")) -> ()
          }
          frame #3 {
            n902 = property on="Move Cap. 2 (ADig Top)" class="Bool (strict)"("Val(Sgnl)"=TRUE ("Value (Signaling)")) -> ()  [unwired: 2 in, 2 out]
          }
        }
      }
      event "Move Cap. 2 (ADig Top)": Value Change {
        n903 = event-data() -> ()  [unwired: 1 in, 5 out]
        n904 = flat-sequence {
          tunnel: w1437 -> [w1441]
          tunnel: w1436 -> [w1440]
          frame #0 {
            n905 = local read "Saved stage positions"() -> (w1439:dbl[][])
            n906 = case shown="True" "Flow on\ncap 2?" {
              frame False {
              }
              frame True {
                n907 = property on="Inject Sample" class="Bool (strict)"("Val(Sgnl)"=TRUE ("Value (Signaling)")) -> ()  [unwired: 2 in, 2 out]
              }
            }
            n908 = local write "Move Cap. 2 (ADig Top)"(FALSE ("Move Cap. 2 (ADig Top)")) -> ()
            n909 = local write "Stage moving"(TRUE ("Stage moving")) -> ()
            n910 = call "move to saved stage position.vi"("error in"=w1440, "Stage VISA resource name in"=w1441, "Position"=2, "Saved Stage Positions"=w1439) -> ()  [unwired: 2 out]
          }
          frame #1 {
            # "Make sure you don't reverse\nwhich is ON and OFF"
            n911 = local read "Cal @ Delta (nm)"() -> (w1449:dbl)
            n912 = local write "Stage moving"(FALSE ("Stage moving")) -> ()
            n913 = call <vilib>:"Beep.vi"() -> ()  [unwired: 12 in]
            n914 = property on="Trap delta (nm)" class="DigNum (strict)"("Val(Sgnl)"=w1449) -> ()  [unwired: 2 in, 2 out]
            n915 = property class="TabCtl (strict)"("Val(Sgnl)"=T5."Status" ("Value (Signaling)")) -> ()  [unwired: 2 in, 2 out]
            n916 = disable-structure shown="Disabled" {
              frame Disabled {
                n917 = property on="Inject Pump 1" class="Bool (strict)"("Val(Sgnl)"=TRUE ("Inject Pump 2")) -> ()  [unwired: 2 in, 2 out]
              }
              frame Enabled {
              }
            }
            n918 = local read "Shutter 2 (A)"() -> (w1448:bool)
            n919 = case shown="False" w1448 {
              frame False {
                n920 = property on="Shutter 2 (A)" class="Bool (strict)"("Val(Sgnl)"=TRUE ("Value (Signaling)")) -> ()  [unwired: 2 in, 2 out]
              }
              frame True {
              }
            }
            n921 = property on="Inject Sample" class="Bool (strict)"("Val(Sgnl)"=FALSE ("Value (Signaling)")) -> ()  [unwired: 2 in, 2 out]
          }
        }
      }
      event "Got ADig bead": Value Change {
        n922 = event-data() -> ()  [unwired: 1 in, 5 out]
        n923 = flat-sequence {
          tunnel: w1455 -> [w1459]
          tunnel: w1454 -> [w1458]
          frame #0 {
            n924 = local read "Saved stage positions"() -> (w1461:dbl[][])
            n925 = property on="Inject Pump 1" class="Bool (strict)"("Val(Sgnl)"=FALSE ("Inject Pump 2")) -> ()  [unwired: 2 in, 2 out]
            n926 = case shown="True" "Flow on\ncap 1?" {
              frame False {
              }
              frame True {
                n927 = property on="Inject Sample" class="Bool (strict)"("Val(Sgnl)"=TRUE ("Value (Signaling)")) -> ()  [unwired: 2 in, 2 out]
              }
            }
            n928 = local write "Stage moving"(TRUE ("Stage moving")) -> ()
            n929 = call "move to saved stage position.vi"("error in"=w1458, "Stage VISA resource name in"=w1459, "Position"=1, "Saved Stage Positions"=w1461) -> ()  [unwired: 2 out]
          }
          frame #1 {
            n930 = local read "Shutter 1 (B)"() -> (w1465:bool)
            n931 = disable-structure shown="Disabled" {
              frame Disabled {
                n932 = property on="Inject Pump 2" class="Bool (strict)"("Val(Sgnl)"=TRUE ("Inject Pump 2")) -> ()  [unwired: 2 in, 2 out]
              }
              frame Enabled {
              }
            }
            n933 = local write "Stage moving"(FALSE ("Stage moving")) -> ()
            n934 = case shown="False" w1465 {
              frame False {
                n935 = property on="Shutter 1 (B)" class="Bool (strict)"("Val(Sgnl)"=TRUE ("Value (Signaling)")) -> ()  [unwired: 2 in, 2 out]
              }
              frame True {
              }
            }
            n936 = property on="Inject Sample" class="Bool (strict)"("Val(Sgnl)"=FALSE ("Value (Signaling)")) -> ()  [unwired: 2 in, 2 out]
            n937 = call <vilib>:"Beep.vi"() -> ()  [unwired: 12 in]
          }
        }
        n938 = local write "Got ADig bead"(FALSE ("Got ADig bead")) -> ()
      }
      event "Set Position 1", "Set Position 2", "Set Position 3", "Set Position 4", "Set Position 5": Value Change {
        n939 = event-data() -> ()  [unwired: 1 in, 5 out]
        n940 = Build Array("Set Position 1", "Set Position 2", "Set Position 3", "Set Position 4", "Set Position 5", "Set Position 6") -> (w1485:bool[])
        n941 = Boolean Array To Number(Boolean array=w1485) -> (number=w1484:u32)
        n942 = call "Read Stage Position.vi"("error in"=w1472, "VISA resource name in"=w1473) -> ("Current Position"=w1470:cluster{dbl, dbl, dbl}, "error out"=→"Stage error":errorcluster)  [unwired: 1 in, 1 out]
        n943 = Logarithm Base 2(1:w1484) -> (0:w1478:dbl)
        n944 = Cluster To Array(cluster=w1470) -> (array=w1480:dbl[])
        n945 = Increment(x=w1478) -> (x+1=w1481:dbl)
        n946 = Build Array (concatenate)(w1481, w1480) -> (w1479:dbl[])
        n947 = Replace Array Subset(array="Saved stage positions", new element=w1479, index (row)=w1478) -> (w1482:dbl[][])  [unwired: 1 in]
        n948 = local write "Saved stage positions"(w1482) -> ()
      }
      event "Move to Position 6", "Move to Position 4", "Move to Position 3", "Move to Position 5", "Move to Position 1", "Move to Position 2": Value Change {
        w1487 = FALSE
        n949 = event-data() -> ()  [unwired: 1 in, 5 out]
        n950 = Build Array("Move to Position 1", "Move to Position 2", "Move to Position 3", "Move to Position 4", "Move to Position 5", "Move to Position 6") -> (w1498:bool[])
        n951 = Boolean Array To Number(Boolean array=w1498) -> (number=w1497:u32)
        n952 = Logarithm Base 2(1:w1497) -> (0:w1496:dbl)
        n953 = flat-sequence {
          tunnel: w1496 -> [w1507]
          tunnel: w1495 -> [w1506]
          tunnel: w1494 -> [w1505]
          tunnel: [w1500] -> w1489
          tunnel: w1489 -> [w1517]
          frame #0 {
            # "only change move time when \nsaving move in T and calibrating is F"
            n954 = local read "Saved stage positions"() -> (w1508:dbl[][])
            n955 = property on="Saving Move" class="Bool (strict)"() -> ("Value"=w1502:bool)  [unwired: 2 in, 2 out]
            n956 = property on="Calibrating" class="Bool (strict)"() -> ("Value"=w1503:bool)  [unwired: 2 in, 2 out]
            n957 = Not(x=w1503) -> (.not. x?=w1501:bool)
            n958 = Increment(x=w1507) -> (x+1=w1500:dbl)
            n959 = And(x=w1502, y=w1501) -> (x .and. y?=w1504:bool)
            n960 = case shown="True" w1504 {
              frame False {
              }
              frame True {
                n961 = Get Date/Time In Seconds() -> (seconds since 1Jan1904=w1514:timestamp)
                n962 = Format Date/Time String(time format string (%c)="%H:%M:%S%3u", seconds (now)=w1514, UTC format=TRUE) -> (date/time string=w1513:string)
                n963 = call <vilib>:"Space Constant.vi"() -> ("String"=w1512:string)
                n964 = Concatenate Strings(w1513, w1512, "moving") -> (w1510:string)
                n965 = property on="Move time" class="Str"("Val(Sgnl)"=w1510) -> ()  [unwired: 2 in, 2 out]
              }
            }
            n966 = call "move to saved stage position.vi"("error in"=w1505, "Stage VISA resource name in"=w1506, "Position"=w1500, "Saved Stage Positions"=w1508) -> ()  [unwired: 2 out]
            n967 = call <vilib>:"Beep.vi"() -> ()  [unwired: 12 in]
            "Stage moving" <- TRUE ("Stage moving")
          }
          frame #1 {
            n968 = property on="Saving Move" class="Bool (strict)"() -> ("Value"=w1519:bool)  [unwired: 2 in, 2 out]
            n969 = property on="Calibrating" class="Bool (strict)"() -> ("Value"=w1520:bool)  [unwired: 2 in, 2 out]
            n970 = call <vilib>:"Beep.vi"() -> ()  [unwired: 12 in]
            n971 = Not(x=w1520) -> (.not. x?=w1518:bool)
            n972 = local write "Stage moving"(FALSE ("Stage moving")) -> ()
            n973 = And(x=w1519, y=w1518) -> (x .and. y?=w1521:bool)
            n974 = case shown="True" w1521 {
              tunnel: w1517 -> [_ w1525]
              frame False {
              }
              frame True {
                n975 = Get Date/Time In Seconds() -> (seconds since 1Jan1904=w1529:timestamp)
                n976 = Format Date/Time String(time format string (%c)="%H:%M:%S%3u", seconds (now)=w1529, UTC format=TRUE) -> (date/time string=w1528:string)
                n977 = Number To Decimal String(number=w1525, width (-)=i16 1) -> (decimal integer string=w1523:string)
                n978 = call <vilib>:"Space Constant.vi"() -> ("String"=w1526:string)
                n979 = Concatenate Strings(w1528, w1526, w1523) -> (w1527:string)
                n980 = property on="Move time" class="Str"("Val(Sgnl)"=w1527) -> ()  [unwired: 2 in, 2 out]
              }
            }
          }
        }
        n981 = local write "Move to Position 1"(w1487) -> ()
        n982 = local write "Move to Position 2"(w1487) -> ()
        n983 = local write "Move to Position 3"(w1487) -> ()
        n984 = local write "Move to Position 4"(w1487) -> ()
        n985 = local write "Move to Position 5"(w1487) -> ()
        n986 = local write "Move to Position 6"(w1487) -> ()
      }
      event "Set Current\nPos to (0,0,0)": Value Change {
        w1533 = ";" ("string")
        # "DH is \"Define Home\" -KW"
        n987 = event-data() -> ()  [unwired: 1 in, 5 out]
        n988 = local write "Set Current\nPos to (0,0,0)"(FALSE ("Set Current\nPos to (0,0,0)")) -> ()
        n989 = call-poly "VISA Configure Serial Port"("VISA resource name"=w1543, "baud rate (9600)"=u32 19200, "error in (no error)"=w1542) -> ("VISA resource name out"=w1537:refnum<visa-resource-name>, "error out"=w1536:errorcluster)  [unwired: 11 in]
        n990 = Concatenate Strings("1DH" ("string"), w1533, "2DH" ("string"), w1533, "3DH" ("string"), "\r") -> (w1535:string)
        n991 = VISA Write(VISA resource name=w1537, write buffer=w1535, error in (no error)=w1536) -> (error out=w1534:errorcluster)  [unwired: 2 out]
        n992 = local write "Stage error"(w1534) -> ()
      }
      event "Dip": Value Change {
        n993 = event-data() -> ()  [unwired: 1 in, 5 out]
        n994 = property on="Calibrating" class="Bool (strict)"() -> ("Value"=w1550:bool)  [unwired: 2 in, 2 out]
        n995 = Not(x=w1550) -> (.not. x?=w1548:bool)
        n996 = property on="Saving Move" class="Bool (strict)"() -> ("Value"=w1549:bool)  [unwired: 2 in, 2 out]
        n997 = And(x=w1549, y=w1548) -> (x .and. y?=w1547:bool)
        n998 = flat-sequence {
          tunnel: w1558 -> [w1562]
          tunnel: w1557 -> [w1561]
          tunnel: [w1563] -> w1555
          tunnel: [w1562] -> w1553
          tunnel: [w1561] -> w1551
          tunnel: w1547 -> [w1560]
          tunnel: ["Dip position"] -> w1546
          tunnel: [w1579] -> w1556
          tunnel: w1555 -> [w1579]
          tunnel: [w1578] -> w1554
          tunnel: w1553 -> [w1578]
          tunnel: [w1577] -> w1552
          tunnel: w1551 -> [w1577]
          tunnel: w1547 -> [w1573]
          tunnel: w1546 -> [w1572]
          tunnel: w1556 -> [w1610]
          tunnel: w1554 -> [w1609]
          tunnel: w1552 -> [w1608]
          tunnel: w1547 -> [w1606]
          tunnel: ["Start/Return position"] -> w1545
          tunnel: w1547 -> [w1619]
          tunnel: w1545 -> [w1618]
          frame #0 {
            n999 = local read "Saved stage positions"() -> (w1563:dbl[][])
            n1000 = case shown="True" w1560 {
              frame False {
              }
              frame True {
                n1001 = Get Date/Time In Seconds() -> (seconds since 1Jan1904=w1571:timestamp)
                n1002 = call <vilib>:"Space Constant.vi"() -> ("String"=w1567:string)
                n1003 = Format Date/Time String(time format string (%c)="%H:%M:%S%3u", seconds (now)=w1571, UTC format=TRUE) -> (date/time string=w1568:string)
                n1004 = Concatenate Strings(w1568, w1567, "moving") -> (w1566:string)
                n1005 = property on="Move time" class="Str"("Val(Sgnl)"=w1566) -> ()  [unwired: 2 in, 2 out]
              }
            }
            n1006 = local write "Stage moving"(TRUE) -> ()
            n1007 = call "move to saved stage position.vi"("error in"=w1561, "Stage VISA resource name in"=w1562, "Position"="Dip position", "Saved Stage Positions"=w1563) -> ()  [unwired: 2 out]
          }
          frame #1 {
            n1008 = node-c288() -> (w1576:T14)  [unwired: 4 in]
            n1009 = case shown="True" w1573 {
              tunnel: w1572 -> [_ w1583]
              frame False {
              }
              frame True {
                n1010 = Get Date/Time In Seconds() -> (seconds since 1Jan1904=w1588:timestamp)
                n1011 = Number To Decimal String(number=w1583, width (-)=i16 1) -> (decimal integer string=w1582:string)
                n1012 = Format Date/Time String(time format string (%c)="%H:%M:%S%3u", seconds (now)=w1588, UTC format=TRUE) -> (date/time string=w1581:string)
                n1013 = call <vilib>:"Space Constant.vi"() -> ("String"=w1585:string)
                n1014 = Concatenate Strings(w1581, w1585, w1582) -> (w1580:string)
                n1015 = property on="Move time" class="Str"("Val(Sgnl)"=w1580) -> ()  [unwired: 2 in, 2 out]
              }
            }
            n1016 = timed-loop {
              timing: w1576 -> [_]
              timing-out: [_] -> w1575
              i -> [w1599]
              stop <- w1592 stop-if-true
              n1017 = node-c288() -> ()  [unwired: 1 in, 1 out]
              n1018 = local read "Cancel Rep\n Dip"() -> (w1589:bool)
              n1019 = Greater Or Equal?(x=w1599, y="Dip duration") -> (x >= y?=w1595:bool)
              n1020 = local read "Dump beads"() -> (w1590:bool)
              n1021 = Or(x=w1595, y="Cancel dwell") -> (x .or. y?=w1594:bool)
              n1022 = Not(x="Pause dwell") -> (.not. x?=w1596:bool)
              n1023 = node-c288() -> ()  [unwired: 1 in, 1 out]
              n1024 = And(x=w1596, y=w1594) -> (x .and. y?=w1593:bool)
              n1025 = Compound Arithmetic op=OR(w1593, w1590, w1589) -> (w1592:bool)
              "Dip elasped time" <- w1599
            }
            n1026 = local write "Stage moving"(FALSE ("Stage moving")) -> ()
            n1027 = node-c288(w1575) -> ()  [unwired: 1 out]
          }
          frame #2 {
            w1604 = FALSE ("Cancel dwell")
            n1028 = case shown="True" w1606 {
              frame False {
              }
              frame True {
                n1029 = Get Date/Time In Seconds() -> (seconds since 1Jan1904=w1617:timestamp)
                n1030 = Format Date/Time String(time format string (%c)="%H:%M:%S%3u", seconds (now)=w1617, UTC format=TRUE) -> (date/time string=w1614:string)
                n1031 = call <vilib>:"Space Constant.vi"() -> ("String"=w1613:string)
                n1032 = Concatenate Strings(w1614, w1613, "moving") -> (w1611:string)
                n1033 = property on="Move time" class="Str"("Val(Sgnl)"=w1611) -> ()  [unwired: 2 in, 2 out]
              }
            }
            n1034 = local write "Cancel dwell"(w1604) -> ()
            n1035 = local write "Cancel Rep\n Dip"(w1604) -> ()
            n1036 = local write "Stage moving"(TRUE) -> ()
            n1037 = call "move to saved stage position.vi"("error in"=w1608, "Stage VISA resource name in"=w1609, "Position"="Start/Return position", "Saved Stage Positions"=w1610) -> ()  [unwired: 2 out]
          }
          frame #3 {
            n1038 = case shown="True" w1619 {
              tunnel: w1618 -> [_ w1621]
              frame False {
              }
              frame True {
                n1039 = Get Date/Time In Seconds() -> (seconds since 1Jan1904=w1629:timestamp)
                n1040 = Number To Decimal String(number=w1621, width (-)=i16 1) -> (decimal integer string=w1622:string)
                n1041 = call <vilib>:"Space Constant.vi"() -> ("String"=w1626:string)
                n1042 = Format Date/Time String(time format string (%c)="%H:%M:%S%3u", seconds (now)=w1629, UTC format=TRUE) -> (date/time string=w1623:string)
                n1043 = Concatenate Strings(w1623, w1626, w1622) -> (w1624:string)
                n1044 = property on="Move time" class="Str"("Val(Sgnl)"=w1624) -> ()  [unwired: 2 in, 2 out]
              }
            }
            n1045 = local write "Stage moving"(FALSE ("Stage moving")) -> ()
          }
          frame #4 {
            n1046 = local write "Dip"(FALSE ("Dip")) -> ()
          }
        }
      }
      event "Grid Movable Trap": Value Change {
        n1047 = event-data() -> ()  [unwired: 1 in, 6 out]
        n1048 = flat-sequence {
          frame #0 {
            n1049 = local write "Shutter 1 (B)"(FALSE ("Shutter 1 (B)")) -> ()
          }
          frame #1 {
            n1050 = while {
              i -> [w1641]
              stop <- w1633 stop-if-true
              # "y lower limit"
              # "y upper limit"
              n1051 = Multiply(x=0.5, y=w1641) -> (x*y=w1639:dbl)
              n1052 = Add(x=0.0, y=w1639) -> (x+y=w1637:dbl)
              n1053 = while {
                tunnel: w1637 -> [w1647]
                tunnel: 0.2 ("x") -> [w1642]
                i -> [w1651]
                stop <- w1650 stop-if-true
                # "x upper limit"
                n1054 = flat-sequence {
                  tunnel: w1651 -> [w1666]
                  tunnel: [w1656] -> w1648
                  tunnel: w1647 -> [w1658]
                  tunnel: [w1661] -> w1645
                  tunnel: [w1660] -> w1643
                  tunnel: w1642 -> [w1654]
                  tunnel: [w1670] -> w1646
                  tunnel: w1645 -> [w1670]
                  tunnel: [w1669] -> w1644
                  tunnel: w1643 -> [w1669]
                  tunnel: w1646 -> [w1673]
                  tunnel: w1644 -> [w1672]
                  frame #0 {
                    w1652 = i16 2 ("precision (6)")
                    w1653 = i16 5 ("width (-)")
                    w1655 = 100.0 ("y")
                    # "x lower limit"
                    n1055 = Multiply(x=w1654, y=w1666) -> (x*y=w1667:dbl)
                    n1056 = Add(x=0.0, y=w1667) -> (x+y=w1656:dbl)
                    n1057 = Multiply(x=w1658, y=w1655) -> (x*y=w1659:dbl)
                    n1058 = Multiply(x=w1656, y=w1655) -> (x*y=w1657:dbl)
                    n1059 = Build Array(w1656, w1658) -> (w1665:dbl[])
                    n1060 = Number To Fractional String(number=w1658, width (-)=w1653, precision (6)=w1652) -> (F-format string=→"moveY":string)  [unwired: 1 in]
                    n1061 = Number To Decimal String(number=w1659) -> (decimal integer string=w1660:string)  [unwired: 1 in]
                    n1062 = Number To Decimal String(number=w1657) -> (decimal integer string=w1661:string)  [unwired: 1 in]
                    n1063 = Number To Fractional String(number=w1656, width (-)=w1653, precision (6)=w1652) -> (F-format string=→"moveX":string)  [unwired: 1 in]
                    n1064 = Array To Cluster(array=w1665) -> (cluster=w1664:cluster{"[0]":dbl, "[1]":dbl})
                    n1065 = property on="Trap position (V)" class="Clust (strict)"("Val(Sgnl)"=w1664) -> ()  [unwired: 2 in, 2 out]
                  }
                  frame #1 {
                    n1066 = Wait (ms)(milliseconds to wait=u32 500) -> ()  [unwired: 1 out]
                  }
                  frame #2 {
                    n1067 = while {
                      tunnel: w1673 -> [w1675]
                      tunnel: w1672 -> [w1674]
                      i -> [w1678]
                      stop <- w1676 stop-if-true
                      n1068 = flat-sequence {
                        tunnel: w1675 -> [w1682]
                        tunnel: w1674 -> [w1681]
                        frame #0 {
                          w1679 = "_" ("string")
                          n1069 = local read "Image Index"() -> (w1691:dbl)
                          n1070 = Concatenate Strings("GridMove_" ("string"), w1682, w1679, w1681, w1679) -> (w1680:string)
                          n1071 = call "Create new save file.vi"("Insert"=w1680, "Ext"=".bmp" ("string"), "Index In"=w1691) -> ("Path Out"=w1687:path, "Index Out"=w1689:dbl)
                          n1072 = local read "GreyscaleArray"() -> (w1685:u32[])
                          n1073 = local read "image8bitArray"() -> (w1686:u8[][])
                          n1074 = Increment(x=w1689) -> (x+1=w1688:dbl)
                          n1075 = local write "Image Index"(w1688) -> ()
                          n1076 = call <vilib>:"Flatten Pixmap.vi"("colors"=w1685, "8-bit pixmap"=w1686) -> ("image data"=w1684:T18)  [unwired: 4 in, 5 out]
                          n1077 = call <vilib>:"Write BMP File.vi"("image data"=w1684, "path to BMP file"=w1687) -> ()  [unwired: 1 in, 9 out]
                        }
                        frame #1 {
                          n1078 = Wait (ms)(milliseconds to wait=u32 50) -> ()  [unwired: 1 out]
                        }
                      }
                      n1079 = Equal?(x=w1678, y=2) -> (x = y?=w1676:bool)
                    }
                  }
                  frame #3 {
                    n1080 = Wait (ms)(milliseconds to wait=u32 50) -> ()  [unwired: 1 out]
                  }
                }
                n1081 = Equal?(x=w1648, y=3.0) -> (x = y?=w1650:bool)
              }
              n1082 = local read "Stop"() -> (w1635:bool)
              n1083 = Equal?(x=w1637, y=2.0) -> (x = y?=w1634:bool)
              n1084 = Or(x=w1635, y=w1634) -> (x .or. y?=w1633:bool)
            }
          }
          frame #2 {
            n1085 = property on="Shutter 2 (A)" class="Bool (strict)"("Val(Sgnl)"=FALSE ("Shutter 2 (A)")) -> ()  [unwired: 2 in, 2 out]
            n1086 = property on="Inject Sample" class="Bool (strict)"("Val(Sgnl)"=TRUE ("Inject Sample")) -> ()  [unwired: 2 in, 2 out]
          }
          frame #3 {
            n1087 = Wait (ms)(milliseconds to wait=u32 10000) -> ()  [unwired: 1 out]
          }
          frame #4 {
            n1088 = property on="Inject Sample" class="Bool (strict)"("Val(Sgnl)"=FALSE ("Inject Sample")) -> ()  [unwired: 2 in, 2 out]
          }
          frame #5 {
            n1089 = while {
              i -> [w1700]
              stop <- w1698 stop-if-true
              n1090 = flat-sequence {
                frame #0 {
                  n1091 = local read "image8bitArray"() -> (w1709:u8[][])
                  n1092 = local read "GreyscaleArray"() -> (w1708:u32[])
                  n1093 = local read "Image Index"() -> (w1707:dbl)
                  n1094 = call "Create new save file.vi"("Insert"="background_" ("string"), "Ext"=".bmp" ("string"), "Index In"=w1707) -> ("Path Out"=w1702:path, "Index Out"=w1704:dbl)
                  n1095 = call <vilib>:"Flatten Pixmap.vi"("colors"=w1708, "8-bit pixmap"=w1709) -> ("image data"=w1701:T18)  [unwired: 4 in, 5 out]
                  n1096 = Increment(x=w1704) -> (x+1=w1703:dbl)
                  n1097 = call <vilib>:"Write BMP File.vi"("image data"=w1701, "path to BMP file"=w1702) -> ()  [unwired: 1 in, 9 out]
                  n1098 = local write "Image Index"(w1703) -> ()
                }
                frame #1 {
                  n1099 = Wait (ms)(milliseconds to wait=u32 500) -> ()  [unwired: 1 out]
                }
              }
              n1100 = Equal?(x=w1700, y=9) -> (x = y?=w1698:bool)
            }
          }
          frame #6 {
            n1101 = local write "Grid Movable Trap"(FALSE ("Grid Movable Trap")) -> ()
            n1102 = property on="Inject Sample" class="Bool (strict)"("Val(Sgnl)"=TRUE ("Value (Signaling)")) -> ()  [unwired: 2 in, 2 out]
          }
        }
      }
      event "Repeat Dip": Value Change {
        n1103 = event-data() -> ()  [unwired: 1 in, 6 out]
        n1104 = local read "Saved stage positions"() -> (w1716:dbl[][])
        n1105 = local read "Calibrating"() -> (w1719:bool)
        n1106 = local read "Saving Move"() -> (w1718:bool)
        n1107 = Not(x=w1719) -> (.not. x?=w1717:bool)
        n1108 = And(x=w1718, y=w1717) -> (x .and. y?=w1714:bool)
        n1109 = flat-sequence {
          tunnel: w1716 -> [w1723]
          tunnel: w1715 -> [w1722]
          tunnel: w1714 -> [w1721]
          tunnel: w1713 -> [w1720]
          frame #0 {
            n1110 = while {
              tunnel: w1723 -> [w1743]
              tunnel: w1722 -> [w1740]
              tunnel: w1721 -> [w1737]
              tunnel: w1721 -> [w1736]
              tunnel: w1720 -> [w1735]
              tunnel: w1720 -> [w1734]
              i -> [w1744]
              stop <- w1725 stop-if-true
              n1111 = flat-sequence {
                tunnel: w1743 -> [w1749]
                tunnel: [w1749] -> w1741
                tunnel: w1740 -> [w1748]
                tunnel: [w1748] -> w1738
                tunnel: w1737 -> [w1747]
                tunnel: w1735 -> [w1746]
                tunnel: [w1745] -> w1730
                tunnel: [w1762] -> w1742
                tunnel: w1741 -> [w1762]
                tunnel: [w1761] -> w1739
                tunnel: w1738 -> [w1761]
                tunnel: w1736 -> [w1760]
                tunnel: w1730 -> [w1759]
                tunnel: w1724 -> [w1758]
                tunnel: w1742 -> [w1796]
                tunnel: w1739 -> [w1795]
                tunnel: w1736 -> [w1794]
                tunnel: w1734 -> [w1793]
                tunnel: [w1792] -> w1729
                tunnel: w1736 -> [w1807]
                tunnel: w1729 -> [w1806]
                tunnel: w1724 -> [w1805]
                frame #0 {
                  n1112 = case shown="True" w1747 {
                    frame False {
                    }
                    frame True {
                      n1113 = Get Date/Time In Seconds() -> (seconds since 1Jan1904=w1757:timestamp)
                      n1114 = call <vilib>:"Space Constant.vi"() -> ("String"=w1753:string)
                      n1115 = Format Date/Time String(time format string (%c)="%H:%M:%S%3u", seconds (now)=w1757, UTC format=TRUE) -> (date/time string=w1754:string)
                      n1116 = Concatenate Strings(w1754, w1753, "moving") -> (w1751:string)
                      n1117 = property on="Move time" class="Str"("Val(Sgnl)"=w1751) -> ()  [unwired: 2 in, 2 out]
                    }
                  }
                  n1118 = local read "Dip position"() -> (w1745:dbl)
                  n1119 = local write "Stage moving"(TRUE) -> ()
                  n1120 = call "move to saved stage position.vi"("error in"=w1746, "Stage VISA resource name in"=w1748, "Position"=w1745, "Saved Stage Positions"=w1749) -> ()  [unwired: 2 out]
                }
                frame #1 {
                  # "IN DIPPING POSITION"
                  n1121 = node-c288() -> (w1765:T14)  [unwired: 4 in]
                  n1122 = case shown="True" w1760 {
                    tunnel: w1759 -> [_ w1770]
                    frame False {
                    }
                    frame True {
                      n1123 = Get Date/Time In Seconds() -> (seconds since 1Jan1904=w1774:timestamp)
                      n1124 = Format Date/Time String(time format string (%c)="%H:%M:%S%3u", seconds (now)=w1774, UTC format=TRUE) -> (date/time string=w1769:string)
                      n1125 = Number To Decimal String(number=w1770, width (-)=i16 1) -> (decimal integer string=w1767:string)
                      n1126 = call <vilib>:"Space Constant.vi"() -> ("String"=w1768:string)
                      n1127 = Concatenate Strings(w1769, w1768, w1767) -> (w1766:string)
                      n1128 = property on="Move time" class="Str"("Val(Sgnl)"=w1766) -> ()  [unwired: 2 in, 2 out]
                    }
                  }
                  n1129 = timed-loop {
                    timing: w1765 -> [_]
                    timing-out: [_] -> w1764
                    tunnel: w1758 -> [w1775]
                    i -> [w1785]
                    stop <- w1777 stop-if-true
                    n1130 = node-c288() -> ()  [unwired: 1 in, 1 out]
                    n1131 = local read "Cancel dwell"() -> (w1783:bool)
                    n1132 = local read "Dip duration"() -> (w1784:dbl)
                    n1133 = local write "Dip elasped time"(w1785) -> ()
                    n1134 = local read "Dump beads"() -> (w1778:bool)
                    n1135 = To Double Precision Float(number=w1785) -> (double precision float=w1786:dbl)
                    n1136 = local read "Pause dwell"() -> (w1787:bool)
                    n1137 = Greater Or Equal?(x=w1786, y=w1784) -> (x >= y?=w1782:bool)
                    n1138 = Or(x=w1782, y=w1783) -> (x .or. y?=w1781:bool)
                    n1139 = Not(x=w1787) -> (.not. x?=w1780:bool)
                    n1140 = local read "Cancel Rep\n Dip"() -> (w1776:bool)
                    n1141 = And(x=w1780, y=w1781) -> (x .and. y?=w1779:bool)
                    n1142 = node-c288() -> ()  [unwired: 1 in, 1 out]
                    n1143 = Compound Arithmetic op=OR(w1776, w1779, w1778, w1775) -> (w1777:bool)
                  }
                  n1144 = local write "Stage moving"(FALSE) -> ()
                  n1145 = node-c288(w1764) -> ()  [unwired: 1 out]
                }
                frame #2 {
                  n1146 = case shown="True" w1794 {
                    frame False {
                    }
                    frame True {
                      n1147 = Get Date/Time In Seconds() -> (seconds since 1Jan1904=w1804:timestamp)
                      n1148 = call <vilib>:"Space Constant.vi"() -> ("String"=w1800:string)
                      n1149 = Format Date/Time String(time format string (%c)="%H:%M:%S%3u", seconds (now)=w1804, UTC format=TRUE) -> (date/time string=w1801:string)
                      n1150 = Concatenate Strings(w1801, w1800, "moving") -> (w1798:string)
                      n1151 = property on="Move time" class="Str"("Val(Sgnl)"=w1798) -> ()  [unwired: 2 in, 2 out]
                    }
                  }
                  n1152 = local read "Start/Return position"() -> (w1792:dbl)
                  n1153 = local write "Stage moving"(TRUE) -> ()
                  n1154 = call "move to saved stage position.vi"("error in"=w1793, "Stage VISA resource name in"=w1795, "Position"=w1792, "Saved Stage Positions"=w1796) -> ()  [unwired: 2 out]
                }
                frame #3 {
                  # "IN RETURN POSITION"
                  n1155 = node-c288() -> (w1810:T14)  [unwired: 4 in]
                  n1156 = timed-loop {
                    timing: w1810 -> [_]
                    timing-out: [_] -> w1809
                    tunnel: w1805 -> [w1820]
                    i -> [w1831]
                    stop <- w1822 stop-if-true
                    n1157 = node-c288() -> ()  [unwired: 1 in, 1 out]
                    n1158 = local read "Return duration"() -> (w1829:dbl)
                    n1159 = local read "Dump beads"() -> (w1823:bool)
                    n1160 = local read "Cancel dwell"() -> (w1827:bool)
                    n1161 = local write "Return elasped time"(w1831) -> ()
                    n1162 = To Double Precision Float(number=w1831) -> (double precision float=w1832:dbl)
                    n1163 = local read "Pause dwell"() -> (w1830:bool)
                    n1164 = Greater Or Equal?(x=w1832, y=w1829) -> (x >= y?=w1828:bool)
                    n1165 = Or(x=w1828, y=w1827) -> (x .or. y?=w1826:bool)
                    n1166 = local read "Cancel Rep\n Dip"() -> (w1821:bool)
                    n1167 = Not(x=w1830) -> (.not. x?=w1825:bool)
                    n1168 = node-c288() -> ()  [unwired: 1 in, 1 out]
                    n1169 = And(x=w1825, y=w1826) -> (x .and. y?=w1824:bool)
                    n1170 = Compound Arithmetic op=OR(w1821, w1824, w1823, w1820) -> (w1822:bool)
                  }
                  n1171 = case shown="True" w1807 {
                    tunnel: w1806 -> [_ w1815]
                    frame False {
                    }
                    frame True {
                      n1172 = Get Date/Time In Seconds() -> (seconds since 1Jan1904=w1819:timestamp)
                      n1173 = Format Date/Time String(time format string (%c)="%H:%M:%S%3u", seconds (now)=w1819, UTC format=TRUE) -> (date/time string=w1812:string)
                      n1174 = Number To Decimal String(number=w1815, width (-)=i16 1) -> (decimal integer string=w1814:string)
                      n1175 = call <vilib>:"Space Constant.vi"() -> ("String"=w1813:string)
                      n1176 = Concatenate Strings(w1812, w1813, w1814) -> (w1811:string)
                      n1177 = property on="Move time" class="Str"("Val(Sgnl)"=w1811) -> ()  [unwired: 2 in, 2 out]
                    }
                  }
                  n1178 = local write "Stage moving"(FALSE) -> ()
                  n1179 = node-c288(w1809) -> ()  [unwired: 1 out]
                }
              }
              n1180 = local read "Tether"() -> (w1726:bool)
              n1181 = Not(x=w1726) -> (.not. x?=w1724:bool)
              n1182 = Increment(x=w1744) -> (x+1=w1732:i32)
              "Dip #" <- w1732
              n1183 = property on="Cancel Rep\n Dip" class="Bool (strict)"() -> ("Value"=w1728:bool)  [unwired: 2 in, 2 out]
              n1184 = To Double Precision Float(number=w1732) -> (double precision float=w1731:dbl)
              n1185 = Greater Or Equal?(x=w1731, y="Dip attempts") -> (x >= y?=w1727:bool)
              n1186 = Compound Arithmetic op=OR(w1728, w1727, w1724) -> (w1725:bool)
            }
          }
          frame #1 {
            w1837 = FALSE
            n1187 = local write "Cancel Rep\n Dip"(w1837) -> ()
            n1188 = call <vilib>:"Beep.vi"() -> ()  [unwired: 12 in]
            n1189 = local write "Repeat Dip"(w1837) -> ()
          }
        }
      }
      event "Force FB script": Value Change {
        n1190 = event-data() -> ()  [unwired: 1 in, 5 out]
        n1191 = flat-sequence {
          frame #0 {
            n1192 = disable-structure shown="Disabled" {
              frame Disabled {
                n1193 = local read "# Samples/channel"() -> (w1840:i32)
                n1194 = local write "# Samples/channel (in)"(w1840) -> ()
              }
              frame Enabled {
              }
            }
            n1195 = local write "Force FB script"(FALSE ("Force FB script")) -> ()
            n1196 = property on="Trap delta (nm)" class="DigNum (strict)"("Val(Sgnl)"="Start trap delta (nm)") -> ()  [unwired: 2 in, 2 out]
          }
          frame #1 {
            n1197 = Wait (ms)(milliseconds to wait=u32 500) -> ()  [unwired: 1 out]
          }
          frame #2 {
            n1198 = property on="Set reading to\nsetpoint 1" class="Bool (strict)"("Val(Sgnl)"=TRUE ("Value (Signaling)")) -> ()  [unwired: 2 in, 2 out]
          }
          frame #3 {
            n1199 = Wait (ms)(milliseconds to wait=u32 300) -> ()  [unwired: 1 out]
          }
          frame #4 {
            n1200 = local write "Force Feedback 1"(TRUE ("Force Feedback")) -> ()
            n1201 = property on="Tabs" class="TabCtl (strict)"("Val(Sgnl)"=T24."Force Feedback" ("Value (Signaling)")) -> ()  [unwired: 2 in, 2 out]
          }
          frame #5 {
            n1202 = property on="Save Data" class="Bool (strict)"("Val(Sgnl)"=TRUE ("Value (Signaling)")) -> ()  [unwired: 2 in, 2 out]
          }
          frame #6 {
            n1203 = Multiply(x="Wait before dip (s)", y=1000) -> (x*y=w1847:dbl)
            n1204 = Wait (ms)(milliseconds to wait=w1847) -> ()  [unwired: 1 out]
          }
          frame #7 {
            n1205 = case shown="True" "Start dipping after?" {
              selector: "Start dipping after?" -> [_ w1852]
              frame False {
              }
              frame True {
                n1206 = property on="Dip" class="Bool (strict)"("Val(Sgnl)"=w1852) -> ()  [unwired: 2 in, 2 out]
              }
            }
            n1207 = property on="Remove offsets" class="Bool (strict)"("Val(Sgnl)"=TRUE ("Value (Signaling)")) -> ()  [unwired: 2 in, 2 out]
          }
        }
      }
      event "Move 0": Value Change {
        n1208 = event-data() -> ()  [unwired: 1 in, 5 out]
        n1209 = local write "Move 0"(FALSE) -> ()
        n1210 = call "HalfWavePlate.vi"("Degrees"="\"Degrees\" 0", "Motor"=0) -> ()  [unwired: 1 in]
      }
      event "Move 1": Value Change {
        n1211 = event-data() -> ()  [unwired: 1 in, 5 out]
        n1212 = local write "Move 1"(FALSE) -> ()
        n1213 = call "HalfWavePlate.vi"("Degrees"="\"Degrees\" 1", "Motor"=1) -> ()  [unwired: 1 in]
      }
      event "Save user params": Value Change {
        n1214 = event-data() -> ()  [unwired: 1 in, 6 out]
        n1215 = local write "Save user params"(FALSE) -> ()
        n1216 = call "save control values.vi"("User"="User") -> ()  [unwired: 8 in, 1 out]
      }
      event "Load user params": Value Change {
        # "Exceptions. Don't load these parameters."
        n1217 = event-data() -> ()  [unwired: 1 in, 6 out]
        n1218 = local write "Load user params"(FALSE) -> ()
        n1219 = flat-sequence {
          tunnel: [w1885] -> w1876
          tunnel: [w1884] -> w1874
          tunnel: [w1883] -> w1872
          tunnel: [w1882] -> w1870
          tunnel: [w1881] -> w1868
          tunnel: [w1880] -> w1866
          tunnel: [w1879] -> w1864
          tunnel: [w1878] -> w1861
          tunnel: [w1893] -> w1877
          tunnel: w1876 -> [w1893]
          tunnel: [w1892] -> w1875
          tunnel: w1874 -> [w1892]
          tunnel: [w1891] -> w1873
          tunnel: w1872 -> [w1891]
          tunnel: [w1890] -> w1871
          tunnel: w1870 -> [w1890]
          tunnel: [w1889] -> w1869
          tunnel: w1868 -> [w1889]
          tunnel: [w1888] -> w1867
          tunnel: w1866 -> [w1888]
          tunnel: [w1887] -> w1865
          tunnel: w1864 -> [w1887]
          tunnel: [w1886] -> w1862
          tunnel: w1861 -> [w1886]
          tunnel: w1877 -> [w1902]
          tunnel: w1875 -> [w1901]
          tunnel: w1873 -> [w1900]
          tunnel: w1871 -> [w1899]
          tunnel: w1869 -> [w1898]
          tunnel: w1867 -> [w1897]
          tunnel: w1865 -> [w1896]
          tunnel: w1862 -> [w1895]
          frame #0 {
            n1220 = local read "Force Feedback 2"() -> (w1878:bool)
            n1221 = local read "Force Feedback 1"() -> (w1879:bool)
            n1222 = local read "Shutter 1 (B)"() -> (w1885:bool)
            n1223 = local read "Shutter 2 (A)"() -> (w1884:bool)
            n1224 = local read "Inject Sample"() -> (w1882:bool)
            n1225 = local read "Trap delta (nm)"() -> (w1881:dbl)
            n1226 = local read "Save file index"() -> (w1880:i32)
            n1227 = local read "Fish"() -> (w1883:bool)
          }
          frame #1 {
            n1228 = local read "User"() -> (w1894:string)
            n1229 = call "retrieve control values.vi"("User"=w1894) -> ()  [unwired: 10 in, 1 out]
          }
          frame #2 {
            n1230 = local write "Force Feedback 1"(w1896) -> ()
            n1231 = local write "Force Feedback 2"(w1895) -> ()
            n1232 = local write "Trap delta (nm)"(w1898) -> ()
            n1233 = local write "Save file index"(w1897) -> ()
            n1234 = local write "Inject Sample"(w1899) -> ()
            n1235 = local write "Shutter 2 (A)"(w1901) -> ()
            n1236 = local write "Shutter 1 (B)"(w1902) -> ()
            n1237 = local write "Fish"(w1900) -> ()
          }
        }
      }
      event "Stop": Value Change {
        n1238 = event-data() -> ()  [unwired: 1 in, 5 out]
        n1239 = local read "Stop"() -> (w1903:bool)
      }
    }
    n1240 = node-c288() -> ()  [unwired: 1 in, 1 out]
  }
  n1241 = call-poly <vilib>:"DAQmx Create Virtual Channel.vi"("lines"=w98) -> ("task out"=w97:refnum<k21>)  [unwired: 13 in, 1 out]
  n1242 = call-poly <vilib>:"DAQmx Create Virtual Channel.vi"("lines"=w101) -> ("task out"=w100:refnum<k21>)  [unwired: 13 in, 1 out]
  n1243 = node-c288(2 ("Processor")) -> (w82:T14)  [unwired: 3 in]
  n1244 = timed-loop {
    timing: w82 -> [_]
    timing-out: [_] -> w81
    stop <- w1906 stop-if-true
    n1245 = node-c288() -> ()  [unwired: 1 in, 1 out]
    n1246 = case shown="\"Control\"" "Tab Control" {
      frame "Control" {
        n1247 = case shown="True" "Start" {
          frame False {
          }
          frame True {
            w1919 = T25 3 items=["no dialog", "OK message", "continue or stop message", "OK message + warnings", "continue/stop + warnings"] ("type of dialog (OK msg:1)")
            n1248 = call "InitializeAcquireFF.vi"("DAQ Rate"="DAQ Rate", "Averaging Number"="Averaging Number", "Sampling Rate"="Sampling Rate") -> ("error out"=w1913:errorcluster, "task out"=w1912:refnum<k21>, "Final Sampling Rate"=→"Final Sampling Rate":dbl)  [unwired: 4 in, 2 out]
            n1249 = while {
              tunnel: [w1931] -> w1918
              tunnel: [w1930] -> w1911
              tunnel: "Averaging Number" -> [w1929]
              tunnel: w1913 -> [w1928]
              tunnel: w1912 -> [w1926]
              stop <- w1927 continue-if-true
              n1250 = call "Acquire2_QPD.vi"("task/channels in"=w1926, "Save Data?"=FALSE ("Take Data?"), "Averaging Number"=w1929, "error in"=w1928) -> ("PSD 1"=→"PSD 1":cluster{dbl[], dbl[]}, "PSD 1 Sum"=→"PSD 1 Sum":dbl, "PSD 2"=→"PSD 2":cluster{dbl[], dbl[]}, "PSD 2 Sum"=→"PSD 2 Sum":dbl, "task out"=w1931:refnum<k21>, "error out"=w1930:errorcluster)  [unwired: 14 in, 4 out]
              n1251 = local read "Start"() -> (w1927:bool)
            }
            n1252 = call <vilib>:"DAQmx Clear Task.vi"("task in"=w1918, "error in"=w1911) -> ("error out"=w1920:errorcluster)  [unwired: 13 in]
            n1253 = call <vilib>:"Simple Error Handler.vi"("type of dialog (OK msg:1)"=w1919, "error in (no error)"=w1920) -> ()  [unwired: 3 in, 5 out]
          }
        }
      }
      frame "Current Saved Data" {
      }
      frame "Data Acquisition" {
      }
      frame "Raw QPD Data" {
      }
    }
    n1254 = local read "Stop"() -> (w1906:bool)
    n1255 = node-c288() -> ()  [unwired: 1 in, 1 out]
  }
  n1256 = node-c288(2 ("Processor")) -> (w34:T14)  [unwired: 3 in]
  n1257 = timed-loop {
    timing: w34 -> [_]
    timing-out: [_] -> w33
    stop <- w1932 stop-if-true
    n1258 = node-c288() -> ()  [unwired: 1 in, 1 out]
    n1259 = event shown="[0] \"Pause Mouse/Mirror Connection\": Value Change" {
      selector: _ -> [_ _]
      dyn-events: _ -> [_ _]
      timeout: _ -> [_ _]
      tunnel: [w2025 _] -> w1933
      tunnel: [_ w2026] -> w1932
      event "Pause Mouse/Mirror Connection": Value Change {
        n1260 = event-data() -> ("NewVal"=w2025:bool)  [unwired: 1 in]
      }
      event "Stop": Value Change {
        n1261 = event-data() -> ("NewVal"=w2026:bool)  [unwired: 1 in]
      }
    }
    n1262 = case shown="True" w1933 {
      frame False {
      }
      frame True {
        n1263 = call "InitializeMouseControl.vi"() -> ("error out 2"=w1942:errorcluster, "task out"=w1943:refnum<k21>, "error out"=w1945:errorcluster, "device ID"=w1944:refnum<k1>)  [unwired: 8 in]
        n1264 = while {
          tunnel: w1945 -> [w1957]
          tunnel: w1944 -> [w1956]
          tunnel: w1943 -> [w1955]
          tunnel: w1942 -> [w1954]
          tunnel: [w1953] -> w1940
          tunnel: [w1952] -> w1939
          tunnel: [w1951] -> w1936
          tunnel: [w1950] -> w1937
          stop <- w1949 stop-if-true
          n1265 = case shown="True" "Use Mouse to Move Trap?" {
            tunnel: w1956 -> [w1964 w1987]
            tunnel: w1957 -> [w1963 w1986]
            tunnel: w1955 -> [w1962 w1985]
            tunnel: w1954 -> [w1961 w1984]
            tunnel: [w1964 w1983] -> w1951
            tunnel: [w1963 w1982] -> w1950
            tunnel: [w1962 w1981] -> w1953
            tunnel: [w1961 w1980] -> w1952
            frame False {
              (unwired) FALSE ("button 1")
            }
            frame True {
              w1975 = 0.0 ("y")
              w1977 = 10
              n1266 = local read "Deflection"() -> (w1988:T6)
              n1267 = call-poly <vilib>:"Acquire Input Data.vi"("device ID"=w1987, "error in (no error)"=w1986) -> ("device ID"=w1983:refnum<k1>, "button info"=w2001:T26, "error out"=w1982:errorcluster)  [unwired: 14 in, 1 out]
              n1268 = Unbundle By Name(w1988) -> ("Horizontal"=w1990:i32, "Vertical"=w1989:i32)
              n1269 = local read "Saved voltage"() -> (w1966:cluster{dbl, dbl})
              n1270 = Divide(x=w1990, y=30) -> (x/y=w1993:dbl)
              n1271 = Divide(x=w1989, y=-20) -> (x/y=w1994:dbl)
              n1272 = Unbundle By Name(w2001) -> ("button 1"=w1979:bool, "button 2"=w1995:bool)
              n1273 = Bundle(w1993, w1994) -> (w1971:cluster{dbl, dbl})  [unwired: 1 in]
              n1274 = local write "Reference Voltage"(w1971) -> ()
              n1275 = Add(x=w1971, y=w1966) -> (x+y=w1999:cluster{dbl, dbl})
              n1276 = case shown="True" w1979 {
                frame False {
                  n1277 = stacked-sequence {
                    frame #0 {
                      n1278 = local write "CoordinatesMousePressed"(T6 {"Horizontal"=0, "Vertical"=0} ("Coords when pressed")) -> ()
                      n1279 = local write "Deflection"(T6 {"Horizontal"=0, "Vertical"=0} ("deflaction")) -> ()
                    }
                  }
                }
                frame True {
                  n1280 = local read "CoordinatesMousePressed"() -> (w2024:T6)
                  n1281 = local read "Real Coordinates"() -> (w2023:cluster{"Horizontal":i32, "Vertical":i32})
                  n1282 = Subtract(x=w2023, y=w2024) -> (x-y=w2022:T6)
                  n1283 = local write "Deflection"(w2022) -> ()
                }
              }
              n1284 = Unbundle(w1999) -> (w1976:dbl, w1967:dbl)
              n1285 = case shown="True" w1995 {
                frame False {
                }
                frame True {
                  n1286 = local read "Reference Voltage"() -> (w2005:cluster{dbl, dbl})
                  n1287 = local read "Saved voltage"() -> (w2003:cluster{dbl, dbl})
                  n1288 = Add(x=w2005, y=w2003) -> (x+y=→"Saved voltage":cluster{dbl, dbl})
                  n1289 = local read "Real Coordinates"() -> (w2004:cluster{"Horizontal":i32, "Vertical":i32})
                  n1290 = local write "CoordinatesMousePressed"(w2004) -> ()
                }
              }
              n1291 = Less?(x=w1976, y=w1977) -> (x < y?=w1974:bool)
              n1292 = Greater?(x=w1976, y=w1975) -> (0:w1973:bool)
              n1293 = Greater?(x=w1967, y=w1975) -> (0:w1969:bool)
              n1294 = Less?(x=w1967, y=w1977) -> (x < y?=w1970:bool)
              n1295 = And(x=w1969, y=w1970) -> (x .and. y?=w1968:bool)
              n1296 = And(x=w1974, y=w1973) -> (x .and. y?=w1972:bool)
              n1297 = case shown="False" w1968 {
                tunnel: [w2015 w2019] -> w1978
                tunnel: w1967 -> [w2013 w2019]
                frame False {
                  n1298 = Greater?(x=w2013, y=10.0) -> (0:w2016:bool)
                  n1299 = case shown="True" w2016 {
                    tunnel: [0.0 10.0] -> w2015
                    frame False {
                    }
                    frame True {
                    }
                  }
                }
                frame True {
                }
              }
              n1300 = case shown="False" w1972 {
                tunnel: w1976 -> [w2007 w2012]
                tunnel: [w2008 w2012] -> w2000
                frame False {
                  n1301 = Greater?(x=w2007, y=10.0) -> (0:w2009:bool)
                  n1302 = case shown="True" w2009 {
                    tunnel: [0.0 10.0] -> w2008
                    frame False {
                    }
                    frame True {
                    }
                  }
                }
                frame True {
                }
              }
              n1303 = Bundle(w2000, w1978) -> (w1965:cluster{dbl, dbl})  [unwired: 1 in]
              n1304 = Cluster To Array(cluster=w1965) -> (array=w1996:dbl[])
              n1305 = call-poly <vilib>:"DAQmx Write.vi"("task/channels in"=w1985, "data"=w1996, "error in"=w1984) -> ("task out"=w1998:refnum<k21>, "error out"=w1997:errorcluster)  [unwired: 10 in, 1 out]
              n1306 = call <vilib>:"DAQmx Is Task Done.vi"("task/channels in"=w1998, "error in"=w1997) -> ("task out"=w1981:refnum<k21>, "error out"=w1980:errorcluster)  [unwired: 11 in, 1 out]
            }
          }
          n1307 = event shown="[0] \"Pane\": Mouse Move" {
            selector: _ -> [_ _ _]
            dyn-events: _ -> [_ _ _]
            timeout: _ -> [_ _ _]
            event Mouse Move {
              n1308 = event-data() -> ("Coords"=w1959:T6)  [unwired: 1 in]
              n1309 = local write "Real Coordinates"(w1959) -> ()
            }
            event Mouse Down {
              n1310 = event-data() -> ("Coords"=w1960:T6)  [unwired: 1 in]
              n1311 = local write "CoordinatesMousePressed"(w1960) -> ()
            }
            event "Pause Mouse/Mirror Connection": Value Change {
              n1312 = event-data() -> ()  [unwired: 1 in, 3 out]
            }
          }
          n1313 = local read "Stop"() -> (w1946:bool)
          n1314 = Not(x="Pause Mouse/Mirror Connection") -> (.not. x?=w1947:bool)
          n1315 = Or(x=w1947, y=w1946) -> (x .or. y?=w1949:bool)
        }
        n1316 = call <vilib>:"DAQmx Clear Task.vi"("task in"=w1940, "error in"=w1939) -> ("error out"=w1941:errorcluster)  [unwired: 13 in]
        n1317 = call <vilib>:"Simple Error Handler.vi"("error in (no error)"=w1941) -> ()  [unwired: 4 in, 5 out]
        n1318 = call-poly <vilib>:"Close Input Device.vi"("error in (no error)"=w1937, "device ID"=w1936) -> ("error out"=w1938:errorcluster)  [unwired: 8 in]
        n1319 = call <vilib>:"Simple Error Handler.vi"("error in (no error)"=w1938) -> ()  [unwired: 4 in, 5 out]
      }
    }
    n1320 = node-c288() -> ()  [unwired: 1 in, 1 out]
  }
  n1321 = node-c288(i64 100 ("Period")) -> (w95:T14)  [unwired: 3 in]
  n1322 = timed-loop {
    tunnel: w97 -> [w2029]
    tunnel: [w2028] -> w96
    tunnel: w100 -> [w2031]
    tunnel: [w2030] -> w99
    timing: w95 -> [_]
    timing-out: [_] -> w94
    stop <- w2027 stop-if-true
    n1323 = node-c288() -> ()  [unwired: 1 in, 1 out]
    n1324 = event shown="[1] \"Shutter 2 (A)\": Value Change" {
      selector: _ -> [_ _ _]
      dyn-events: _ -> [_ _ _]
      timeout: _ -> [_ _ _]
      tunnel: w2031 -> [w2035 _ w2072]
      tunnel: [w2034 _ w2072] -> w2030
      tunnel: w2029 -> [_ w2055 w2073]
      tunnel: [_ w2053 w2073] -> w2028
      tunnel: [_ _ w2074] -> w2027
      event "Shutter 1 (B)": Value Change {
        n1325 = event-data() -> ()  [unwired: 1 in, 1 out]
        n1326 = flat-sequence {
          tunnel: [w2041] -> w2038
          tunnel: w2035 -> [w2040]
          tunnel: [w2045] -> w2037
          tunnel: [w2048] -> w2036
          tunnel: w2038 -> [w2043]
          tunnel: w2037 -> [w2052]
          tunnel: w2036 -> [w2050]
          tunnel: [w2049] -> w2034
          frame #0 {
            n1327 = call-poly <vilib>:"DAQmx Write.vi"("task/channels in"=w2040, "data"=FALSE) -> ("task out"=w2041:refnum<k21>)  [unwired: 11 in, 2 out]
            n1328 = Wait (ms)(milliseconds to wait=100) -> ()  [unwired: 1 out]
          }
          frame #1 {
            n1329 = Or(x="Shutter 1 (B)", y=TRUE) -> (x .or. y?=w2045:bool)
            n1330 = call-poly <vilib>:"DAQmx Write.vi"("task/channels in"=w2043, "data"=w2045) -> ("task out"=w2048:refnum<k21>)  [unwired: 11 in, 2 out]
            n1331 = Wait (ms)(milliseconds to wait=100) -> ()  [unwired: 1 out]
          }
          frame #2 {
            n1332 = Not(x=w2052) -> (.not. x?=w2051:bool)
            n1333 = call-poly <vilib>:"DAQmx Write.vi"("task/channels in"=w2050, "data"=w2051) -> ("task out"=w2049:refnum<k21>)  [unwired: 11 in, 2 out]
          }
        }
      }
      event "Shutter 2 (A)": Value Change {
        n1334 = event-data() -> ()  [unwired: 1 in, 1 out]
        n1335 = flat-sequence {
          tunnel: w2055 -> [w2060]
          tunnel: [w2059] -> w2054
          tunnel: [w2064] -> w2057
          tunnel: [w2067] -> w2056
          tunnel: w2054 -> [w2062]
          tunnel: w2057 -> [w2071]
          tunnel: w2056 -> [w2069]
          tunnel: [w2068] -> w2053
          frame #0 {
            n1336 = call-poly <vilib>:"DAQmx Write.vi"("task/channels in"=w2060, "data"=FALSE) -> ("task out"=w2059:refnum<k21>)  [unwired: 11 in, 2 out]
            n1337 = Wait (ms)(milliseconds to wait=100) -> ()  [unwired: 1 out]
          }
          frame #1 {
            n1338 = Or(x="Shutter 2 (A)", y=TRUE) -> (x .or. y?=w2064:bool)
            n1339 = call-poly <vilib>:"DAQmx Write.vi"("task/channels in"=w2062, "data"=w2064) -> ("task out"=w2067:refnum<k21>)  [unwired: 11 in, 2 out]
            n1340 = Wait (ms)(milliseconds to wait=100) -> ()  [unwired: 1 out]
          }
          frame #2 {
            n1341 = Not(x=w2071) -> (.not. x?=w2070:bool)
            n1342 = call-poly <vilib>:"DAQmx Write.vi"("task/channels in"=w2069, "data"=w2070) -> ("task out"=w2068:refnum<k21>)  [unwired: 11 in, 2 out]
          }
        }
      }
      event "Stop": Value Change {
        n1343 = event-data() -> ("NewVal"=w2074:bool)  [unwired: 1 in, 5 out]
      }
    }
    n1344 = node-c288() -> ()  [unwired: 1 in, 1 out]
  }
  n1345 = node-c288(w94) -> ()  [unwired: 1 out]
  n1346 = node-c288(w81) -> ()  [unwired: 1 out]
  n1347 = call <vilib>:"DAQmx Clear Task.vi"("task in"=w96) -> ()  [unwired: 14 in, 1 out]
  n1348 = call <vilib>:"DAQmx Clear Task.vi"("task in"=w99) -> ()  [unwired: 14 in, 1 out]
  n1349 = node-c288(w33) -> ()  [unwired: 1 out]
  n1350 = node-c288(w29) -> ()  [unwired: 1 out]
  n1351 = local write "Tether"(FALSE ("Tether")) -> ()
  n1352 = local read "Path"() -> (w88:path)
  n1353 = node-c288(i64 1 ("Period"), 2 ("Processor")) -> (w93:T14)  [unwired: 2 in]
  n1354 = timed-loop {
    timing: w93 -> [_]
    timing-out: [_] -> w92
    tunnel: w88 -> [w2076]
    stop <- w2075 stop-if-true
    n1355 = node-c288() -> ()  [unwired: 1 in, 1 out]
    n1356 = event shown="[2] \"Read  Offset FFB param\": Value Change" {
      selector: _ -> [_ _ _ _ _ _ _ _ _ _ _ _]
      dyn-events: _ -> [_ _ _ _ _ _ _ _ _ _ _ _]
      timeout: _ -> [_ _ _ _ _ _ _ _ _ _ _ _]
      tunnel: w2076 -> [_ w2080 w2119 _ _ _ _ _ _ _ _ _]
      tunnel: [_ _ _ _ w2125 _ _ _ _ _ _ _] -> w2075
      event Timeout {
        n1357 = event-data() -> ()  [unwired: 1 in, 2 out]
      }
      event "Read Cal": Value Change {
        n1358 = event-data() -> ()  [unwired: 1 in, 6 out]
        n1359 = Path To String(path=w2080) -> (string=w2079:string)
        n1360 = Format Date/Time String(time format string (%c)="%y%m%d") -> (date/time string=w2081:string)  [unwired: 2 in]
        n1361 = Concatenate Strings(w2079, "\\" ("string"), w2081, "\\" ("string"), "current.cal") -> (w2099:string)
        n1362 = String To Path(string=w2099) -> (path=w2098:path)
        n1363 = Open/Create/Replace File(file path (use dialog)=w2098, operation (0:open)=T19."open", access (0:read/write)=enum16{"read/write", "read-only", "write-only"}."read-only") -> (refnum out=w2094:refnum<file>, error out=w2095:errorcluster)  [unwired: 3 in, 1 out]
        n1364 = Deny Access(4:w2095, 7:w2094) -> (0:w2093:errorcluster, 3:w2092:refnum<file>)  [unwired: 1 in]
        n1365 = Read from Binary File(5:0.0, 8:w2093, 9:T20."big-endian, network order" ("byte order (0:big-endian, network order)"), 10:12 ("count"), 11:w2092) -> (0:w2088:errorcluster, 2:w2086:dbl[], 3:w2089:refnum<file>)  [unwired: 1 in, 1 out]
        n1366 = Array To Cluster(array=w2086) -> (cluster=→"Cal values":T27)
        n1367 = Close File(refnum=w2089, error in=w2088) -> ()  [unwired: 2 out]
        n1368 = local write "Read Cal"(FALSE ("Read Cal")) -> ()
      }
      event "Read \nOffset FFB param": Value Change {
        w2116 = "\\" ("string")
        n1369 = event-data() -> ()  [unwired: 1 in, 6 out]
        n1370 = Path To String(path=w2119) -> (string=w2118:string)
        n1371 = Format Date/Time String(time format string (%c)="%y%m%d") -> (date/time string=w2117:string)  [unwired: 2 in]
        n1372 = Concatenate Strings(w2118, w2116, w2117, w2116, "current.offsetffbparam" ("string")) -> (w2114:string)
        n1373 = String To Path(string=w2114) -> (path=w2113:path)
        n1374 = Open/Create/Replace File(file path (use dialog)=w2113, operation (0:open)=T19."open", access (0:read/write)=enum16{"read/write", "read-only", "write-only"}."read-only") -> (refnum out=w2110:refnum<file>, error out=w2109:errorcluster)  [unwired: 3 in, 1 out]
        n1375 = local write "Read \nOffset FFB param"(FALSE ("Read Cal")) -> ()
        n1376 = Deny Access(4:w2109, 7:w2110) -> (0:w2107:errorcluster, 3:w2108:refnum<file>)  [unwired: 1 in]
        n1377 = Read from Binary File(5:0.0, 8:w2107, 9:T20."big-endian, network order" ("byte order (0:big-endian, network order)"), 10:15 ("count (1)"), 11:w2108) -> (0:w2105:errorcluster, 2:w2102:dbl[], 3:w2106:refnum<file>)  [unwired: 1 in, 1 out]
        n1378 = Array To Cluster(array=w2102) -> (cluster=→"offset ffb param":T28)
        n1379 = Close File(refnum=w2106, error in=w2105) -> ()  [unwired: 2 out]
      }
      event "reset offset ffb param": Value Change {
        n1380 = event-data() -> ()  [unwired: 1 in, 6 out]
        n1381 = local write "reset offset ffb param"(FALSE ("reset offset ffb param")) -> ()
        n1382 = Array To Cluster(array=dbl[] [0.0, 0.0, 0.0, 0.0, 0.0, 0.0, 0.0, 0.0, 0.0, 0.0, 0.0, 0.0, 0.0, 0.0, 10.0, 0.0, 0.0, 0.0, 0.0, 0.0, 0.0, 0.0, 0.0, 0.0, 0.0, 0.0, 0.0, 0.0, 0.0, 0.0]) -> (cluster=w2122:T29)
        n1383 = local write "offset ffb param"(w2122) -> ()
      }
      event "Stop": Value Change {
        n1384 = event-data() -> ("NewVal"=w2125:bool)  [unwired: 1 in, 5 out]
      }
      event "Trap position (V)": Value Change {
        # "Need to rotate so X and Y don't get mixed up."
        n1385 = event-data() -> ()  [unwired: 1 in, 6 out]
        n1386 = local read "Mirror task"() -> (w2126:refnum<k21>)
        n1387 = Cluster To Array(cluster="Trap position (V)") -> (array=w2129:dbl[])
        n1388 = Rotate 1D Array(1:w2129, 2:1 ("n")) -> (0:w2127:dbl[])
        n1389 = call-poly <vilib>:"DAQmx Write.vi"("task/channels in"=w2126, "data"=w2127) -> ("task out"=w2132:refnum<k21>, "error out"=w2131:errorcluster)  [unwired: 11 in, 1 out]
        n1390 = call <vilib>:"DAQmx Stop Task.vi"("task/channels in"=w2132, "error in"=w2131) -> ("error out"=w2130:errorcluster)  [unwired: 12 in, 1 out]
        n1391 = call <vilib>:"Simple Error Handler.vi"("error in (no error)"=w2130) -> ()  [unwired: 4 in, 5 out]
      }
      event "Trap delta (nm)": Value Change {
        n1392 = event-data() -> ()  [unwired: 1 in, 6 out]
        n1393 = local read "Pulling direction"() -> (w2134:bool)
        n1394 = local read "Conv Y (nm/V)"() -> (w2135:dbl)
        n1395 = local read "Conv X (nm/V)"() -> (w2136:dbl)
        n1396 = Select(t=w2135, s=w2134, f=w2136) -> (s? t:f=w2137:dbl)
        n1397 = local read "Fixed Y"() -> (w2143:dbl)
        n1398 = Divide(x="Trap delta (nm)", y=w2137) -> (x/y=w2138:dbl)
        n1399 = local read "Fixed X"() -> (w2142:dbl)
        n1400 = Select(t=w2143, s=w2134, f=w2142) -> (s? t:f=w2141:dbl)
        n1401 = Add(x=w2138, y=w2141) -> (x+y=w2139:dbl)
        n1402 = case shown="False" w2134 {
          tunnel: w2139 -> [w2144 w2145]
          frame False {
            n1403 = property on="X" class="DigNum (strict)"("Val(Sgnl)"=w2144) -> ()  [unwired: 2 in, 2 out]
          }
          frame True {
            n1404 = property on="Y" class="DigNum (strict)"("Val(Sgnl)"=w2145) -> ()  [unwired: 2 in, 2 out]
          }
        }
      }
      event "Fish": Value Change {
        n1405 = event-data() -> ()  [unwired: 1 in, 6 out]
        n1406 = local read "Fish"() -> (w2146:bool)
        n1407 = case shown="True" w2146 {
          frame False {
          }
          frame True {
            w2156 = 0.0 ("minimum value")
            w2157 = 10.0 ("maximum value")
            # "Grab offset in pulling\ndirection and add to \ndelta values"
            n1408 = call-poly <vilib>:"DAQmx Create Virtual Channel.vi"("maximum value"=w2157, "minimum value"=w2156, "physical channels"=tag "Dev1/ao0") -> ("task out"=w2161:refnum<k21>, "error out"=w2160:errorcluster)  [unwired: 11 in]
            n1409 = call-poly <vilib>:"DAQmx Create Virtual Channel.vi"("task in"=w2161, "maximum value"=w2157, "minimum value"=w2156, "physical channels"=tag "Dev1/ao1", "error in"=w2160) -> ("task out"=w2155:refnum<k21>, "error out"=w2154:errorcluster)  [unwired: 9 in]
            n1410 = node-c288(i64 1 ("Period")) -> (w2163:T14)  [unwired: 3 in]
            n1411 = timed-loop {
              timing: w2163 -> [_]
              timing-out: [_] -> w2162
              tunnel: w2155 -> [w2232]
              tunnel: w2154 -> [w2231]
              tunnel: [w2230] -> w2151
              tunnel: [w2229] -> w2150
              tunnel: [w2189] -> w2152
              tunnel: [w2190] -> w2149
              i -> [w2215]
              stop <- w2190 stop-if-true
              # "x direction"
              # "y direction"
              # "Send offset in direction\nof not-pulling to DAQ"
              n1412 = node-c288() -> ()  [unwired: 1 in, 1 out]
              n1413 = local read "Pulling direction"() -> (w2194:bool)
              n1414 = local read "Conv Y (nm/V)"() -> (w2196:dbl)
              n1415 = local read "Conv X (nm/V)"() -> (w2195:dbl)
              n1416 = local read "Fixed X"() -> (w2203:dbl)
              n1417 = local read "Fixed Y"() -> (w2202:dbl)
              n1418 = Select(t=w2202, s=w2194, f=w2203) -> (s? t:f=w2204:dbl)
              n1419 = Select(t=w2203, s=w2194, f=w2202) -> (s? t:f=w2201:dbl)
              n1420 = Select(t=w2196, s=w2194, f=w2195) -> (s? t:f=w2191:dbl)
              n1421 = Divide(x="Max fish\ndelta (nm)", y=w2191) -> (x/y=w2193:dbl)
              n1422 = Divide(x="Min fish\ndelta (nm)", y=w2191) -> (x/y=w2192:dbl)
              n1423 = Add(x=w2204, y=w2193) -> (x+y=w2206:dbl)
              n1424 = Subtract(x=w2193, y=w2192) -> (x-y=w2208:dbl)
              n1425 = Divide(x=w2208, y="Fish Speed (ms)") -> (x/y=w2209:dbl)
              n1426 = flat-sequence {
                tunnel: w2194 -> [w2252]
                tunnel: w2201 -> [w2251]
                tunnel: w2232 -> [w2250]
                tunnel: w2231 -> [w2249]
                tunnel: w2209 -> [w2248]
                tunnel: w2206 -> [w2247]
                tunnel: "Fish Speed (ms)" -> [w2242]
                tunnel: [w2246] -> w2228
                tunnel: [w2245] -> w2227
                tunnel: [w2244] -> w2226
                tunnel: [w2243] -> w2225
                tunnel: [w2236] -> w2214
                tunnel: [w2235] -> w2200
                tunnel: [w2234] -> w2197
                tunnel: [w2233] -> w2187
                tunnel: [w2305] -> w2224
                tunnel: w2228 -> [w2305]
                tunnel: [w2304] -> w2223
                tunnel: w2227 -> [w2304]
                tunnel: [w2303] -> w2222
                tunnel: w2226 -> [w2303]
                tunnel: [w2302] -> w2221
                tunnel: w2225 -> [w2302]
                tunnel: w2214 -> [w2301]
                tunnel: [w2301] -> w2213
                tunnel: w2200 -> [w2300]
                tunnel: [w2299] -> w2198
                tunnel: w2197 -> [w2299]
                tunnel: [w2298] -> w2188
                tunnel: w2187 -> [w2298]
                tunnel: w2224 -> [w2317]
                tunnel: w2223 -> [w2316]
                tunnel: w2222 -> [w2315]
                tunnel: w2221 -> [w2314]
                tunnel: w2211 -> [w2313]
                tunnel: [w2312] -> w2230
                tunnel: [w2311] -> w2229
                tunnel: w2213 -> [w2310]
                tunnel: [w2309] -> w2199
                tunnel: w2198 -> [w2308]
                tunnel: [w2307] -> w2186
                tunnel: w2188 -> [w2307]
                frame #0 {
                  n1427 = local read "Mean force (pN)"() -> (w2241:dbl)
                  n1428 = local read "Cutoff force (pN)"() -> (w2240:dbl)
                  n1429 = Less Or Equal?(x=w2241, y=w2240) -> (x <= y?=w2238:bool)
                  n1430 = And(x="Fish", y=w2238) -> (x .and. y?=w2239:bool)
                  n1431 = case shown="True" w2239 {
                    selector: w2239 -> [w2255 _]
                    tunnel: w2252 -> [w2258 w2275]
                    tunnel: w2251 -> [_ w2274]
                    tunnel: w2250 -> [w2260 w2273]
                    tunnel: w2249 -> [w2259 w2272]
                    tunnel: w2248 -> [w2257 w2271]
                    tunnel: w2247 -> [w2256 w2270]
                    tunnel: [w2260 w2269] -> w2246
                    tunnel: [w2259 w2268] -> w2245
                    tunnel: [w2258 w2267] -> w2244
                    tunnel: [w2256 w2266] -> w2234
                    tunnel: [w2257 w2265] -> w2243
                    tunnel: w2242 -> [_ w2264]
                    tunnel: [w2255 w2263] -> w2236
                    tunnel: [FALSE w2262] -> w2235
                    tunnel: [FALSE w2261] -> w2233
                    frame False {
                    }
                    frame True {
                      n1432 = while {
                        tunnel: w2275 -> [w2287]
                        tunnel: w2274 -> [w2286]
                        tunnel: w2273 -> [w2294]
                        tunnel: w2272 -> [w2293]
                        tunnel: w2271 -> [w2285]
                        tunnel: w2270 -> [w2291]
                        tunnel: [w2289] -> w2269
                        tunnel: [w2288] -> w2268
                        tunnel: [w2287] -> w2267
                        tunnel: [w2286] -> w2266
                        tunnel: [w2285] -> w2265
                        tunnel: w2264 -> [w2284]
                        tunnel: [w2277] -> w2263
                        tunnel: [w2277] -> w2262
                        tunnel: [w2276] -> w2261
                        i -> [w2283]
                        stop <- w2280 stop-if-true
                        # "top: x"
                        # "x direction"
                        # "y direction"
                        n1433 = Multiply(x=w2285, y=w2283) -> (x*y=w2292:dbl)
                        n1434 = local read "Cutoff force (pN)"() -> (w2278:dbl)
                        n1435 = local read "Mean force (pN)"() -> (w2279:dbl)
                        n1436 = Subtract(x=w2291, y=w2292) -> (x-y=w2290:dbl)
                        n1437 = Build Array(w2286, w2290) -> (w2297:dbl[])
                        n1438 = Build Array(w2290, w2286) -> (w2296:dbl[])
                        n1439 = Greater Or Equal?(x=w2283, y=w2284) -> (x >= y?=w2277:bool)
                        n1440 = Select(t=w2297, s=w2287, f=w2296) -> (s? t:f=w2295:dbl[])
                        n1441 = Greater?(x=w2279, y=w2278) -> (0:w2276:bool)
                        n1442 = local read "Fish"() -> (w2281:bool)
                        n1443 = Not(x=w2281) -> (.not. x?=w2282:bool)
                        n1444 = call-poly <vilib>:"DAQmx Write.vi"("task/channels in"=w2294, "data"=w2295, "error in"=w2293) -> ("task out"=w2289:refnum<k21>, "error out"=w2288:errorcluster)  [unwired: 10 in, 1 out]
                        n1445 = Compound Arithmetic op=OR(w2277, w2282, w2276) -> (w2280:bool)
                      }
                    }
                  }
                }
                frame #1 {
                  n1446 = case shown="True" w2300 {
                    frame False {
                    }
                    frame True {
                      n1447 = Wait (ms)(milliseconds to wait="Wait (ms)") -> ()  [unwired: 1 out]
                    }
                  }
                }
                frame #2 {
                  n1448 = case shown="True" w2310 {
                    tunnel: w2317 -> [w2320 w2329]
                    tunnel: w2316 -> [w2319 w2328]
                    tunnel: w2315 -> [_ w2327]
                    tunnel: w2314 -> [_ w2326]
                    tunnel: w2313 -> [_ w2325]
                    tunnel: [w2320 w2324] -> w2312
                    tunnel: [w2319 w2323] -> w2311
                    tunnel: [FALSE w2322] -> w2309
                    tunnel: w2308 -> [_ w2321]
                    frame False {
                    }
                    frame True {
                      n1449 = while {
                        tunnel: w2329 -> [w2361]
                        tunnel: w2328 -> [w2360]
                        tunnel: w2327 -> [w2332]
                        tunnel: w2326 -> [w2358]
                        tunnel: w2325 -> [w2357]
                        tunnel: [w2355] -> w2324
                        tunnel: [w2354] -> w2323
                        tunnel: [w2339] -> w2322
                        tunnel: w2321 -> [w2330]
                        i -> [w2346]
                        stop <- w2351 stop-if-true
                        # "y direction"
                        # "If tether formed,\nimmediately change\nto new delta."
                        n1450 = local read "Conv Y (nm/V)"() -> (w2333:dbl)
                        n1451 = local read "Conv X (nm/V)"() -> (w2331:dbl)
                        n1452 = local read "Fixed Y"() -> (w2340:dbl)
                        n1453 = local read "Fixed X"() -> (w2345:dbl)
                        n1454 = Select(t=w2333, s=w2332, f=w2331) -> (s? t:f=w2334:dbl)
                        n1455 = local read "Cutoff force (pN)"() -> (w2347:dbl)
                        n1456 = Divide(x="Delta after tether", y=w2334) -> (x/y=w2335:dbl)
                        n1457 = Multiply(x=w2358, y=w2346) -> (x*y=w2359:dbl)
                        n1458 = local read "Mean force (pN)"() -> (w2348:dbl)
                        n1459 = Add(x=w2357, y=w2359) -> (x+y=w2342:dbl)
                        n1460 = Select(t=w2340, s=w2332, f=w2345) -> (s? t:f=w2344:dbl)
                        n1461 = Greater?(x=w2348, y=w2347) -> (0:w2339:bool)
                        n1462 = Add(x=w2344, y=w2335) -> (x+y=w2343:dbl)
                        n1463 = Select(t=w2343, s=w2339, f=w2342) -> (s? t:f=w2341:dbl)
                        n1464 = local read "Fish Speed (ms)"() -> (w2353:i32)
                        n1465 = Build Array(w2330, w2341) -> (w2356:dbl[])
                        n1466 = Build Array(w2341, w2330) -> (w2337:dbl[])
                        n1467 = Select(t=w2356, s=w2332, f=w2337) -> (s? t:f=w2336:dbl[])
                        n1468 = case shown="True" w2339 {
                          tunnel: w2335 -> [_ _]
                          tunnel: w2336 -> [_ w2363]
                          frame False {
                          }
                          frame True {
                            n1469 = Array To Cluster(array=w2363) -> (cluster=w2362:cluster{"[0]":dbl, "[1]":dbl})
                            n1470 = property on="Trap position (V)" class="Clust (strict)"("Val(Sgnl)"=w2362) -> ()  [unwired: 2 in, 2 out]
                          }
                        }
                        n1471 = local read "Fish"() -> (w2350:bool)
                        n1472 = Greater Or Equal?(x=w2346, y=w2353) -> (x >= y?=w2352:bool)
                        n1473 = Not(x=w2350) -> (.not. x?=w2349:bool)
                        n1474 = call-poly <vilib>:"DAQmx Write.vi"("task/channels in"=w2361, "data"=w2336, "error in"=w2360) -> ("task out"=w2355:refnum<k21>, "error out"=w2354:errorcluster)  [unwired: 10 in, 1 out]
                        n1475 = Compound Arithmetic op=OR(w2352, w2349, w2339) -> (w2351:bool)
                      }
                    }
                  }
                }
              }
              n1476 = Add(x=w2204, y=w2192) -> (x+y=w2211:dbl)
              n1477 = Decrement(x="# attempts") -> (x-1=w2219:dbl)
              n1478 = Greater Or Equal?(x=w2215, y=w2219) -> (x >= y?=w2218:bool)
              n1479 = local read "Mean force (pN)"() -> (w2217:dbl)
              n1480 = Greater?(x=w2217, y="Cutoff force (pN)") -> (0:w2212:bool)
              n1481 = Compound Arithmetic op=OR(w2186, w2199, w2212, w2218) -> (w2190:bool)
              n1482 = Or(x=w2199, y=w2186) -> (x .or. y?=w2189:bool)
              "Tether" <- w2189
              n1483 = case shown="True" w2189 {
                frame False {
                }
                frame True {
                  n1484 = call <vilib>:"Beep.vi"() -> ()  [unwired: 12 in]
                }
              }
              n1485 = node-c288() -> ()  [unwired: 1 in, 1 out]
              "Attempt #" <- w2215
            }
            n1486 = node-c288(w2162) -> ()  [unwired: 1 out]
            n1487 = flat-sequence {
              tunnel: w2152 -> [w2170]
              tunnel: [w2170] -> w2148
              tunnel: w2151 -> [w2167]
              tunnel: w2150 -> [w2166]
              tunnel: w2149 -> [w2164]
              tunnel: w2148 -> [w2172]
              tunnel: [w2172] -> w2147
              tunnel: w2147 -> [w2174]
              frame #0 {
                w2169 = T25 1 items=["no dialog", "OK message", "continue or stop message", "OK message + warnings", "continue/stop + warnings"] ("type of dialog (OK msg:1)")
                n1488 = call <vilib>:"DAQmx Clear Task.vi"("task in"=w2167, "error in"=w2166) -> ("error out"=w2168:errorcluster)  [unwired: 13 in]
                n1489 = Not(x=w2164) -> (.not. x?=w2165:bool)
                n1490 = local write "Fish"(w2165) -> ()
                n1491 = call <vilib>:"Simple Error Handler.vi"("type of dialog (OK msg:1)"=w2169, "error in (no error)"=w2168) -> ()  [unwired: 3 in, 5 out]
              }
              frame #1 {
                n1492 = Wait (ms)(milliseconds to wait=u32 500) -> ()  [unwired: 1 out]
              }
              frame #2 {
                n1493 = And(x=w2174, y="Raster after\n tether?") -> (x .and. y?=w2175:bool)
                n1494 = case shown="True" w2175 {
                  selector: w2175 -> [_ w2176]
                  frame False {
                  }
                  frame True {
                    n1495 = stacked-sequence {
                      tunnel: w2176 -> [_ _ w2183 _ w2185]
                      frame #0 {
                        n1496 = Replace Array Subset(array=i32[] [0], new element="Raster set", index=0) -> (w2178:i32[])
                        n1497 = property on="Scan Parameters" class="Arr (strict)"("Index Values"=w2178) -> ()  [unwired: 2 in, 2 out]
                        n1498 = property on="Inject Sample" class="Bool (strict)"("Val(Sgnl)"=FALSE ("Value (Signaling)")) -> ()  [unwired: 2 in, 2 out]
                      }
                      frame #1 {
                        n1499 = Wait (ms)(milliseconds to wait=u32 500) -> ()  [unwired: 1 out]
                      }
                      frame #2 {
                        n1500 = property on="Load param" class="Bool (strict)"("Val(Sgnl)"=w2183) -> ()  [unwired: 2 in, 2 out]
                      }
                      frame #3 {
                        n1501 = Wait (ms)(milliseconds to wait=u32 500) -> ()  [unwired: 1 out]
                      }
                      frame #4 {
                        n1502 = property on="Raster scan" class="Bool (strict)"("Val(Sgnl)"=w2185) -> ()  [unwired: 2 in, 2 out]
                      }
                    }
                  }
                }
              }
            }
          }
        }
      }
      event "Load param": Value Change {
        n1503 = event-data() -> ()  [unwired: 1 in, 6 out]
        n1504 = property on="Scan Parameters" class="Arr (strict)"() -> ("Index Values"=w2379:u32[])  [unwired: 2 in, 2 out]
        n1505 = Index Array(array=w2379, index=0) -> (element=w2376:u32)
        n1506 = Index Array(array="Scan Parameters", index=w2376) -> (element=w2375:T30)
        n1507 = Unbundle(w2375) -> ("Scan range 1"=w2370:dbl, "Step size 1"=w2371:dbl, "Scan speed 1"=w2373:i32, "# scans 2"=w2372:i32)  [unwired: 1 out]
        n1508 = flat-sequence {
          tunnel: w2372 -> [w2382]
          tunnel: w2371 -> [w2380]
          tunnel: w2370 -> [w2381]
          tunnel: w2373 -> [w2384]
          frame #0 {
            n1509 = property on="# scans" class="DigNum (strict)"("Val(Sgnl)"=w2382) -> ()  [unwired: 2 in, 2 out]
            n1510 = property on="Scan range (nm)" class="DigNum (strict)"("Val(Sgnl)"=w2381) -> ()  [unwired: 2 in, 2 out]
            n1511 = property on="Step size (nm)" class="DigNum (strict)"("Val(Sgnl)"=w2380) -> ()  [unwired: 2 in, 2 out]
          }
          frame #1 {
            n1512 = Wait (ms)(milliseconds to wait=u32 500) -> ()  [unwired: 1 out]
          }
          frame #2 {
            n1513 = property on="Scan speed (nm/s)" class="DigNum (strict)"("Val(Sgnl)"=w2384) -> ()  [unwired: 2 in, 2 out]
          }
        }
        n1514 = local write "Load param"(FALSE ("Load param")) -> ()
      }
      event "# scans", "Scan range (nm)", "Step size (nm)", "Scan speed (nm/s)": Value Change {
        n1515 = event-data() -> ()  [unwired: 1 in, 6 out]
        n1516 = local read "Pulling direction"() -> (w2415:bool)
        n1517 = Reciprocal(x="Scan speed (nm/s)") -> (1/x=w2407:dbl)
        n1518 = local read "Conv Y (nm/V)"() -> (w2413:dbl)
        n1519 = local read "Conv X (nm/V)"() -> (w2414:dbl)
        n1520 = Multiply(x="Step size (nm)", y=w2407) -> (x*y=w2405:dbl)
        n1521 = Divide(x="Scan range (nm)", y="Step size (nm)") -> (x/y=w2412:dbl)
        n1522 = Absolute Value(x=w2412) -> (abs(x)=w2411:dbl)
        n1523 = Multiply(x=w2405, y=1000.0) -> (x*y=w2392:dbl)
        n1524 = Select(t=w2413, s=w2415, f=w2414) -> (s? t:f=w2403:dbl)
        n1525 = Multiply(x="# scans", y=2) -> (x*y=w2391:i32)
        n1526 = To Unsigned Quad Integer(1:w2411) -> (0:w2401:u64)
        "Scan steps (mirror)" <- w2401
        n1527 = Divide(x="Scan range (nm)", y=w2403) -> (x/y=→"Scan range (V)":dbl)
        n1528 = Multiply(x=w2401, y=w2392) -> (x*y=w2400:dbl)
        n1529 = Divide(x="Step size (nm)", y=w2403) -> (x/y=→"Scan increment (V)":dbl)
        n1530 = Round Toward +Infinity(x=w2392) -> (ceil(x): smallest int >= x=w2389:dbl)
        "Time per step (ms)" <- w2389
        n1531 = local read "Data update period (s/set)"() -> (w2395:dbl)
        n1532 = Multiply(x=w2391, y=w2400) -> (x*y=w2398:dbl)
        n1533 = Divide(x=w2398, y=1000.0) -> (x/y=w2396:dbl)
        "Total raster time (s)" <- w2396
        n1534 = local read "Data update period (s/set)"() -> (w2387:dbl)
        n1535 = Divide(x=w2396, y=w2395) -> (x/y=w2394:dbl)
        n1536 = Round Toward -Infinity(1:w2394) -> (0:→"N sets to be saved":dbl)
        n1537 = Multiply(x=w2387, y=1000.0) -> (x*y=w2385:dbl)
        n1538 = Less?(x=w2389, y=w2385) -> (x < y?=w2388:bool)
        n1539 = case shown="True" w2388 {
          selector: w2388 -> [_ w2416]
          frame False {
          }
          frame True {
            n1540 = call "Display Message to User"("Enable"=w2416) -> ()  [unwired: 9 in, 2 out]
          }
        }
      }
      event "Pulling direction": Value Change {
        n1541 = event-data() -> ()  [unwired: 1 in, 6 out]
        n1542 = local read "Pulling direction"() -> (w2422:bool)
        n1543 = local read "Conv Y (nm/V)"() -> (w2424:dbl)
        n1544 = local read "Conv X (nm/V)"() -> (w2423:dbl)
        n1545 = local read "Scan range (nm)"() -> (w2421:dbl)
        n1546 = Select(t=w2424, s=w2422, f=w2423) -> (s? t:f=w2418:dbl)
        n1547 = local read "Step size (nm)"() -> (w2419:dbl)
        n1548 = case shown="False" w2422 {
          frame False {
            n1549 = local read "Fixed Y"() -> (w2427:dbl)
            n1550 = local read "Trap delta (nm)"() -> (w2432:dbl)
            n1551 = local read "Conv X (nm/V)"() -> (w2431:dbl)
            n1552 = local read "Fixed X"() -> (w2429:dbl)
            n1553 = Divide(x=w2432, y=w2431) -> (x/y=w2430:dbl)
            n1554 = Add(x=w2430, y=w2429) -> (x+y=w2428:dbl)
            n1555 = Build Array(w2428, w2427) -> (w2426:dbl[])
            n1556 = Array To Cluster(array=w2426) -> (cluster=w2425:cluster{"[0]":dbl, "[1]":dbl})
            n1557 = property on="Trap position (V)" class="Clust (strict)"("Val(Sgnl)"=w2425) -> ()  [unwired: 2 in, 2 out]
          }
          frame True {
            n1558 = local read "Trap delta (nm)"() -> (w2440:dbl)
            n1559 = local read "Conv Y (nm/V)"() -> (w2439:dbl)
            n1560 = local read "Fixed X"() -> (w2435:dbl)
            n1561 = local read "Fixed Y"() -> (w2437:dbl)
            n1562 = Divide(x=w2440, y=w2439) -> (x/y=w2438:dbl)
            n1563 = Add(x=w2438, y=w2437) -> (x+y=w2436:dbl)
            n1564 = Build Array(w2435, w2436) -> (w2434:dbl[])
            n1565 = Array To Cluster(array=w2434) -> (cluster=w2433:cluster{"[0]":dbl, "[1]":dbl})
            n1566 = property on="Trap position (V)" class="Clust (strict)"("Val(Sgnl)"=w2433) -> ()  [unwired: 2 in, 2 out]
          }
        }
        n1567 = Divide(x=w2421, y=w2418) -> (x/y=w2420:dbl)
        n1568 = Divide(x=w2419, y=w2418) -> (x/y=w2417:dbl)
        n1569 = local write "Scan range (V)"(w2420) -> ()
        n1570 = local write "Scan increment (V)"(w2417) -> ()
      }
      event "Averaging Number": Value Change {
        n1571 = event-data() -> ()  [unwired: 1 in, 6 out]
        n1572 = local read "# Samples/channel (in)"() -> (w2444:i32)
        n1573 = local read "Averaging Number"() -> (w2442:i32)
        n1574 = Quotient & Remainder(x=w2444, y=w2442) -> (floor(x/y)=w2443:i32)  [unwired: 1 out]
        n1575 = Multiply(x=w2443, y=w2442) -> (x*y=w2441:i32)
        n1576 = local write "# Samples/channel (in)"(w2441) -> ()
      }
    }
    n1577 = node-c288() -> ()  [unwired: 1 in, 1 out]
  }
  n1578 = VISA Close(VISA resource name=w27) -> (error out=w105:errorcluster)  [unwired: 1 in]
  n1579 = call <vilib>:"Simple Error Handler.vi"("error in (no error)"=w105) -> ()  [unwired: 4 in, 5 out]
  n1580 = disable-structure shown="Enabled" {
    frame Disabled {
      n1581 = node-c288(2 ("Processor")) -> (w2450:T14)  [unwired: 3 in]
      n1582 = timed-loop "Pump Control" {
        timing: w2450 -> [_]
        timing-out: [_] -> w2449
        tunnel: refnum<visa-resource-name> "COM6" ("VISA resource name") -> [w2452]
        stop <- w2451 stop-if-true
        n1583 = node-c288() -> ()  [unwired: 1 in, 1 out]
        n1584 = event shown="[2] \"Stop\": Value Change" {
          selector: _ -> [_ _ _ _ _ _ _ _ _]
          dyn-events: _ -> [_ _ _ _ _ _ _ _ _]
          timeout: _ -> [_ _ _ _ _ _ _ _ _]
          tunnel: w2452 -> [w2460 w2556 _ w2632 w2760 w2903 w2948 w3006 w3065]
          tunnel: [_ _ w2631 _ _ _ _ _ _] -> w2451
          event "Flush Pump 1": Value Change {
            w2461 = "\r"
            n1585 = event-data() -> ()  [unwired: 1 in, 5 out]
            n1586 = call-poly "VISA Configure Serial Port"("VISA resource name"=w2460) -> ("VISA resource name out"=w2474:refnum<visa-resource-name>, "error out"=w2475:errorcluster)  [unwired: 13 in]
            n1587 = local read "Write Wait"() -> (w2453:i32)
            n1588 = Concatenate Strings("enter pump1", w2461) -> (w2462:string)
            n1589 = flat-sequence {
              tunnel: w2475 -> [w2494]
              tunnel: w2474 -> [w2496]
              tunnel: [w2495] -> w2491
              tunnel: [w2493] -> w2490
              tunnel: w2462 -> [w2492]
              tunnel: w2491 -> [w2499]
              tunnel: [w2499] -> w2489
              tunnel: w2490 -> [w2498]
              tunnel: [w2498] -> w2488
              tunnel: w2453 -> [w2497]
              tunnel: [w2504] -> w2487
              tunnel: w2467 -> [w2503]
              tunnel: [w2500] -> w2486
              tunnel: w2489 -> [w2502]
              tunnel: w2488 -> [w2501]
              tunnel: w2487 -> [w2507]
              tunnel: [w2507] -> w2485
              tunnel: [w2506] -> w2484
              tunnel: w2486 -> [w2506]
              tunnel: w2453 -> [w2505]
              tunnel: w2485 -> [w2512]
              tunnel: [w2511] -> w2483
              tunnel: w2470 -> [w2510]
              tunnel: w2484 -> [w2509]
              tunnel: [w2508] -> w2482
              tunnel: w2483 -> [w2515]
              tunnel: [w2515] -> w2481
              tunnel: [w2514] -> w2480
              tunnel: w2482 -> [w2514]
              tunnel: w2453 -> [w2513]
              tunnel: w2481 -> [w2520]
              tunnel: [w2519] -> w2479
              tunnel: w2473 -> [w2518]
              tunnel: w2480 -> [w2517]
              tunnel: [w2516] -> w2478
              tunnel: [w2523] -> w2477
              tunnel: w2479 -> [w2523]
              tunnel: [w2522] -> w2476
              tunnel: w2478 -> [w2522]
              tunnel: w2453 -> [w2521]
              tunnel: w2477 -> [w2528]
              tunnel: w2476 -> [w2525]
              tunnel: [w2527] -> w2456
              tunnel: [w2526] -> w2454
              tunnel: [w2533] -> w2457
              tunnel: w2456 -> [w2533]
              tunnel: [w2532] -> w2455
              tunnel: w2454 -> [w2532]
              tunnel: w2453 -> [w2531]
              tunnel: w2457 -> [w2535]
              tunnel: w2455 -> [w2534]
              frame #0 {
                n1590 = VISA Write(VISA resource name=w2496, write buffer=w2492, error in (no error)=w2494) -> (VISA resource name out=w2495:refnum<visa-resource-name>, error out=w2493:errorcluster)  [unwired: 1 out]
              }
              frame #1 {
                n1591 = Wait (ms)(milliseconds to wait=w2497) -> ()  [unwired: 1 out]
              }
              frame #2 {
                n1592 = VISA Write(VISA resource name=w2502, write buffer=w2503, error in (no error)=w2501) -> (VISA resource name out=w2504:refnum<visa-resource-name>, error out=w2500:errorcluster)  [unwired: 1 out]
              }
              frame #3 {
                n1593 = Wait (ms)(milliseconds to wait=w2505) -> ()  [unwired: 1 out]
              }
              frame #4 {
                n1594 = VISA Write(VISA resource name=w2512, write buffer=w2510, error in (no error)=w2509) -> (VISA resource name out=w2511:refnum<visa-resource-name>, error out=w2508:errorcluster)  [unwired: 1 out]
              }
              frame #5 {
                n1595 = Wait (ms)(milliseconds to wait=w2513) -> ()  [unwired: 1 out]
              }
              frame #6 {
                n1596 = VISA Write(VISA resource name=w2520, write buffer=w2518, error in (no error)=w2517) -> (VISA resource name out=w2519:refnum<visa-resource-name>, error out=w2516:errorcluster)  [unwired: 1 out]
              }
              frame #7 {
                n1597 = Wait (ms)(milliseconds to wait=w2521) -> ()  [unwired: 1 out]
              }
              frame #8 {
                n1598 = Concatenate Strings("start ", "\r") -> (w2524:string)
                n1599 = VISA Write(VISA resource name=w2528, write buffer=w2524, error in (no error)=w2525) -> (VISA resource name out=w2527:refnum<visa-resource-name>, error out=w2526:errorcluster)  [unwired: 1 out]
              }
              frame #9 {
                n1600 = Wait (ms)(milliseconds to wait=w2531) -> ()  [unwired: 1 out]
              }
              frame #10 {
                n1601 = local write "Flush Pump 1"(FALSE ("Flush Pump 1")) -> ()
                n1602 = Concatenate Strings("enter main ", "\r") -> (w2539:string)
                n1603 = VISA Write(VISA resource name=w2535, write buffer=w2539, error in (no error)=w2534) -> (VISA resource name out=w2538:refnum<visa-resource-name>, error out=w2537:errorcluster)  [unwired: 1 out]
                n1604 = VISA Close(VISA resource name=w2538, error in (no error)=w2537) -> ()  [unwired: 1 out]
              }
            }
            n1605 = Concatenate Strings("set units 4 ", w2461) -> (w2467:string)
            n1606 = Multiply(x="Flush\nRate (ul/min)", y=60) -> (x*y=w2465:dbl)
            n1607 = Number To Decimal String(number=w2465) -> (decimal integer string=w2468:string)  [unwired: 1 in]
            n1608 = Concatenate Strings("set rate ", w2468, w2461) -> (w2470:string)
            n1609 = Number To Decimal String(number="Flush\nVolume (ul)") -> (decimal integer string=w2472:string)  [unwired: 1 in]
            n1610 = Concatenate Strings("set volume ", w2472, w2461) -> (w2473:string)
          }
          event "Flush Pump 2": Value Change {
            w2547 = "\r"
            n1611 = event-data() -> ()  [unwired: 1 in, 5 out]
            n1612 = call-poly "VISA Configure Serial Port"("VISA resource name"=w2556) -> ("VISA resource name out"=w2567:refnum<visa-resource-name>, "error out"=w2568:errorcluster)  [unwired: 13 in]
            n1613 = local read "Write Wait"() -> (w2542:i32)
            n1614 = Concatenate Strings("enter pump2", w2547) -> (w2548:string)
            n1615 = flat-sequence {
              tunnel: w2568 -> [w2583]
              tunnel: w2567 -> [w2585]
              tunnel: [w2584] -> w2553
              tunnel: [w2582] -> w2551
              tunnel: w2548 -> [w2581]
              tunnel: w2553 -> [w2588]
              tunnel: [w2588] -> w2552
              tunnel: w2551 -> [w2587]
              tunnel: [w2587] -> w2550
              tunnel: w2542 -> [w2586]
              tunnel: [w2593] -> w2580
              tunnel: w2560 -> [w2592]
              tunnel: [w2589] -> w2579
              tunnel: w2552 -> [w2591]
              tunnel: w2550 -> [w2590]
              tunnel: w2580 -> [w2596]
              tunnel: [w2596] -> w2578
              tunnel: [w2595] -> w2577
              tunnel: w2579 -> [w2595]
              tunnel: w2542 -> [w2594]
              tunnel: w2578 -> [w2601]
              tunnel: [w2600] -> w2576
              tunnel: w2563 -> [w2599]
              tunnel: w2577 -> [w2598]
              tunnel: [w2597] -> w2575
              tunnel: w2576 -> [w2604]
              tunnel: [w2604] -> w2574
              tunnel: [w2603] -> w2573
              tunnel: w2575 -> [w2603]
              tunnel: w2542 -> [w2602]
              tunnel: w2574 -> [w2609]
              tunnel: [w2608] -> w2572
              tunnel: w2566 -> [w2607]
              tunnel: w2573 -> [w2606]
              tunnel: [w2605] -> w2571
              tunnel: [w2612] -> w2570
              tunnel: w2572 -> [w2612]
              tunnel: [w2611] -> w2569
              tunnel: w2571 -> [w2611]
              tunnel: w2542 -> [w2610]
              tunnel: w2570 -> [w2619]
              tunnel: w2569 -> [w2618]
              tunnel: [w2614] -> w2546
              tunnel: [w2613] -> w2544
              tunnel: w2546 -> [w2622]
              tunnel: [w2622] -> w2545
              tunnel: w2544 -> [w2621]
              tunnel: [w2621] -> w2543
              tunnel: w2542 -> [w2620]
              tunnel: w2545 -> [w2626]
              tunnel: w2543 -> [w2625]
              frame #0 {
                n1616 = VISA Write(VISA resource name=w2585, write buffer=w2581, error in (no error)=w2583) -> (VISA resource name out=w2584:refnum<visa-resource-name>, error out=w2582:errorcluster)  [unwired: 1 out]
              }
              frame #1 {
                n1617 = Wait (ms)(milliseconds to wait=w2586) -> ()  [unwired: 1 out]
              }
              frame #2 {
                n1618 = VISA Write(VISA resource name=w2591, write buffer=w2592, error in (no error)=w2590) -> (VISA resource name out=w2593:refnum<visa-resource-name>, error out=w2589:errorcluster)  [unwired: 1 out]
              }
              frame #3 {
                n1619 = Wait (ms)(milliseconds to wait=w2594) -> ()  [unwired: 1 out]
              }
              frame #4 {
                n1620 = VISA Write(VISA resource name=w2601, write buffer=w2599, error in (no error)=w2598) -> (VISA resource name out=w2600:refnum<visa-resource-name>, error out=w2597:errorcluster)  [unwired: 1 out]
              }
              frame #5 {
                n1621 = Wait (ms)(milliseconds to wait=w2602) -> ()  [unwired: 1 out]
              }
              frame #6 {
                n1622 = VISA Write(VISA resource name=w2609, write buffer=w2607, error in (no error)=w2606) -> (VISA resource name out=w2608:refnum<visa-resource-name>, error out=w2605:errorcluster)  [unwired: 1 out]
              }
              frame #7 {
                n1623 = Wait (ms)(milliseconds to wait=w2610) -> ()  [unwired: 1 out]
              }
              frame #8 {
                n1624 = Concatenate Strings("start ", "\r") -> (w2617:string)
                n1625 = VISA Write(VISA resource name=w2619, write buffer=w2617, error in (no error)=w2618) -> (VISA resource name out=w2614:refnum<visa-resource-name>, error out=w2613:errorcluster)  [unwired: 1 out]
              }
              frame #9 {
                n1626 = Wait (ms)(milliseconds to wait=w2620) -> ()  [unwired: 1 out]
              }
              frame #10 {
                n1627 = local write "Flush Pump 2"(FALSE ("Flush Pump 1")) -> ()
                n1628 = Concatenate Strings("enter main ", "\r") -> (w2627:string)
                n1629 = VISA Write(VISA resource name=w2626, write buffer=w2627, error in (no error)=w2625) -> (VISA resource name out=w2624:refnum<visa-resource-name>, error out=w2623:errorcluster)  [unwired: 1 out]
                n1630 = VISA Close(VISA resource name=w2624, error in (no error)=w2623) -> ()  [unwired: 1 out]
              }
            }
            n1631 = Concatenate Strings("set units 4 ", w2547) -> (w2560:string)
            n1632 = Multiply(x="Flush \nRate (ul/min)  2", y=60) -> (x*y=w2558:dbl)
            n1633 = Number To Decimal String(number=w2558) -> (decimal integer string=w2561:string)  [unwired: 1 in]
            n1634 = Concatenate Strings("set rate ", w2561, w2547) -> (w2563:string)
            n1635 = Number To Decimal String(number="Flush\nVolume (ul)  2") -> (decimal integer string=w2565:string)  [unwired: 1 in]
            n1636 = Concatenate Strings("set volume ", w2565, w2547) -> (w2566:string)
          }
          event "Stop": Value Change {
            n1637 = event-data() -> ()  [unwired: 1 in, 5 out]
            n1638 = local read "Stop"() -> (w2631:bool)
          }
          event "Inject Pump 2": Value Change {
            n1639 = event-data() -> ()  [unwired: 1 in, 5 out]
            n1640 = case shown="True" "Inject Pump 2" {
              tunnel: w2632 -> [w2635 w2677]
              frame False {
                n1641 = local read "Write Wait"() -> (w2634:i32)
                n1642 = call-poly "VISA Configure Serial Port"("VISA resource name"=w2635) -> ("VISA resource name out"=w2639:refnum<visa-resource-name>, "error out"=w2640:errorcluster)  [unwired: 13 in]
                n1643 = Concatenate Strings("enter pump2", "\r") -> (w2637:string)
                n1644 = flat-sequence {
                  tunnel: w2640 -> [w2651]
                  tunnel: w2639 -> [w2653]
                  tunnel: [w2652] -> w2648
                  tunnel: [w2650] -> w2647
                  tunnel: w2637 -> [w2649]
                  tunnel: w2648 -> [w2656]
                  tunnel: w2647 -> [w2655]
                  tunnel: [w2656] -> w2646
                  tunnel: [w2655] -> w2645
                  tunnel: w2634 -> [w2654]
                  tunnel: [w2660] -> w2644
                  tunnel: [w2659] -> w2643
                  tunnel: w2646 -> [w2658]
                  tunnel: w2645 -> [w2657]
                  tunnel: w2644 -> [w2666]
                  tunnel: [w2666] -> w2642
                  tunnel: w2643 -> [w2665]
                  tunnel: [w2665] -> w2641
                  tunnel: w2634 -> [w2664]
                  tunnel: w2642 -> [w2670]
                  tunnel: w2641 -> [w2669]
                  frame #0 {
                    n1645 = VISA Write(VISA resource name=w2653, write buffer=w2649, error in (no error)=w2651) -> (VISA resource name out=w2652:refnum<visa-resource-name>, error out=w2650:errorcluster)  [unwired: 1 out]
                  }
                  frame #1 {
                    n1646 = Wait (ms)(milliseconds to wait=w2654) -> ()  [unwired: 1 out]
                  }
                  frame #2 {
                    n1647 = Concatenate Strings("stop ", "\r") -> (w2663:string)
                    n1648 = VISA Write(VISA resource name=w2658, write buffer=w2663, error in (no error)=w2657) -> (VISA resource name out=w2660:refnum<visa-resource-name>, error out=w2659:errorcluster)  [unwired: 1 out]
                  }
                  frame #3 {
                    n1649 = Wait (ms)(milliseconds to wait=w2664) -> ()  [unwired: 1 out]
                  }
                  frame #4 {
                    n1650 = Concatenate Strings("enter main ", "\r") -> (w2671:string)
                    n1651 = VISA Write(VISA resource name=w2670, write buffer=w2671, error in (no error)=w2669) -> (VISA resource name out=w2668:refnum<visa-resource-name>, error out=w2667:errorcluster)  [unwired: 1 out]
                    n1652 = VISA Close(VISA resource name=w2668, error in (no error)=w2667) -> ()  [unwired: 1 out]
                  }
                }
              }
              frame True {
                w2690 = "\r"
                n1653 = call-poly "VISA Configure Serial Port"("VISA resource name"=w2677) -> ("VISA resource name out"=w2679:refnum<visa-resource-name>, "error out"=w2678:errorcluster)  [unwired: 13 in]
                n1654 = local read "Write Wait"() -> (w2674:i32)
                n1655 = Concatenate Strings("enter pump2", w2690) -> (w2689:string)
                n1656 = flat-sequence {
                  tunnel: w2678 -> [w2713]
                  tunnel: w2679 -> [w2715]
                  tunnel: [w2714] -> w2710
                  tunnel: [w2712] -> w2709
                  tunnel: w2689 -> [w2711]
                  tunnel: w2710 -> [w2718]
                  tunnel: [w2718] -> w2708
                  tunnel: w2709 -> [w2717]
                  tunnel: [w2717] -> w2707
                  tunnel: w2674 -> [w2716]
                  tunnel: [w2723] -> w2706
                  tunnel: w2686 -> [w2722]
                  tunnel: [w2719] -> w2705
                  tunnel: w2708 -> [w2721]
                  tunnel: w2707 -> [w2720]
                  tunnel: w2706 -> [w2726]
                  tunnel: [w2726] -> w2704
                  tunnel: [w2725] -> w2703
                  tunnel: w2705 -> [w2725]
                  tunnel: w2674 -> [w2724]
                  tunnel: w2704 -> [w2731]
                  tunnel: [w2730] -> w2702
                  tunnel: w2683 -> [w2729]
                  tunnel: w2703 -> [w2728]
                  tunnel: [w2727] -> w2701
                  tunnel: w2702 -> [w2734]
                  tunnel: [w2734] -> w2700
                  tunnel: [w2733] -> w2699
                  tunnel: w2701 -> [w2733]
                  tunnel: w2674 -> [w2732]
                  tunnel: w2700 -> [w2739]
                  tunnel: [w2738] -> w2698
                  tunnel: w2680 -> [w2737]
                  tunnel: w2699 -> [w2736]
                  tunnel: [w2735] -> w2697
                  tunnel: [w2742] -> w2696
                  tunnel: w2698 -> [w2742]
                  tunnel: [w2741] -> w2695
                  tunnel: w2697 -> [w2741]
                  tunnel: w2674 -> [w2740]
                  tunnel: w2696 -> [w2749]
                  tunnel: w2695 -> [w2748]
                  tunnel: [w2744] -> w2694
                  tunnel: [w2743] -> w2693
                  tunnel: w2694 -> [w2752]
                  tunnel: [w2752] -> w2692
                  tunnel: w2693 -> [w2751]
                  tunnel: [w2751] -> w2691
                  tunnel: w2674 -> [w2750]
                  tunnel: w2692 -> [w2756]
                  tunnel: w2691 -> [w2755]
                  frame #0 {
                    n1657 = VISA Write(VISA resource name=w2715, write buffer=w2711, error in (no error)=w2713) -> (VISA resource name out=w2714:refnum<visa-resource-name>, error out=w2712:errorcluster)  [unwired: 1 out]
                  }
                  frame #1 {
                    n1658 = Wait (ms)(milliseconds to wait=w2716) -> ()  [unwired: 1 out]
                  }
                  frame #2 {
                    n1659 = VISA Write(VISA resource name=w2721, write buffer=w2722, error in (no error)=w2720) -> (VISA resource name out=w2723:refnum<visa-resource-name>, error out=w2719:errorcluster)  [unwired: 1 out]
                  }
                  frame #3 {
                    n1660 = Wait (ms)(milliseconds to wait=w2724) -> ()  [unwired: 1 out]
                  }
                  frame #4 {
                    n1661 = VISA Write(VISA resource name=w2731, write buffer=w2729, error in (no error)=w2728) -> (VISA resource name out=w2730:refnum<visa-resource-name>, error out=w2727:errorcluster)  [unwired: 1 out]
                  }
                  frame #5 {
                    n1662 = Wait (ms)(milliseconds to wait=w2732) -> ()  [unwired: 1 out]
                  }
                  frame #6 {
                    n1663 = VISA Write(VISA resource name=w2739, write buffer=w2737, error in (no error)=w2736) -> (VISA resource name out=w2738:refnum<visa-resource-name>, error out=w2735:errorcluster)  [unwired: 1 out]
                  }
                  frame #7 {
                    n1664 = Wait (ms)(milliseconds to wait=w2740) -> ()  [unwired: 1 out]
                  }
                  frame #8 {
                    n1665 = Concatenate Strings("start ", "\r") -> (w2747:string)
                    n1666 = VISA Write(VISA resource name=w2749, write buffer=w2747, error in (no error)=w2748) -> (VISA resource name out=w2744:refnum<visa-resource-name>, error out=w2743:errorcluster)  [unwired: 1 out]
                  }
                  frame #9 {
                    n1667 = Wait (ms)(milliseconds to wait=w2750) -> ()  [unwired: 1 out]
                  }
                  frame #10 {
                    n1668 = Concatenate Strings("enter main ", "\r") -> (w2757:string)
                    n1669 = VISA Write(VISA resource name=w2756, write buffer=w2757, error in (no error)=w2755) -> (VISA resource name out=w2754:refnum<visa-resource-name>, error out=w2753:errorcluster)  [unwired: 1 out]
                    n1670 = VISA Close(VISA resource name=w2754, error in (no error)=w2753) -> ()  [unwired: 1 out]
                  }
                }
                n1671 = local read "Normal \nRate (ul/hr)  2"() -> (w2675:dbl)
                n1672 = Concatenate Strings("set units 4 ", w2690) -> (w2686:string)
                n1673 = local read "Normal \nVolume (ul) 2"() -> (w2676:dbl)
                n1674 = Number To Decimal String(number=w2675) -> (decimal integer string=w2685:string)  [unwired: 1 in]
                n1675 = Concatenate Strings("set rate ", w2685, w2690) -> (w2683:string)
                n1676 = Number To Decimal String(number=w2676) -> (decimal integer string=w2681:string)  [unwired: 1 in]
                n1677 = Concatenate Strings("set volume ", w2681, w2690) -> (w2680:string)
              }
            }
          }
          event "Inject Pump 1": Value Change {
            n1678 = event-data() -> ()  [unwired: 1 in, 5 out]
            n1679 = case shown="True" "Inject Pump 1" {
              tunnel: w2760 -> [w2763 w2805]
              frame False {
                n1680 = local read "Write Wait"() -> (w2762:i32)
                n1681 = call-poly "VISA Configure Serial Port"("VISA resource name"=w2763) -> ("VISA resource name out"=w2767:refnum<visa-resource-name>, "error out"=w2768:errorcluster)  [unwired: 13 in]
                n1682 = Concatenate Strings("enter pump1", "\r") -> (w2765:string)
                n1683 = flat-sequence {
                  tunnel: w2768 -> [w2779]
                  tunnel: w2767 -> [w2781]
                  tunnel: [w2780] -> w2776
                  tunnel: [w2778] -> w2775
                  tunnel: w2765 -> [w2777]
                  tunnel: w2776 -> [w2784]
                  tunnel: w2775 -> [w2783]
                  tunnel: [w2784] -> w2774
                  tunnel: [w2783] -> w2773
                  tunnel: w2762 -> [w2782]
                  tunnel: [w2788] -> w2772
                  tunnel: [w2787] -> w2771
                  tunnel: w2774 -> [w2786]
                  tunnel: w2773 -> [w2785]
                  tunnel: w2772 -> [w2794]
                  tunnel: [w2794] -> w2770
                  tunnel: w2771 -> [w2793]
                  tunnel: [w2793] -> w2769
                  tunnel: w2762 -> [w2792]
                  tunnel: w2770 -> [w2798]
                  tunnel: w2769 -> [w2797]
                  frame #0 {
                    n1684 = VISA Write(VISA resource name=w2781, write buffer=w2777, error in (no error)=w2779) -> (VISA resource name out=w2780:refnum<visa-resource-name>, error out=w2778:errorcluster)  [unwired: 1 out]
                  }
                  frame #1 {
                    n1685 = Wait (ms)(milliseconds to wait=w2782) -> ()  [unwired: 1 out]
                  }
                  frame #2 {
                    n1686 = Concatenate Strings("stop ", "\r") -> (w2791:string)
                    n1687 = VISA Write(VISA resource name=w2786, write buffer=w2791, error in (no error)=w2785) -> (VISA resource name out=w2788:refnum<visa-resource-name>, error out=w2787:errorcluster)  [unwired: 1 out]
                  }
                  frame #3 {
                    n1688 = Wait (ms)(milliseconds to wait=w2792) -> ()  [unwired: 1 out]
                  }
                  frame #4 {
                    n1689 = Concatenate Strings("enter main ", "\r") -> (w2799:string)
                    n1690 = VISA Write(VISA resource name=w2798, write buffer=w2799, error in (no error)=w2797) -> (VISA resource name out=w2796:refnum<visa-resource-name>, error out=w2795:errorcluster)  [unwired: 1 out]
                    n1691 = VISA Close(VISA resource name=w2796, error in (no error)=w2795) -> ()  [unwired: 1 out]
                  }
                }
              }
              frame True {
                w2818 = "\r"
                n1692 = call-poly "VISA Configure Serial Port"("VISA resource name"=w2805) -> ("VISA resource name out"=w2807:refnum<visa-resource-name>, "error out"=w2806:errorcluster)  [unwired: 13 in]
                n1693 = local read "Write Wait"() -> (w2802:i32)
                n1694 = flat-sequence {
                  tunnel: w2806 -> [w2841]
                  tunnel: w2807 -> [w2843]
                  tunnel: [w2842] -> w2838
                  tunnel: [w2840] -> w2837
                  tunnel: w2817 -> [w2839]
                  tunnel: w2838 -> [w2846]
                  tunnel: [w2846] -> w2836
                  tunnel: w2837 -> [w2845]
                  tunnel: [w2845] -> w2835
                  tunnel: w2802 -> [w2844]
                  tunnel: [w2851] -> w2834
                  tunnel: w2814 -> [w2850]
                  tunnel: [w2847] -> w2833
                  tunnel: w2836 -> [w2849]
                  tunnel: w2835 -> [w2848]
                  tunnel: w2834 -> [w2854]
                  tunnel: [w2854] -> w2832
                  tunnel: [w2853] -> w2831
                  tunnel: w2833 -> [w2853]
                  tunnel: w2802 -> [w2852]
                  tunnel: w2832 -> [w2859]
                  tunnel: [w2858] -> w2830
                  tunnel: w2811 -> [w2857]
                  tunnel: w2831 -> [w2856]
                  tunnel: [w2855] -> w2829
                  tunnel: w2830 -> [w2862]
                  tunnel: [w2862] -> w2828
                  tunnel: [w2861] -> w2827
                  tunnel: w2829 -> [w2861]
                  tunnel: w2802 -> [w2860]
                  tunnel: w2828 -> [w2867]
                  tunnel: [w2866] -> w2826
                  tunnel: w2808 -> [w2865]
                  tunnel: w2827 -> [w2864]
                  tunnel: [w2863] -> w2825
                  tunnel: [w2870] -> w2824
                  tunnel: w2826 -> [w2870]
                  tunnel: [w2869] -> w2823
                  tunnel: w2825 -> [w2869]
                  tunnel: w2802 -> [w2868]
                  tunnel: w2824 -> [w2877]
                  tunnel: w2823 -> [w2876]
                  tunnel: [w2872] -> w2822
                  tunnel: [w2871] -> w2821
                  tunnel: w2822 -> [w2880]
                  tunnel: [w2880] -> w2820
                  tunnel: w2821 -> [w2879]
                  tunnel: [w2879] -> w2819
                  tunnel: w2802 -> [w2878]
                  tunnel: w2820 -> [w2884]
                  tunnel: w2819 -> [w2883]
                  frame #0 {
                    n1695 = VISA Write(VISA resource name=w2843, write buffer=w2839, error in (no error)=w2841) -> (VISA resource name out=w2842:refnum<visa-resource-name>, error out=w2840:errorcluster)  [unwired: 1 out]
                  }
                  frame #1 {
                    n1696 = Wait (ms)(milliseconds to wait=w2844) -> ()  [unwired: 1 out]
                  }
                  frame #2 {
                    n1697 = VISA Write(VISA resource name=w2849, write buffer=w2850, error in (no error)=w2848) -> (VISA resource name out=w2851:refnum<visa-resource-name>, error out=w2847:errorcluster)  [unwired: 1 out]
                  }
                  frame #3 {
                    n1698 = Wait (ms)(milliseconds to wait=w2852) -> ()  [unwired: 1 out]
                  }
                  frame #4 {
                    n1699 = VISA Write(VISA resource name=w2859, write buffer=w2857, error in (no error)=w2856) -> (VISA resource name out=w2858:refnum<visa-resource-name>, error out=w2855:errorcluster)  [unwired: 1 out]
                  }
                  frame #5 {
                    n1700 = Wait (ms)(milliseconds to wait=w2860) -> ()  [unwired: 1 out]
                  }
                  frame #6 {
                    n1701 = VISA Write(VISA resource name=w2867, write buffer=w2865, error in (no error)=w2864) -> (VISA resource name out=w2866:refnum<visa-resource-name>, error out=w2863:errorcluster)  [unwired: 1 out]
                  }
                  frame #7 {
                    n1702 = Wait (ms)(milliseconds to wait=w2868) -> ()  [unwired: 1 out]
                  }
                  frame #8 {
                    n1703 = Concatenate Strings("start ", "\r") -> (w2875:string)
                    n1704 = VISA Write(VISA resource name=w2877, write buffer=w2875, error in (no error)=w2876) -> (VISA resource name out=w2872:refnum<visa-resource-name>, error out=w2871:errorcluster)  [unwired: 1 out]
                  }
                  frame #9 {
                    n1705 = Wait (ms)(milliseconds to wait=w2878) -> ()  [unwired: 1 out]
                  }
                  frame #10 {
                    n1706 = Concatenate Strings("enter main ", "\r") -> (w2885:string)
                    n1707 = VISA Write(VISA resource name=w2884, write buffer=w2885, error in (no error)=w2883) -> (VISA resource name out=w2882:refnum<visa-resource-name>, error out=w2881:errorcluster)  [unwired: 1 out]
                    n1708 = VISA Close(VISA resource name=w2882, error in (no error)=w2881) -> ()  [unwired: 1 out]
                  }
                }
                n1709 = Concatenate Strings("enter pump1", w2818) -> (w2817:string)
                n1710 = local read "Normal \nRate (ul/hr)"() -> (w2803:dbl)
                n1711 = Concatenate Strings("set units 4 ", w2818) -> (w2814:string)
                n1712 = local read "Normal \nVolume (ul)"() -> (w2804:dbl)
                n1713 = Number To Decimal String(number=w2803) -> (decimal integer string=w2813:string)  [unwired: 1 in]
                n1714 = Concatenate Strings("set rate ", w2813, w2818) -> (w2811:string)
                n1715 = Number To Decimal String(number=w2804) -> (decimal integer string=w2809:string)  [unwired: 1 in]
                n1716 = Concatenate Strings("set volume ", w2809, w2818) -> (w2808:string)
              }
            }
          }
          event "Normal \nVolume (ul)": Value Change {
            n1717 = event-data() -> ()  [unwired: 1 in, 5 out]
            n1718 = call-poly "VISA Configure Serial Port"("VISA resource name"=w2903) -> ("VISA resource name out"=w2905:refnum<visa-resource-name>, "error out"=w2904:errorcluster)  [unwired: 13 in]
            n1719 = local read "Write Wait"() -> (w2888:i32)
            n1720 = Concatenate Strings("enter pump1", "\r") -> (w2907:string)
            n1721 = flat-sequence {
              tunnel: w2904 -> [w2917]
              tunnel: w2905 -> [w2919]
              tunnel: [w2918] -> w2897
              tunnel: [w2916] -> w2896
              tunnel: w2907 -> [w2915]
              tunnel: w2897 -> [w2922]
              tunnel: [w2922] -> w2895
              tunnel: w2896 -> [w2921]
              tunnel: [w2921] -> w2893
              tunnel: w2888 -> [w2920]
              tunnel: w2895 -> [w2926]
              tunnel: [w2927] -> w2894
              tunnel: w2893 -> [w2925]
              tunnel: [w2924] -> w2892
              tunnel: w2889 -> [w2923]
              tunnel: w2894 -> [w2930]
              tunnel: w2892 -> [w2929]
              tunnel: [w2930] -> w2914
              tunnel: [w2929] -> w2913
              tunnel: w2888 -> [w2928]
              tunnel: [w2935] -> w2912
              tunnel: [w2934] -> w2911
              tunnel: w2914 -> [w2933]
              tunnel: w2913 -> [w2932]
              tunnel: w2898 -> [w2931]
              tunnel: w2912 -> [w2938]
              tunnel: [w2938] -> w2910
              tunnel: w2911 -> [w2937]
              tunnel: [w2937] -> w2909
              tunnel: w2888 -> [w2936]
              tunnel: w2910 -> [w2942]
              tunnel: w2909 -> [w2941]
              frame #0 {
                n1722 = VISA Write(VISA resource name=w2919, write buffer=w2915, error in (no error)=w2917) -> (VISA resource name out=w2918:refnum<visa-resource-name>, error out=w2916:errorcluster)  [unwired: 1 out]
              }
              frame #1 {
                n1723 = Wait (ms)(milliseconds to wait=w2920) -> ()  [unwired: 1 out]
              }
              frame #2 {
                n1724 = VISA Write(VISA resource name=w2926, write buffer=w2923, error in (no error)=w2925) -> (VISA resource name out=w2927:refnum<visa-resource-name>, error out=w2924:errorcluster)  [unwired: 1 out]
              }
              frame #3 {
                n1725 = Wait (ms)(milliseconds to wait=w2928) -> ()  [unwired: 1 out]
              }
              frame #4 {
                n1726 = VISA Write(VISA resource name=w2933, write buffer=w2931, error in (no error)=w2932) -> (VISA resource name out=w2935:refnum<visa-resource-name>, error out=w2934:errorcluster)  [unwired: 1 out]
              }
              frame #5 {
                n1727 = Wait (ms)(milliseconds to wait=w2936) -> ()  [unwired: 1 out]
              }
              frame #6 {
                n1728 = Concatenate Strings("enter main ", "\r") -> (w2943:string)
                n1729 = VISA Write(VISA resource name=w2942, write buffer=w2943, error in (no error)=w2941) -> (VISA resource name out=w2940:refnum<visa-resource-name>, error out=w2939:errorcluster)  [unwired: 1 out]
                n1730 = VISA Close(VISA resource name=w2940, error in (no error)=w2939) -> ()  [unwired: 1 out]
              }
            }
            n1731 = Concatenate Strings("set units 4", "\r") -> (w2889:string)
            n1732 = Number To Decimal String(number="Normal \nVolume (ul)") -> (decimal integer string=w2900:string)  [unwired: 1 in]
            n1733 = Concatenate Strings("set volume", w2900, "\r") -> (w2898:string)
          }
          event "Normal \nRate (ul/hr)": Value Change {
            n1734 = event-data() -> ()  [unwired: 1 in, 5 out]
            n1735 = call-poly "VISA Configure Serial Port"("VISA resource name"=w2948) -> ("VISA resource name out"=w2956:refnum<visa-resource-name>, "error out"=w2955:errorcluster)  [unwired: 13 in]
            n1736 = local read "Write Wait"() -> (w2946:i32)
            n1737 = Concatenate Strings("enter pump1", "\r") -> (w2958:string)
            n1738 = flat-sequence {
              tunnel: w2955 -> [w2975]
              tunnel: w2956 -> [w2977]
              tunnel: [w2976] -> w2971
              tunnel: [w2974] -> w2970
              tunnel: w2958 -> [w2973]
              tunnel: w2971 -> [w2980]
              tunnel: [w2980] -> w2969
              tunnel: w2970 -> [w2979]
              tunnel: [w2979] -> w2968
              tunnel: w2946 -> [w2978]
              tunnel: w2969 -> [w2984]
              tunnel: [w2985] -> w2967
              tunnel: w2968 -> [w2983]
              tunnel: [w2982] -> w2966
              tunnel: w2949 -> [w2981]
              tunnel: w2967 -> [w2988]
              tunnel: w2966 -> [w2987]
              tunnel: [w2988] -> w2965
              tunnel: [w2987] -> w2964
              tunnel: w2946 -> [w2986]
              tunnel: [w2993] -> w2963
              tunnel: [w2992] -> w2962
              tunnel: w2965 -> [w2991]
              tunnel: w2964 -> [w2990]
              tunnel: w2952 -> [w2989]
              tunnel: w2963 -> [w2996]
              tunnel: [w2996] -> w2961
              tunnel: w2962 -> [w2995]
              tunnel: [w2995] -> w2960
              tunnel: w2946 -> [w2994]
              tunnel: w2961 -> [w3000]
              tunnel: w2960 -> [w2999]
              frame #0 {
                n1739 = VISA Write(VISA resource name=w2977, write buffer=w2973, error in (no error)=w2975) -> (VISA resource name out=w2976:refnum<visa-resource-name>, error out=w2974:errorcluster)  [unwired: 1 out]
              }
              frame #1 {
                n1740 = Wait (ms)(milliseconds to wait=w2978) -> ()  [unwired: 1 out]
              }
              frame #2 {
                n1741 = VISA Write(VISA resource name=w2984, write buffer=w2981, error in (no error)=w2983) -> (VISA resource name out=w2985:refnum<visa-resource-name>, error out=w2982:errorcluster)  [unwired: 1 out]
              }
              frame #3 {
                n1742 = Wait (ms)(milliseconds to wait=w2986) -> ()  [unwired: 1 out]
              }
              frame #4 {
                n1743 = VISA Write(VISA resource name=w2991, write buffer=w2989, error in (no error)=w2990) -> (VISA resource name out=w2993:refnum<visa-resource-name>, error out=w2992:errorcluster)  [unwired: 1 out]
              }
              frame #5 {
                n1744 = Wait (ms)(milliseconds to wait=w2994) -> ()  [unwired: 1 out]
              }
              frame #6 {
                n1745 = Concatenate Strings("enter main ", "\r") -> (w3001:string)
                n1746 = VISA Write(VISA resource name=w3000, write buffer=w3001, error in (no error)=w2999) -> (VISA resource name out=w2998:refnum<visa-resource-name>, error out=w2997:errorcluster)  [unwired: 1 out]
                n1747 = VISA Close(VISA resource name=w2998, error in (no error)=w2997) -> ()  [unwired: 1 out]
              }
            }
            n1748 = Concatenate Strings("set units 4", "\r") -> (w2949:string)
            n1749 = Number To Decimal String(number="Normal \nRate (ul/hr)") -> (decimal integer string=w2947:string)  [unwired: 1 in]
            n1750 = Concatenate Strings("set rate", w2947, "\r") -> (w2952:string)
          }
          event "Normal \nRate (ul/hr)  2": Value Change {
            n1751 = event-data() -> ()  [unwired: 1 in, 5 out]
            n1752 = call-poly "VISA Configure Serial Port"("VISA resource name"=w3006) -> ("VISA resource name out"=w3014:refnum<visa-resource-name>, "error out"=w3013:errorcluster)  [unwired: 13 in]
            n1753 = local read "Write Wait"() -> (w3004:i32)
            n1754 = Concatenate Strings("enter pump2", "\r") -> (w3016:string)
            n1755 = flat-sequence {
              tunnel: w3013 -> [w3033]
              tunnel: w3014 -> [w3035]
              tunnel: [w3034] -> w3029
              tunnel: [w3032] -> w3028
              tunnel: w3016 -> [w3031]
              tunnel: w3029 -> [w3038]
              tunnel: [w3038] -> w3027
              tunnel: w3028 -> [w3037]
              tunnel: [w3037] -> w3026
              tunnel: w3004 -> [w3036]
              tunnel: w3027 -> [w3042]
              tunnel: [w3043] -> w3025
              tunnel: w3026 -> [w3041]
              tunnel: [w3040] -> w3024
              tunnel: w3007 -> [w3039]
              tunnel: w3025 -> [w3046]
              tunnel: w3024 -> [w3045]
              tunnel: [w3046] -> w3023
              tunnel: [w3045] -> w3022
              tunnel: w3004 -> [w3044]
              tunnel: [w3051] -> w3021
              tunnel: [w3050] -> w3020
              tunnel: w3023 -> [w3049]
              tunnel: w3022 -> [w3048]
              tunnel: w3010 -> [w3047]
              tunnel: w3021 -> [w3054]
              tunnel: [w3054] -> w3019
              tunnel: w3020 -> [w3053]
              tunnel: [w3053] -> w3018
              tunnel: w3004 -> [w3052]
              tunnel: w3019 -> [w3058]
              tunnel: w3018 -> [w3057]
              frame #0 {
                n1756 = VISA Write(VISA resource name=w3035, write buffer=w3031, error in (no error)=w3033) -> (VISA resource name out=w3034:refnum<visa-resource-name>, error out=w3032:errorcluster)  [unwired: 1 out]
              }
              frame #1 {
                n1757 = Wait (ms)(milliseconds to wait=w3036) -> ()  [unwired: 1 out]
              }
              frame #2 {
                n1758 = VISA Write(VISA resource name=w3042, write buffer=w3039, error in (no error)=w3041) -> (VISA resource name out=w3043:refnum<visa-resource-name>, error out=w3040:errorcluster)  [unwired: 1 out]
              }
              frame #3 {
                n1759 = Wait (ms)(milliseconds to wait=w3044) -> ()  [unwired: 1 out]
              }
              frame #4 {
                n1760 = VISA Write(VISA resource name=w3049, write buffer=w3047, error in (no error)=w3048) -> (VISA resource name out=w3051:refnum<visa-resource-name>, error out=w3050:errorcluster)  [unwired: 1 out]
              }
              frame #5 {
                n1761 = Wait (ms)(milliseconds to wait=w3052) -> ()  [unwired: 1 out]
              }
              frame #6 {
                n1762 = Concatenate Strings("enter main ", "\r") -> (w3059:string)
                n1763 = VISA Write(VISA resource name=w3058, write buffer=w3059, error in (no error)=w3057) -> (VISA resource name out=w3056:refnum<visa-resource-name>, error out=w3055:errorcluster)  [unwired: 1 out]
                n1764 = VISA Close(VISA resource name=w3056, error in (no error)=w3055) -> ()  [unwired: 1 out]
              }
            }
            n1765 = Concatenate Strings("set units 4", "\r") -> (w3007:string)
            n1766 = Number To Decimal String(number="Normal \nRate (ul/hr)  2") -> (decimal integer string=w3005:string)  [unwired: 1 in]
            n1767 = Concatenate Strings("set rate", w3005, "\r") -> (w3010:string)
          }
          event "Normal \nVolume (ul) 2": Value Change {
            n1768 = event-data() -> ()  [unwired: 1 in, 5 out]
            n1769 = call-poly "VISA Configure Serial Port"("VISA resource name"=w3065) -> ("VISA resource name out"=w3069:refnum<visa-resource-name>, "error out"=w3070:errorcluster)  [unwired: 13 in]
            n1770 = local read "Write Wait"() -> (w3062:i32)
            n1771 = Concatenate Strings("enter pump2", "\r") -> (w3067:string)
            n1772 = flat-sequence {
              tunnel: w3070 -> [w3091]
              tunnel: w3069 -> [w3093]
              tunnel: [w3092] -> w3088
              tunnel: [w3090] -> w3087
              tunnel: w3067 -> [w3089]
              tunnel: w3088 -> [w3096]
              tunnel: [w3096] -> w3086
              tunnel: w3087 -> [w3095]
              tunnel: [w3095] -> w3085
              tunnel: w3062 -> [w3094]
              tunnel: w3086 -> [w3100]
              tunnel: [w3101] -> w3084
              tunnel: w3085 -> [w3099]
              tunnel: [w3098] -> w3083
              tunnel: w3076 -> [w3097]
              tunnel: w3084 -> [w3104]
              tunnel: w3083 -> [w3103]
              tunnel: [w3104] -> w3082
              tunnel: [w3103] -> w3081
              tunnel: w3062 -> [w3102]
              tunnel: [w3109] -> w3080
              tunnel: [w3108] -> w3079
              tunnel: w3082 -> [w3107]
              tunnel: w3081 -> [w3106]
              tunnel: w3073 -> [w3105]
              tunnel: w3080 -> [w3112]
              tunnel: [w3112] -> w3078
              tunnel: w3079 -> [w3111]
              tunnel: [w3111] -> w3077
              tunnel: w3062 -> [w3110]
              tunnel: w3078 -> [w3116]
              tunnel: w3077 -> [w3115]
              frame #0 {
                n1773 = VISA Write(VISA resource name=w3093, write buffer=w3089, error in (no error)=w3091) -> (VISA resource name out=w3092:refnum<visa-resource-name>, error out=w3090:errorcluster)  [unwired: 1 out]
              }
              frame #1 {
                n1774 = Wait (ms)(milliseconds to wait=w3094) -> ()  [unwired: 1 out]
              }
              frame #2 {
                n1775 = VISA Write(VISA resource name=w3100, write buffer=w3097, error in (no error)=w3099) -> (VISA resource name out=w3101:refnum<visa-resource-name>, error out=w3098:errorcluster)  [unwired: 1 out]
              }
              frame #3 {
                n1776 = Wait (ms)(milliseconds to wait=w3102) -> ()  [unwired: 1 out]
              }
              frame #4 {
                n1777 = VISA Write(VISA resource name=w3107, write buffer=w3105, error in (no error)=w3106) -> (VISA resource name out=w3109:refnum<visa-resource-name>, error out=w3108:errorcluster)  [unwired: 1 out]
              }
              frame #5 {
                n1778 = Wait (ms)(milliseconds to wait=w3110) -> ()  [unwired: 1 out]
              }
              frame #6 {
                n1779 = Concatenate Strings("enter main ", "\r") -> (w3117:string)
                n1780 = VISA Write(VISA resource name=w3116, write buffer=w3117, error in (no error)=w3115) -> (VISA resource name out=w3114:refnum<visa-resource-name>, error out=w3113:errorcluster)  [unwired: 1 out]
                n1781 = VISA Close(VISA resource name=w3114, error in (no error)=w3113) -> ()  [unwired: 1 out]
              }
            }
            n1782 = Concatenate Strings("set units 4", "\r") -> (w3076:string)
            n1783 = Number To Decimal String(number="Normal \nVolume (ul) 2") -> (decimal integer string=w3063:string)  [unwired: 1 in]
            n1784 = Concatenate Strings("set volume", w3063, "\r") -> (w3073:string)
          }
        }
        n1785 = node-c288() -> ()  [unwired: 1 in, 1 out]
      }
      n1786 = node-c288(w2449) -> ()  [unwired: 1 out]
    }
    frame Enabled {
      n1787 = node-c288(2 ("Processor")) -> (w3129:T14)  [unwired: 3 in]
      n1788 = timed-loop "Pump Control" {
        timing: w3129 -> [_]
        timing-out: [_] -> w3128
        tunnel: refnum<visa-resource-name> "COM4" ("VISA resource name") -> [w3131]
        stop <- w3130 stop-if-true
        n1789 = node-c288() -> ()  [unwired: 1 in, 1 out]
        n1790 = event shown="[0] \"Flush Sample\": Value Change" {
          selector: _ -> [_ _ _ _ _]
          dyn-events: _ -> [_ _ _ _ _]
          timeout: _ -> [_ _ _ _ _]
          tunnel: w3131 -> [w3137 _ w3211 w3249 w3254]
          tunnel: [_ w3209 _ _ _] -> w3130
          event "Flush Sample": Value Change {
            n1791 = event-data() -> ()  [unwired: 1 in, 5 out]
            n1792 = local read "Write Wait"() -> (w3151:i32)
            n1793 = flat-sequence {
              tunnel: [w3175] -> w3171
              tunnel: [w3174] -> w3170
              tunnel: "CLD" -> [w3173]
              tunnel: w3137 -> [w3172]
              tunnel: w3171 -> [w3178]
              tunnel: [w3178] -> w3169
              tunnel: w3170 -> [w3177]
              tunnel: [w3177] -> w3168
              tunnel: w3151 -> [w3176]
              tunnel: [w3183] -> w3167
              tunnel: [w3180] -> w3166
              tunnel: w3169 -> [w3182]
              tunnel: w3168 -> [w3181]
              tunnel: "MODVOL" -> [w3179]
              tunnel: w3167 -> [w3186]
              tunnel: [w3186] -> w3165
              tunnel: [w3185] -> w3164
              tunnel: w3166 -> [w3185]
              tunnel: w3151 -> [w3184]
              tunnel: w3165 -> [w3191]
              tunnel: [w3190] -> w3163
              tunnel: w3153 -> [w3189]
              tunnel: w3164 -> [w3188]
              tunnel: [w3187] -> w3162
              tunnel: w3163 -> [w3194]
              tunnel: [w3194] -> w3161
              tunnel: [w3193] -> w3160
              tunnel: w3162 -> [w3193]
              tunnel: w3151 -> [w3192]
              tunnel: w3161 -> [w3199]
              tunnel: [w3198] -> w3159
              tunnel: w3155 -> [w3197]
              tunnel: w3160 -> [w3196]
              tunnel: [w3195] -> w3158
              tunnel: [w3202] -> w3156
              tunnel: w3159 -> [w3202]
              tunnel: [w3201] -> w3157
              tunnel: w3158 -> [w3201]
              tunnel: w3151 -> [w3200]
              tunnel: w3157 -> [w3207]
              tunnel: w3156 -> [w3208]
              tunnel: [w3206] -> w3146
              tunnel: "RUN " -> [w3205]
              frame #0 {
                n1794 = call "Write to pump 2.vi"("String to write"=w3173, "VISA resource name"=w3172) -> ("error out"=w3174:errorcluster, "VISA resource name out"=w3175:refnum<visa-resource-name>)  [unwired: 8 in]
              }
              frame #1 {
                n1795 = Wait (ms)(milliseconds to wait=w3176) -> ()  [unwired: 1 out]
              }
              frame #2 {
                n1796 = call "Write to pump 2.vi"("error in (no error)"=w3181, "String to write"=w3179, "VISA resource name"=w3182) -> ("error out"=w3180:errorcluster, "VISA resource name out"=w3183:refnum<visa-resource-name>)  [unwired: 7 in]
              }
              frame #3 {
                n1797 = Wait (ms)(milliseconds to wait=w3184) -> ()  [unwired: 1 out]
              }
              frame #4 {
                n1798 = call "Write to pump 2.vi"("error in (no error)"=w3188, "String to write"=w3189, "VISA resource name"=w3191) -> ("error out"=w3187:errorcluster, "VISA resource name out"=w3190:refnum<visa-resource-name>)  [unwired: 7 in]
              }
              frame #5 {
                n1799 = Wait (ms)(milliseconds to wait=w3192) -> ()  [unwired: 1 out]
              }
              frame #6 {
                n1800 = call "Write to pump 2.vi"("error in (no error)"=w3196, "String to write"=w3197, "VISA resource name"=w3199) -> ("error out"=w3195:errorcluster, "VISA resource name out"=w3198:refnum<visa-resource-name>)  [unwired: 7 in]
              }
              frame #7 {
                n1801 = Wait (ms)(milliseconds to wait=w3200) -> ()  [unwired: 1 out]
              }
              frame #8 {
                w3204 = TRUE ("Inject Pump 3")
                n1802 = Tick Count (ms)() -> (millisecond timer value=→"Flush Sample Start Time":u32)
                n1803 = call "Write to pump 2.vi"("error in (no error)"=w3207, "String to write"=w3205, "VISA resource name"=w3208) -> ("error out"=w3206:errorcluster)  [unwired: 7 in, 1 out]
                n1804 = local write "Inject Sample"(w3204) -> ()
                "Flushing Sample" <- w3204
              }
            }
            n1805 = Number To Fractional String(number="Flush \nRate (ul/min)  3") -> (F-format string=w3139:string)  [unwired: 3 in]
            n1806 = String Subset(string=w3139, length (rest)=6 ("length (rest)")) -> (substring=w3138:string)  [unwired: 1 in]
            n1807 = Concatenate Strings("RAT", w3138, "UM") -> (w3153:string)
            n1808 = Divide(x="Flush\nVolume (ul)  3", y=1000.0) -> (x/y=w3144:dbl)
            n1809 = Number To Fractional String(number=w3144) -> (F-format string=w3143:string)  [unwired: 3 in]
            n1810 = Divide(x="Flush\nVolume (ul)  3", y="Flush \nRate (ul/min)  3") -> (x/y=w3134:dbl)
            n1811 = Multiply(x=w3134, y=60.0) -> (x*y=→"Sample flush time (s)":dbl)
            n1812 = String Subset(string=w3143, length (rest)=6 ("length (rest)")) -> (substring=w3142:string)  [unwired: 1 in]
            n1813 = Concatenate Strings("TGT", w3142) -> (w3155:string)
            "error out" <- w3146
          }
          event "Stop": Value Change {
            n1814 = event-data() -> ()  [unwired: 1 in, 5 out]
            n1815 = local read "Stop"() -> (w3209:bool)
          }
          event "Inject Sample": Value Change {
            n1816 = event-data() -> ()  [unwired: 1 in, 5 out]
            n1817 = case shown="True" "Inject Sample" {
              tunnel: w3211 -> [w3213 w3219]
              frame False {
                n1818 = call "Write to pump 2.vi"("String to write"="STP", "VISA resource name"=w3213) -> ()  [unwired: 8 in, 2 out]
              }
              frame True {
                n1819 = local read "Normal \nRate (ul/hr)  3"() -> (w3220:dbl)
                n1820 = Number To Fractional String(number=w3220) -> (F-format string=w3223:string)  [unwired: 3 in]
                n1821 = String Subset(string=w3223, length (rest)=6 ("length (rest)")) -> (substring=w3221:string)  [unwired: 1 in]
                n1822 = flat-sequence {
                  tunnel: w3219 -> [w3237]
                  tunnel: [w3236] -> w3217
                  tunnel: [w3235] -> w3215
                  tunnel: w3218 -> [w3234]
                  tunnel: w3217 -> [w3240]
                  tunnel: [w3240] -> w3216
                  tunnel: w3215 -> [w3239]
                  tunnel: [w3239] -> w3214
                  tunnel: "RUN " -> [w3243]
                  tunnel: w3216 -> [w3242]
                  tunnel: w3214 -> [w3241]
                  frame #0 {
                    n1823 = call "Write to pump 2.vi"("String to write"=w3234, "VISA resource name"=w3237) -> ("error out"=w3235:errorcluster, "VISA resource name out"=w3236:refnum<visa-resource-name>)  [unwired: 8 in]
                  }
                  frame #1 {
                    n1824 = Wait (ms)(milliseconds to wait=u32 200) -> ()  [unwired: 1 out]
                  }
                  frame #2 {
                    n1825 = call "Write to pump 2.vi"("error in (no error)"=w3241, "String to write"=w3243, "VISA resource name"=w3242) -> ()  [unwired: 7 in, 2 out]
                  }
                }
                n1826 = Concatenate Strings("RAT", w3221, "UH" ("string")) -> ()  [unwired: 1 out]
                n1827 = local read "Normal \nVolume (ul) 3"() -> (w3229:dbl)
                n1828 = Divide(x=w3229, y=1000.0) -> (x/y=w3224:dbl)
                n1829 = Number To Fractional String(number=w3224) -> (F-format string=w3227:string)  [unwired: 3 in]
                n1830 = String Subset(string=w3227, length (rest)=6 ("length (rest)")) -> (substring=w3225:string)  [unwired: 1 in]
                n1831 = Concatenate Strings("TGT", w3225) -> (w3218:string)
              }
            }
          }
          event "Normal \nRate (ul/hr)  3": Value Change {
            n1832 = event-data() -> ()  [unwired: 1 in, 5 out]
            n1833 = Number To Fractional String(number="Normal \nRate (ul/hr)  3") -> (F-format string=w3247:string)  [unwired: 3 in]
            n1834 = String Subset(string=w3247, length (rest)=6 ("length (rest)")) -> (substring=w3245:string)  [unwired: 1 in]
            n1835 = Concatenate Strings("RAT", w3245, "UH") -> (w3248:string)
            n1836 = call "Write to pump 2.vi"("String to write"=w3248, "VISA resource name"=w3249) -> ()  [unwired: 8 in, 2 out]
          }
          event "Clear Volume": Value Change {
            n1837 = event-data() -> ()  [unwired: 1 in, 5 out]
            n1838 = Divide(x="Normal \nVolume (ul) 3", y=1000.0) -> (x/y=w3267:dbl)
            n1839 = Number To Fractional String(number=w3267) -> (F-format string=w3270:string)  [unwired: 3 in]
            n1840 = String Subset(string=w3270, length (rest)=6 ("length (rest)")) -> (substring=w3268:string)  [unwired: 1 in]
            n1841 = flat-sequence {
              tunnel: [w3277] -> w3265
              tunnel: [w3276] -> w3264
              tunnel: w3254 -> [w3275]
              tunnel: w3253 -> [w3274]
              tunnel: [w3279] -> w3262
              tunnel: [w3278] -> w3263
              tunnel: w3259 -> [w3280]
              tunnel: w3265 -> [w3279]
              tunnel: w3264 -> [w3278]
              tunnel: w3263 -> [w3284]
              tunnel: w3262 -> [w3285]
              tunnel: [w3283] -> _
              tunnel: [w3282] -> _
              tunnel: w3252 -> [w3281]
              frame #0 {
                n1842 = call "Write to pump 2.vi"("String to write"=w3274, "VISA resource name"=w3275) -> ("error out"=w3276:errorcluster, "VISA resource name out"=w3277:refnum<visa-resource-name>)  [unwired: 8 in]
              }
              frame #1 {
                n1843 = Wait (ms)(milliseconds to wait=w3280) -> ()  [unwired: 1 out]
              }
              frame #2 {
                n1844 = call "Write to pump 2.vi"("error in (no error)"=w3284, "String to write"=w3281, "VISA resource name"=w3285) -> ("error out"=w3282:errorcluster, "VISA resource name out"=w3283:refnum<visa-resource-name>)  [unwired: 7 in]
              }
            }
            n1845 = local read "Write Wait"() -> (w3259:i32)
            n1846 = Concatenate Strings("TGT", w3268) -> (w3253:string)
            n1847 = local read "Normal \nRate (ul/hr)  3"() -> (w3255:dbl)
            n1848 = local write "Clear Volume"(FALSE ("Clear Volume")) -> ()
            n1849 = Number To Fractional String(number=w3255) -> (F-format string=w3258:string)  [unwired: 3 in]
            n1850 = String Subset(string=w3258, length (rest)=6 ("length (rest)")) -> (substring=w3256:string)  [unwired: 1 in]
            n1851 = Concatenate Strings("RAT", w3256, "UH" ("string")) -> (w3252:string)
          }
        }
        n1852 = node-c288() -> ()  [unwired: 1 in, 1 out]
      }
      n1853 = node-c288(w3128) -> ()  [unwired: 1 out]
    }
  }
  n1854 = node-c288() -> (w90:T14)  [unwired: 4 in]
  n1855 = timed-loop {
    timing: w90 -> [_]
    timing-out: [_] -> w89
    stop <- w3292 stop-if-true
    n1856 = node-c288() -> ()  [unwired: 1 in, 1 out]
    n1857 = event shown="[1] \"Stop\": Value Change" {
      selector: _ -> [_ _]
      dyn-events: _ -> [_ _]
      timeout: _ -> [_ _]
      tunnel: [_ w3293] -> w3292
      event Timeout {
        n1858 = event-data() -> ()  [unwired: 1 in, 2 out]
      }
      event "Stop": Value Change {
        n1859 = event-data() -> ()  [unwired: 1 in, 4 out]
        n1860 = flat-sequence {
          tunnel: ["Stop"] -> w3293
          frame #0 {
            w3294 = FALSE ("Force Feedback")
            n1861 = local write "Force Feedback 1"(w3294) -> ()
            n1862 = local write "Force Feedback 2"(w3294) -> ()
            n1863 = property on="Cancel dwell" class="Bool (strict)"("Val(Sgnl)"=TRUE ("Value (Signaling)")) -> ()  [unwired: 2 in, 2 out]
          }
          frame #1 {
            w3296 = FALSE
            n1864 = local write "Raster scanning..."(w3296) -> ()
            n1865 = local write "Cancel dwell"(w3296) -> ()
            n1866 = local write "Stage moving"(w3296) -> ()
            n1867 = local write "Saving Move"(w3296) -> ()
          }
        }
      }
    }
    n1868 = node-c288() -> ()  [unwired: 1 in, 1 out]
  }
  n1869 = case shown="True" w80 {
    tunnel: w85 -> [_ w3302]
    tunnel: w84 -> [_ w3301]
    tunnel: w83 -> [_ w3300]
    frame False {
    }
    frame True {
      w3304 = T25 3 items=["no dialog", "OK message", "continue or stop message", "OK message + warnings", "continue/stop + warnings"] ("type of dialog (OK msg:1)")
      w3303 = T25 3 items=["no dialog", "OK message", "continue or stop message", "OK message + warnings", "continue/stop + warnings"] ("type of dialog (OK msg:1)")
      n1870 = call <vilib>:"DAQmx Clear Task.vi"("task in"=w3302, "error in"=w3300) -> ("error out"=w3305:errorcluster)  [unwired: 13 in]
      n1871 = call <vilib>:"DAQmx Clear Task.vi"("task in"=w3301) -> ("error out"=w3306:errorcluster)  [unwired: 14 in]
      n1872 = call <vilib>:"Simple Error Handler.vi"("type of dialog (OK msg:1)"=w3304, "error in (no error)"=w3305) -> ()  [unwired: 3 in, 5 out]
      n1873 = call <vilib>:"Simple Error Handler.vi"("type of dialog (OK msg:1)"=w3303, "error in (no error)"=w3306) -> ()  [unwired: 3 in, 5 out]
    }
  }
  n1874 = case shown="\"Raster scan\"" "?" {
    frame "Force Feedback", Default {
    }
    frame "Raster scan" {
    }
  }
  n1875 = node-c288(w89) -> ()  [unwired: 1 out]
  n1876 = node-c288(w92) -> ()  [unwired: 1 out]
  n1877 = local write "Pause Mouse/Mirror Connection"(FALSE ("Pause Mouse/Mirror Connection")) -> ()
  n1878 = local write "Stop"(FALSE ("Stop all")) -> ()
  "CoordinatesMousePressed" <- T6 {"Horizontal"=0, "Vertical"=0} ("Coords when pressed")
  "Deflection" <- T6 {"Horizontal"=0, "Vertical"=0} ("Coords when pressed")
